vi "PAS RI Retrieval with LABVIEW.vi"() -> ()   [LabVIEW 2013]
uses:
  BaesDataTypeDefinition.ctl
  ReadBaesDataTypeDefinition.ctl
  ParticleDistributionData.ctl
  GeneralDataForRIRetrieval.ctl
  <vilib>/Native 3D Graph/xcontrol/3DPC_SurfacePlot.xctl
  <vilib>/Native 3D Graph/classes/Surface/Surface.lvclass
  RIandRIMCResults.ctl
  <vilib>/gmath/NumericalOptimization/stopping criteria.ctl
  <vilib>/Analysis/1siggen.llb/Ramp Pattern by Samples.vi
  <vilib>/gmath/NumericalOptimization/Conjugate Gradient.vi
  <vilib>/Utility/file.llb/Write To Spreadsheet File (string).vi
  <vilib>/Analysis/Matrix/Numeric/Conversions/Matrix To Array - RM.vi
  <vilib>/gmath/statdist.llb/Normal Inverse CDF.vi
  <vilib>/imath/engines/lvmath2/RunTimeEngine/ErrorHandling/NIMS_Finalize Error.vi
  <vilib>/imath/engines/lvmath2/RunTimeEngine/RangeToken/NIMS_Range_R2 - Float.vi
  <instcachedir>/0/NIMS_Range_R2 - Float_E19924E36A3948A4B33043226480F83C.lvgen/NIMS_Range_R2 - Float_E19924E36A3948A4B33043226480F83C_000.vi
  <vilib>/imath/engines/lvmath2/RunTimeEngine/NodeEndStatement/NIMS_NodeEndStatement_Output.vi
  <instcachedir>/0/NIMS_NodeEndStatement_Output_53EC0D466D134D7ABD903AC30B43404B.lvgen/NIMS_NodeEndStatement_Output_53EC0D466D134D7ABD903AC30B43404B_002.vi
  <vilib>/imath/engines/lvmath2/RunTimeEngine/CommandStatement/MC_CommandStatement_break.vi
  <vilib>/imath/engines/lvmath2/RunTimeSupport/NIMS_Error if Not Equal.vi
  <instcachedir>/0/NIMS_Error if Not Equal_902F5D2649E64F5087A1EF57C55C58AB.lvgen/NIMS_Error if Not Equal_902F5D2649E64F5087A1EF57C55C58AB_000.vi
  <vilib>/imath/engines/lvmath2/RunTimeEngine/IndexRead/NIMS M($,S).vi
  <instcachedir>/0/NIMS M($,S)_3E5749BBB62E49528D4765A77F1F6D98.lvgen/NIMS M($,S)_3E5749BBB62E49528D4765A77F1F6D98_000.vi
  <vilib>/imath/engines/lvmath2/RunTimeEngine/RowToken/NIMS_RowToken_M_CV.vi
  <instcachedir>/0/NIMS_RowToken_M_CV_4FFFB80A1A2C4A06BEF1E2564C6BAFA4.lvgen/NIMS_RowToken_M_CV_4FFFB80A1A2C4A06BEF1E2564C6BAFA4_000.vi
  <vilib>/imath/engines/lvmath2/RunTimeEngine/ErrorHandling/NIMS_Create Error From Enums.vi
  <vilib>/gmath/NI_Gmath.lvlib
  <vilib>/Analysis/Matrix/NI_Matrix.lvlib
  <vilib>/Analysis/NI_AALBase.lvlib
panel:
  in  "autoscale":bool
  in  "Correct SMPS sizes to selected Sizes":bool
  out "Peak Center":dbl[](array[numeric])=[215.23700286959917, 239.46777469280113, 266.53712087613405, 296.56972011152817, 329.9933867048781, 354.3213922159785, 380.24064147372457, 407.9273850466716, 436.86507564817134]
  in  "method":i32(ring)=3 items=["nearest", "linear", "spline", "cubic Hermite", "Lagrange"]
  out "yi out":dbl[][](array[numeric])=[[0.0, 0.0, 0.0, 0.0, 0.0, 0.0, 0.0, 0.0, 0.0], [0.0, 0.0, 0.0, 0.0, 0.0, 0.0, 0.0, 0.0, 0.0], [0.0, 0.0, 0.0, 0.0, 0.0, 0.0, 0.0, 0.0, 0.0], [0.0, 0.0, 0.0, 0.0, 0.0, 0.0, 0.0, 0.0, 0.0], [0.0, 0.0, 0.0, 0.0, 0.0, 0.0, 0.0, 0.0, 0.0], [0.0, 0.0, 0.0, 0.0, 0.0, 0.0, 0.0, 0.0, 0.0], [0.0, 0.0, 0.0, 0.0, 0.0, 0.0, 0.0, 0.0, 0.0], [0.0, 0.0, 0.0, 0.0, 0.0, 0.0, 0.0, 0.0, 0.0], [0.0, 0.0, 0.0, 0.0, 0.0, 0.0, 0.0, 0.0, 0.0], [0.0, 0.0, 0.0, 0.0, 0.0, 0.0, 0.0, 0.0, 0.0], [0.0, 0.0, 0.0, 0.0, 0.0, 0.0, 0.0, 0.0, 0.0], [0.0, 0.0, 0.0, 0.0, 0.0, 0.0, 0.0, 0.0, 0.0], [0.0, 0.0, 0.0, 0.0, 0.0, 0.0, 0.0, 0.0, 0.0], [0.0, 0.0, 0.0, 0.0, 0.0, 0.0, 0.0, 0.0, 0.0], [0.0, 0.0, 0.0, 0.0, 0.0, 0.0, 0.0, 0.0, 0.0], [0.0, 0.0, 0.0, 0.0, 0.0, 0.0, 0.0, 0.0, 0.0], [0.002995533043634161, 0.0, 0.0, 0.0, 0.0, 0.0, 0.0, 0.0, 0.0], [0.025840856539342556, 0.0, 0.0, 0.0, 0.0, 0.0, 0.0, 0.0, 0.0], [0.09627433030958367, 0.0, 0.0, 0.0, 0.0, 0.0, 0.0, 0.0, 0.0], [0.20114413818462407, 0.003679405258454903, 0.0, 0.0, 0.0, 0.0, 0.0, 0.0, 0.0], [0.24542760207823705, 0.030110785948579594, 0.0, 0.0, 0.0, 0.0, 0.0, 0.0, 0.0], [0.19935011876678227, 0.10676097365384078, 0.0, 0.0, 0.0, 0.0, 0.0, 0.0, 0.0], [0.10027077337218139, 0.21292413302969826, 0.0033748243651170722, 0.0, 0.0, 0.0, 0.0, 0.0, 0.0], [0.02900603131815543, 0.252436330373865, 0.02890039600275283, 0.0, 0.0, 0.0, 0.0, 0.0, 0.0], [0.0039798778324419744, 0.1962993842174311, 0.10425475468568692, 0.0, 0.0, 0.0, 0.0, 0.0, 0.0], [0.0, 0.09510810120556674, 0.2127509720448336, 0.003204303022032701, 0.0, 0.0, 0.0, 0.0, 0.0], [0.0, 0.026788275767934952, 0.25443516550640577, 0.028222420464123123, 0.0, 0.0, 0.0, 0.0, 0.0], [0.0, 0.0036138798422305257, 0.20572070395413536, 0.10336691645150534, 0.0, 0.0, 0.0, 0.0, 0.0], [0.0, 0.0, 0.10385751888143922, 0.21356874773842194, 0.003345015757771727, 0.0, 0.0, 0.0, 0.0], [0.0, 0.0, 0.03184137129301377, 0.25514474611865134, 0.02938228217938827, 0.0, 0.0, 0.0, 0.0], [0.0014956304497509467, 0.0, 0.005324689051489316, 0.21179320089555217, 0.10705199934528585, 0.003308736710887511, 0.0, 0.0, 0.0], [0.006181204689297098, 0.0, 0.0, 0.10947088728935564, 0.21880478513266646, 0.029404152563977024, 0.0, 0.0, 0.0], [0.014779079751943505, 0.0, 0.0, 0.0351443521735081, 0.2573967125709004, 0.10811744003531051, 0.004055473967709127, 0.0, 0.0], [0.021873123606276416, 0.0, 0.0, 0.00645421284142625, 0.21311979554910082, 0.21949012820871305, 0.03249660231234976, 0.0, 0.0], [0.020938671287516166, 0.002941447778294588, 0.0, 0.0005784696243201418, 0.11000745576713801, 0.2570127905092043, 0.11420156491259865, 0.004251138588627886, 0.0], [0.014150903231161319, 0.00918486371676828, 0.0, 0.0, 0.036185400505208645, 0.21598258772382448, 0.22683349675845424, 0.03241034304426709, 0.0], [0.005998151011193356, 0.016563944732687075, 0.0, 0.0, 0.007021566470141746, 0.11238428494392888, 0.25641274621663857, 0.11266793086437756, 0.004147715999403451], [0.0015120995486811858, 0.017797923247623602, 0.001492807625783663, 0.0, 0.0007094205616598339, 0.037396339870968194, 0.21111602466052512, 0.22428037538775147, 0.031085439808444255], [0.0, 0.01329593538708705, 0.005201029958243257, 0.0, 0.0, 0.007536234728094553, 0.10787117985635983, 0.25568882442612334, 0.11065902188610582], [0.0, 0.00635541490586478, 0.010415971194231972, 0.0, 0.0, 0.0008190951722994508, 0.03536648135652447, 0.21469636352155314, 0.2221123992215679], [0.0010729774499575713, 0.0019363898629268694, 0.01277891881575932, 0.0006807013617405569, 0.0, 0.0, 0.007025068509258474, 0.10969810395513567, 0.25508407775997943], [0.002057300309839938, 0.0, 0.010740838502774176, 0.002649342768284491, 0.0, 0.0, 0.0007440549395453882, 0.03615143628832095, 0.216785934587122], [0.002474950875894475, 0.0, 0.006120821318984597, 0.006052131853820764, 0.0, 0.0, 0.0, 0.007394514918229318, 0.11122539130067338], [0.002060729815382503, 0.0, 0.002286068305636173, 0.008519468407529212, 0.0, 0.0, 0.0, 0.0008550654797584019, 0.03853326504170029], [0.0011159165281229126, 0.0009250356514019637, 0.0005031484937129974, 0.007827186354841077, 0.0010483084611445424, 0.0, 0.0, 0.0, 0.008221211137071305], [0.0, 0.0013182032160797494, 0.0, 0.0048751624944381525, 0.002846930380238516, 0.0, 0.0, 0.0, 0.0009934611660537788], [0.0, 0.0011832812074649155, 0.0, 0.0019419202748162476, 0.004454066932151218, 0.0, 0.0, 0.0, 0.0], [0.0, 0.0007762909961994142, 0.0, 0.0005058298656327597, 0.004488441198541657, 0.001576949269729668, 0.0, 0.0, 0.0], [0.0, 0.0, 0.0, 0.0, 0.0029347814148206284, 0.002346089545272472, 0.0, 0.0, 0.0], [0.0, 0.0, 0.0, 0.0, 0.0012030377738417415, 0.00231674366991226, 0.0007291026037730795, 0.0, 0.0], [0.0, 0.0, 0.0, 0.0, 0.0, 0.0015886617028698508, 0.0011333656105798114, 0.0, 0.0], [0.0, 0.0, 0.0, 0.0, 0.0, 0.0007197653450079487, 0.0011589853888717718, 0.0, 0.0], [0.0, 0.0, 0.0, 0.0, 0.0, 0.0, 0.0008558529068117928, 0.0005237679257223164, 0.0], [0.0, 0.0, 0.0, 0.0, 0.0, 0.0, 0.0, 0.0007042968505584731, 0.0], [0.0, 0.0, 0.0, 0.0, 0.0, 0.0, 0.0, 0.000677838749574469, 0.0], [0.0, 0.0, 0.0, 0.0, 0.0, 0.0, 0.0, 0.0, 0.000518938219565122], [0.0, 0.0, 0.0, 0.0, 0.0, 0.0, 0.0, 0.0, 0.0006331438723132111]]
  out "SMPS":T1(graph)=[{"Ramp Pattern"=[105.5, 109.4, 113.4, 117.6, 121.9, 126.3, 131.0, 135.8, 140.7, 145.9, 151.2, 156.8, 162.5, 168.5, 174.7, 181.1, 187.7, 194.6, 201.7, 209.1, 216.7, 224.7, 232.9, 241.4, 250.3, 259.5, 269.0, 278.8, 289.0, 299.6, 310.6, 322.0, 333.8, 346.0, 358.7, 371.8, 385.4, 399.5, 414.2, 429.4, 445.1, 461.4, 478.3, 495.8, 514.0, 532.8, 552.3, 572.5, 593.5, 615.3, 637.8, 661.2, 685.4, 710.5, 736.5, 763.5, 791.5], "Extinction"=[0.0, 0.0, 0.0, 0.0, 0.0, 0.0, 0.0, 0.0, 0.0, 0.0, 0.0, 0.0, 0.0, 0.0, 0.0, 0.0, 0.0, 0.0, 0.0, 0.0, 0.0, 0.0, 0.0, 0.0, 0.0, 0.0, 0.0, 0.0, 0.0, 0.0, 0.0, 0.0, 0.0, 0.0, 0.0, 0.0, 0.004147715999403451, 0.031085439808444255, 0.11065902188610582, 0.2221123992215679, 0.25508407775997943, 0.216785934587122, 0.11122539130067338, 0.03853326504170029, 0.008221211137071305, 0.0009934611660537788, 0.0, 0.0, 0.0, 0.0, 0.0, 0.0, 0.0, 0.0, 0.0, 0.000518938219565122, 0.0006331438723132111]}, {"Ramp Pattern"=[105.5, 109.4, 113.4, 117.6, 121.9, 126.3, 131.0, 135.8, 140.7, 145.9, 151.2, 156.8, 162.5, 168.5, 174.7, 181.1, 187.7, 194.6, 201.7, 209.1, 216.7, 224.7, 232.9, 241.4, 250.3, 259.5, 269.0, 278.8, 289.0, 299.6, 310.6, 322.0, 333.8, 346.0, 358.7, 371.8, 385.4, 399.5, 414.2, 429.4, 445.1, 461.4, 478.3, 495.8, 514.0, 532.8, 552.3, 572.5, 593.5, 615.3, 637.8, 661.2, 685.4, 710.5, 736.5, 763.5, 791.5], "Extinction"=[0.0, 0.0, 0.0, 0.0, 0.0, 0.0, 0.0, 0.0, 0.0, 0.0, 0.0, 0.0, 0.0, 0.0, 0.0, 0.0, 0.0, 0.0, 0.0, 0.0, 0.0, 0.0, 0.0, 0.0, 0.0, 0.0, 0.0, 0.0, 0.0, 0.0, 0.0, 0.0, 0.0, 0.0, 0.0, 0.000717254, 0.0123831, 0.0638696, 0.166954, 0.256206, 0.250783, 0.158589, 0.0675111, 0.0180047, 0.00271755, 0.000182617, 0.0, 0.0, 0.0, 0.0, 0.0, 1.197e-05, 6.86901e-05, 0.000249565, 0.000468067, 0.00056712, 0.000716313]}]
  in  "ShiftSMPStoSizes":bool
  out "Size Distribution":T1(graph)=[{"Ramp Pattern"=[105.5, 109.4, 113.4, 117.6, 121.9, 126.3, 131.0, 135.8, 140.7, 145.9, 151.2, 156.8, 162.5, 168.5, 174.7, 181.1, 187.7, 194.6, 201.7, 209.1, 216.7, 224.7, 232.9, 241.4, 250.3, 259.5, 269.0, 278.8, 289.0, 299.6, 310.6, 322.0, 333.8, 346.0, 358.7, 371.8, 385.4, 399.5, 414.2, 429.4, 445.1, 461.4, 478.3, 495.8, 514.0, 532.8, 552.3, 572.5, 593.5, 615.3, 637.8, 661.2, 685.4, 710.5, 736.5, 763.5, 791.5], "Extinction"=[0.0, 0.0, 0.0, 0.0, 0.0, 0.0, 0.0, 0.0, 0.0, 0.0, 0.0, 0.0, 0.0, 0.0, 0.0, 0.0, 0.00469758, 0.0354227, 0.116984, 0.216414, 0.247187, 0.179631, 0.0803359, 0.0204142, 0.00221516, 0.0, 0.0, 0.0, 0.0, 0.000247208, 0.00208403, 0.00771025, 0.0165625, 0.0223051, 0.0201811, 0.012183, 0.00466618, 0.00104529, 0.000166113, 0.000427922, 0.00128502, 0.00219655, 0.00249145, 0.00187776, 0.00091843, 0.000292032, 5.29153e-05, 4.6626e-06, 0.0, 0.0, 0.0, 0.0, 0.0, 0.0, 0.0, 0.0, 0.0]}, {"Ramp Pattern"=[105.5, 109.4, 113.4, 117.6, 121.9, 126.3, 131.0, 135.8, 140.7, 145.9, 151.2, 156.8, 162.5, 168.5, 174.7, 181.1, 187.7, 194.6, 201.7, 209.1, 216.7, 224.7, 232.9, 241.4, 250.3, 259.5, 269.0, 278.8, 289.0, 299.6, 310.6, 322.0, 333.8, 346.0, 358.7, 371.8, 385.4, 399.5, 414.2, 429.4, 445.1, 461.4, 478.3, 495.8, 514.0, 532.8, 552.3, 572.5, 593.5, 615.3, 637.8, 661.2, 685.4, 710.5, 736.5, 763.5, 791.5], "Extinction"=[0.0, 0.0, 0.0, 0.0, 0.0, 0.0, 0.0, 0.0, 0.0, 0.0, 0.0, 0.0, 0.0, 0.0, 0.0, 0.0, 0.0, 0.0, 0.0, 0.00519856, 0.0384325, 0.123532, 0.224073, 0.253164, 0.179467, 0.0797032, 0.0202966, 0.00230883, 2.78494e-05, 0.0, 0.0, 0.0, 1.449e-05, 0.000603145, 0.00368011, 0.0104387, 0.0170704, 0.0177851, 0.0120367, 0.00534763, 0.0015055, 0.000251878, 0.000139253, 0.000474877, 0.00100593, 0.00133239, 0.00112993, 0.000690039, 0.000227701, 5.64159e-05, 7.13036e-06, 4.80125e-07, 0.0, 0.0, 0.0, 0.0, 0.0]}, {"Ramp Pattern"=[105.5, 109.4, 113.4, 117.6, 121.9, 126.3, 131.0, 135.8, 140.7, 145.9, 151.2, 156.8, 162.5, 168.5, 174.7, 181.1, 187.7, 194.6, 201.7, 209.1, 216.7, 224.7, 232.9, 241.4, 250.3, 259.5, 269.0, 278.8, 289.0, 299.6, 310.6, 322.0, 333.8, 346.0, 358.7, 371.8, 385.4, 399.5, 414.2, 429.4, 445.1, 461.4, 478.3, 495.8, 514.0, 532.8, 552.3, 572.5, 593.5, 615.3, 637.8, 661.2, 685.4, 710.5, 736.5, 763.5, 791.5], "Extinction"=[0.0, 0.0, 0.0, 0.0, 0.0, 0.0, 0.0, 0.0, 0.0, 0.0, 0.0, 0.0, 0.0, 0.0, 0.0, 0.0, 0.0, 0.0, 0.0, 0.0, 0.0, 0.0, 0.00571825, 0.0414768, 0.129134, 0.230099, 0.256094, 0.180426, 0.0808733, 0.0216409, 0.00294192, 0.000130313, 0.0, 0.0, 0.0, 0.0, 0.000309949, 0.00212484, 0.00641526, 0.0113124, 0.0128925, 0.00963301, 0.00497583, 0.00165198, 0.00031264, 4.70524e-05, 0.00012066, 0.000336979, 0.000449342, 0.00045116, 0.000267214, 0.000124042, 3.43184e-05, 6.32589e-06, 6.1806e-07, 0.0, 0.0]}, {"Ramp Pattern"=[105.5, 109.4, 113.4, 117.6, 121.9, 126.3, 131.0, 135.8, 140.7, 145.9, 151.2, 156.8, 162.5, 168.5, 174.7, 181.1, 187.7, 194.6, 201.7, 209.1, 216.7, 224.7, 232.9, 241.4, 250.3, 259.5, 269.0, 278.8, 289.0, 299.6, 310.6, 322.0, 333.8, 346.0, 358.7, 371.8, 385.4, 399.5, 414.2, 429.4, 445.1, 461.4, 478.3, 495.8, 514.0, 532.8, 552.3, 572.5, 593.5, 615.3, 637.8, 661.2, 685.4, 710.5, 736.5, 763.5, 791.5], "Extinction"=[0.0, 0.0, 0.0, 0.0, 0.0, 0.0, 0.0, 0.0, 0.0, 0.0, 0.0, 0.0, 0.0, 0.0, 0.0, 0.0, 0.0, 0.0, 0.0, 0.0, 0.0, 0.0, 0.0, 0.0, 0.0, 0.00632071, 0.0446845, 0.135704, 0.236113, 0.25755, 0.180077, 0.0805602, 0.0218917, 0.00313629, 0.000172749, 0.0, 0.0, 0.0, 0.0, 0.000146105, 0.00109424, 0.00357516, 0.00701794, 0.00877109, 0.00708357, 0.00381669, 0.00131952, 0.000297028, 3.13476e-05, 2.27371e-05, 6.57026e-05, 0.000128581, 0.000145168, 0.00012623, 8.554e-05, 3.72251e-05, 2.65028e-05]}, {"Ramp Pattern"=[105.5, 109.4, 113.4, 117.6, 121.9, 126.3, 131.0, 135.8, 140.7, 145.9, 151.2, 156.8, 162.5, 168.5, 174.7, 181.1, 187.7, 194.6, 201.7, 209.1, 216.7, 224.7, 232.9, 241.4, 250.3, 259.5, 269.0, 278.8, 289.0, 299.6, 310.6, 322.0, 333.8, 346.0, 358.7, 371.8, 385.4, 399.5, 414.2, 429.4, 445.1, 461.4, 478.3, 495.8, 514.0, 532.8, 552.3, 572.5, 593.5, 615.3, 637.8, 661.2, 685.4, 710.5, 736.5, 763.5, 791.5], "Extinction"=[0.0, 0.0, 0.0, 0.0, 0.0, 0.0, 0.0, 0.0, 0.0, 0.0, 0.0, 0.0, 0.0, 0.0, 0.0, 0.0, 0.0, 0.0, 0.0, 0.0, 0.0, 0.0, 0.0, 0.0, 0.0, 0.0, 0.0, 0.0, 0.00691542, 0.0475552, 0.141845, 0.242118, 0.259618, 0.178404, 0.0799987, 0.0221613, 0.00339671, 0.000219474, 0.0, 0.0, 0.0, 0.0, 2.69179e-05, 0.000353007, 0.00153723, 0.00346079, 0.0046555, 0.00430387, 0.00217813, 0.000845627, 0.000191511, 2.95911e-05, 4.40706e-06, 1.46487e-05, 4.0603e-05, 5.6006e-05, 7.02252e-05]}, {"Ramp Pattern"=[105.5, 109.4, 113.4, 117.6, 121.9, 126.3, 131.0, 135.8, 140.7, 145.9, 151.2, 156.8, 162.5, 168.5, 174.7, 181.1, 187.7, 194.6, 201.7, 209.1, 216.7, 224.7, 232.9, 241.4, 250.3, 259.5, 269.0, 278.8, 289.0, 299.6, 310.6, 322.0, 333.8, 346.0, 358.7, 371.8, 385.4, 399.5, 414.2, 429.4, 445.1, 461.4, 478.3, 495.8, 514.0, 532.8, 552.3, 572.5, 593.5, 615.3, 637.8, 661.2, 685.4, 710.5, 736.5, 763.5, 791.5], "Extinction"=[0.0, 0.0, 0.0, 0.0, 0.0, 0.0, 0.0, 0.0, 0.0, 0.0, 0.0, 0.0, 0.0, 0.0, 0.0, 0.0, 0.0, 0.0, 0.0, 0.0, 0.0, 0.0, 0.0, 0.0, 0.0, 0.0, 0.0, 0.0, 0.0, 0.0, 0.00736473, 0.0497393, 0.146587, 0.244445, 0.259093, 0.17829, 0.0792691, 0.0221239, 0.00350155, 0.000239507, 0.0, 0.0, 0.0, 0.0, 0.0, 0.000136757, 0.000762018, 0.00196813, 0.00242627, 0.00218637, 0.0012033, 0.000506553, 0.000129976, 2.46205e-05, 2.20754e-06, 0.0, 0.0]}, {"Ramp Pattern"=[105.5, 109.4, 113.4, 117.6, 121.9, 126.3, 131.0, 135.8, 140.7, 145.9, 151.2, 156.8, 162.5, 168.5, 174.7, 181.1, 187.7, 194.6, 201.7, 209.1, 216.7, 224.7, 232.9, 241.4, 250.3, 259.5, 269.0, 278.8, 289.0, 299.6, 310.6, 322.0, 333.8, 346.0, 358.7, 371.8, 385.4, 399.5, 414.2, 429.4, 445.1, 461.4, 478.3, 495.8, 514.0, 532.8, 552.3, 572.5, 593.5, 615.3, 637.8, 661.2, 685.4, 710.5, 736.5, 763.5, 791.5], "Extinction"=[0.0, 0.0, 0.0, 0.0, 0.0, 0.0, 0.0, 0.0, 0.0, 0.0, 0.0, 0.0, 0.0, 0.0, 0.0, 0.0, 0.0, 0.0, 0.0, 0.0, 0.0, 0.0, 0.0, 0.0, 0.0, 0.0, 0.0, 0.0, 0.0, 0.0, 0.0, 0.000111786, 0.00841072, 0.0527736, 0.151025, 0.248521, 0.257332, 0.174677, 0.0773732, 0.021334, 0.00336166, 0.000228943, 0.0, 0.0, 0.0, 0.0, 0.0, 7.68722e-05, 0.000371516, 0.000899449, 0.00118202, 0.00112913, 0.000682538, 0.000358916, 0.00012183, 2.28142e-05, 5.76992e-06]}, {"Ramp Pattern"=[105.5, 109.4, 113.4, 117.6, 121.9, 126.3, 131.0, 135.8, 140.7, 145.9, 151.2, 156.8, 162.5, 168.5, 174.7, 181.1, 187.7, 194.6, 201.7, 209.1, 216.7, 224.7, 232.9, 241.4, 250.3, 259.5, 269.0, 278.8, 289.0, 299.6, 310.6, 322.0, 333.8, 346.0, 358.7, 371.8, 385.4, 399.5, 414.2, 429.4, 445.1, 461.4, 478.3, 495.8, 514.0, 532.8, 552.3, 572.5, 593.5, 615.3, 637.8, 661.2, 685.4, 710.5, 736.5, 763.5, 791.5], "Extinction"=[0.0, 0.0, 0.0, 0.0, 0.0, 0.0, 0.0, 0.0, 0.0, 0.0, 0.0, 0.0, 0.0, 0.0, 0.0, 0.0, 0.0, 0.0, 0.0, 0.0, 0.0, 0.0, 0.0, 0.0, 0.0, 0.0, 0.0, 0.0, 0.0, 0.0, 0.0, 0.0, 0.0, 0.00034567, 0.00996877, 0.0572363, 0.156117, 0.250468, 0.256357, 0.169838, 0.0734243, 0.0196929, 0.00313418, 0.000220524, 0.0, 0.0, 0.0, 0.0, 0.0, 3.08466e-05, 0.000159988, 0.000411927, 0.000591209, 0.000742169, 0.000598205, 0.000349683, 0.000313284]}, {"Ramp Pattern"=[105.5, 109.4, 113.4, 117.6, 121.9, 126.3, 131.0, 135.8, 140.7, 145.9, 151.2, 156.8, 162.5, 168.5, 174.7, 181.1, 187.7, 194.6, 201.7, 209.1, 216.7, 224.7, 232.9, 241.4, 250.3, 259.5, 269.0, 278.8, 289.0, 299.6, 310.6, 322.0, 333.8, 346.0, 358.7, 371.8, 385.4, 399.5, 414.2, 429.4, 445.1, 461.4, 478.3, 495.8, 514.0, 532.8, 552.3, 572.5, 593.5, 615.3, 637.8, 661.2, 685.4, 710.5, 736.5, 763.5, 791.5], "Extinction"=[0.0, 0.0, 0.0, 0.0, 0.0, 0.0, 0.0, 0.0, 0.0, 0.0, 0.0, 0.0, 0.0, 0.0, 0.0, 0.0, 0.0, 0.0, 0.0, 0.0, 0.0, 0.0, 0.0, 0.0, 0.0, 0.0, 0.0, 0.0, 0.0, 0.0, 0.0, 0.0, 0.0, 0.0, 0.0, 0.000717254, 0.0123831, 0.0638696, 0.166954, 0.256206, 0.250783, 0.158589, 0.0675111, 0.0180047, 0.00271755, 0.000182617, 0.0, 0.0, 0.0, 0.0, 0.0, 1.197e-05, 6.86901e-05, 0.000249565, 0.000468067, 0.00056712, 0.000716313]}]
  out "Extinction Data per size":T1(graph)=[{"Ramp Pattern"=[365.01001, 365.56, 366.10001, 366.64999, 367.19, 367.73001, 368.26999, 368.81, 369.35001, 369.89001, 386.09, 386.60001, 387.10999, 387.62, 388.13, 388.63, 389.14001, 389.64999, 390.14999, 390.66, 391.16, 391.67001, 392.17001, 392.67999, 393.17999, 393.67999, 394.17999, 394.67999, 395.19, 395.69, 396.19, 396.69, 397.19, 397.69, 398.19, 398.69, 399.19, 399.67999, 400.17999, 400.67999, 401.17999, 401.67999, 402.17001, 402.67001, 403.17001, 403.66, 404.16, 404.66, 405.14999, 405.64999, 406.14999, 406.64001, 407.14001, 407.64001, 408.13, 408.63, 409.13, 409.62, 410.12, 410.62, 411.10999, 411.60999, 412.10001, 412.60001, 413.10001, 413.60001, 414.09, 414.59, 415.09, 415.59, 416.07999, 416.57999, 417.07999, 417.57999, 418.07999, 418.57999, 419.07999, 419.57999, 420.07999, 420.57999, 421.07999, 421.57999, 422.07999, 422.57999, 423.09, 423.59, 424.09, 424.60001], "Extinction"=[-2.8242922e-13, -9.5446372e-13, -9.5673914e-13, -2.1710713e-12, -3.0653965e-12, -3.5744682e-12, -2.7968654e-12, -2.494626e-12, -1.8658978e-12, -2.7078036e-12, 1.199962e-09, 1.2044283e-09, 1.1869159e-09, 1.1971283e-09, 1.1743045e-09, 1.1673239e-09, 1.1844579e-09, 1.1774074e-09, 1.1781032e-09, 1.1685674e-09, 1.1821694e-09, 1.1679153e-09, 1.1804325e-09, 1.1549264e-09, 1.1582446e-09, 1.1719666e-09, 1.1561709e-09, 1.1576946e-09, 1.1596397e-09, 1.1522512e-09, 1.1499967e-09, 1.1519218e-09, 1.1412127e-09, 1.136586e-09, 1.1347415e-09, 1.1384925e-09, 1.1290678e-09, 1.134521e-09, 1.125919e-09, 1.1187079e-09, 1.1216958e-09, 1.1213084e-09, 1.1191187e-09, 1.1248569e-09, 1.1156328e-09, 1.1128937e-09, 1.1153232e-09, 1.1142656e-09, 1.1032915e-09, 1.1037591e-09, 1.0994153e-09, 1.0982592e-09, 1.0898938e-09, 1.0945469e-09, 1.090964e-09, 1.0935359e-09, 1.0873367e-09, 1.0829221e-09, 1.0798286e-09, 1.0773584e-09, 1.0711578e-09, 1.0749976e-09, 1.0730125e-09, 1.0733134e-09, 1.0667034e-09, 1.0626963e-09, 1.0597497e-09, 1.0538669e-09, 1.056263e-09, 1.0531479e-09, 1.0517495e-09, 1.0454831e-09, 1.0547482e-09, 1.0485262e-09, 1.0436499e-09, 1.042629e-09, 1.0315969e-09, 1.0291459e-09, 1.0254163e-09, 1.0385639e-09, 1.0386701e-09, 1.0280848e-09, 1.0382387e-09, 1.0251714e-09, 1.0107518e-09, 1.0066801e-09, 1.0073331e-09, 1.0244581e-09]}, {"Ramp Pattern"=[365.01001, 365.01001, 365.01001, 365.56, 365.56, 365.56, 366.10001, 366.10001, 366.10001, 366.64999, 366.64999, 366.64999, 367.19, 367.19, 367.19, 367.73001, 367.73001, 367.73001, 368.26999, 368.26999, 368.26999, 368.81, 368.81, 368.81, 369.35001, 369.35001, 369.35001, 369.89001, 369.89001, 369.89001, 386.09, 386.09, 386.09, 386.60001, 386.60001, 386.60001, 387.10999, 387.10999, 387.10999, 387.62, 387.62, 387.62, 388.13, 388.13, 388.13, 388.63, 388.63, 388.63, 389.14001, 389.14001, 389.14001, 389.64999, 389.64999, 389.64999, 390.14999, 390.14999, 390.14999, 390.66, 390.66, 390.66, 391.16, 391.16, 391.16, 391.67001, 391.67001, 391.67001, 392.17001, 392.17001, 392.17001, 392.67999, 392.67999, 392.67999, 393.17999, 393.17999, 393.17999, 393.67999, 393.67999, 393.67999, 394.17999, 394.17999, 394.17999, 394.67999, 394.67999, 394.67999, 395.19, 395.19, 395.19, 395.69, 395.69, 395.69, 396.19, 396.19, 396.19, 396.69, 396.69, 396.69, 397.19, 397.19, 397.19, 397.69, 397.69, 397.69, 398.19, 398.19, 398.19, 398.69, 398.69, 398.69, 399.19, 399.19, 399.19, 399.67999, 399.67999, 399.67999, 400.17999, 400.17999, 400.17999, 400.67999, 400.67999, 400.67999, 401.17999, 401.17999, 401.17999, 401.67999, 401.67999, 401.67999, 402.17001, 402.17001, 402.17001, 402.67001, 402.67001, 402.67001, 403.17001, 403.17001, 403.17001, 403.66, 403.66, 403.66, 404.16, 404.16, 404.16, 404.66, 404.66, 404.66, 405.14999, 405.14999, 405.14999, 405.64999, 405.64999, 405.64999, 406.14999, 406.14999, 406.14999, 406.64001, 406.64001, 406.64001, 407.14001, 407.14001, 407.14001, 407.64001, 407.64001, 407.64001, 408.13, 408.13, 408.13, 408.63, 408.63, 408.63, 409.13, 409.13, 409.13, 409.62, 409.62, 409.62, 410.12, 410.12, 410.12, 410.62, 410.62, 410.62, 411.10999, 411.10999, 411.10999, 411.60999, 411.60999, 411.60999, 412.10001, 412.10001, 412.10001, 412.60001, 412.60001, 412.60001, 413.10001, 413.10001, 413.10001, 413.60001, 413.60001, 413.60001, 414.09, 414.09, 414.09, 414.59, 414.59, 414.59, 415.09, 415.09, 415.09, 415.59, 415.59, 415.59, 416.07999, 416.07999, 416.07999, 416.57999, 416.57999, 416.57999, 417.07999, 417.07999, 417.07999, 417.57999, 417.57999, 417.57999, 418.07999, 418.07999, 418.07999, 418.57999, 418.57999, 418.57999, 419.07999, 419.07999, 419.07999, 419.57999, 419.57999, 419.57999, 420.07999, 420.07999, 420.07999, 420.57999, 420.57999, 420.57999, 421.07999, 421.07999, 421.07999, 421.57999, 421.57999, 421.57999, 422.07999, 422.07999, 422.07999, 422.57999, 422.57999, 422.57999, 423.09, 423.09, 423.09, 423.59, 423.59, 423.59, 424.09, 424.09, 424.09, 424.60001, 424.60001, 424.60001], "Extinction"=[nan, 5.63555038e-12, -6.20040882e-12, nan, 4.42688488e-12, -6.33581232e-12, nan, 4.44172376e-12, -6.35520204e-12, nan, 3.1925879e-12, -7.5347305e-12, nan, 1.9136571e-12, -8.044450099999999e-12, nan, 1.7542992000000003e-12, -8.9032356e-12, nan, 2.3729171999999995e-12, -7.966648e-12, nan, 2.7093124e-12, -7.6985644e-12, nan, 4.4583185e-12, -8.1901141e-12, nan, 2.9758349000000003e-12, -8.3914421e-12, nan, 1.3537115500000002e-09, 1.04621245e-09, nan, 1.33050989e-09, 1.0783467100000001e-09, nan, 1.29980645e-09, 1.07402535e-09, nan, 1.30703543e-09, 1.0872211700000001e-09, nan, 1.263323188e-09, 1.085285812e-09, nan, 1.257682822e-09, 1.0769649780000001e-09, nan, 1.257997803e-09, 1.110917997e-09, nan, 1.258281811e-09, 1.0965329889999999e-09, nan, 1.249724367e-09, 1.106482033e-09, nan, 1.233311541e-09, 1.1038232590000001e-09, nan, 1.242856071e-09, 1.1214827290000002e-09, nan, 1.220968997e-09, 1.114861603e-09, nan, 1.237850674e-09, 1.123014326e-09, nan, 1.20776521e-09, 1.1020875899999999e-09, nan, 1.207318623e-09, 1.1091705769999999e-09, nan, 1.219534456e-09, 1.124398744e-09, nan, 1.206780784e-09, 1.105561016e-09, nan, 1.2016583529999999e-09, 1.113730847e-09, nan, 1.202722643e-09, 1.1165567570000001e-09, nan, 1.193639166e-09, 1.110863234e-09, nan, 1.190472677e-09, 1.1095207229999998e-09, nan, 1.192674486e-09, 1.1111691140000001e-09, nan, 1.1818626490000002e-09, 1.100562751e-09, nan, 1.1711783190000001e-09, 1.101993681e-09, nan, 1.171442972e-09, 1.0980400280000001e-09, nan, 1.1742146020000001e-09, 1.102770398e-09, nan, 1.1647996130000001e-09, 1.093335987e-09, nan, 1.1680687030000001e-09, 1.100973297e-09, nan, 1.158754071e-09, 1.0930839290000001e-09, nan, 1.150347064e-09, 1.0870687359999998e-09, nan, 1.153138513e-09, 1.0902530870000001e-09, nan, 1.1536706730000001e-09, 1.088946127e-09, nan, 1.152280031e-09, 1.085957369e-09, nan, 1.155661193e-09, 1.094052607e-09, nan, 1.147199119e-09, 1.0840664810000001e-09, nan, 1.145071783e-09, 1.080715617e-09, nan, 1.147246497e-09, 1.083399903e-09, nan, 1.143375044e-09, 1.0851561559999999e-09, nan, 1.1348594220000001e-09, 1.071723578e-09, nan, 1.135517436e-09, 1.072000764e-09, nan, 1.125704434e-09, 1.0731261660000001e-09, nan, 1.127667266e-09, 1.0688511340000001e-09, nan, 1.117893049e-09, 1.061894551e-09, nan, 1.126185515e-09, 1.062908285e-09, nan, 1.1200817459999999e-09, 1.061846254e-09, nan, 1.1247833070000001e-09, 1.062288493e-09, nan, 1.117086625e-09, 1.057586775e-09, nan, 1.11416822e-09, 1.0516759800000001e-09, nan, 1.111104457e-09, 1.048552743e-09, nan, 1.107725349e-09, 1.046991451e-09, nan, 1.104137273e-09, 1.038178327e-09, nan, 1.107764944e-09, 1.042230256e-09, nan, 1.106480232e-09, 1.039544768e-09, nan, 1.110412925e-09, 1.0362138749999999e-09, nan, 1.1036413210000002e-09, 1.029765479e-09, nan, 1.099794992e-09, 1.0255976079999999e-09, nan, 1.098809091e-09, 1.0206903090000001e-09, nan, 1.094440483e-09, 1.013293317e-09, nan, 1.09649886e-09, 1.01602714e-09, nan, 1.095379445e-09, 1.010916355e-09, nan, 1.095129175e-09, 1.008369825e-09, nan, 1.0888327469999999e-09, 1.002133453e-09, nan, 1.105700682e-09, 1.0037957179999999e-09, nan, 1.096226079e-09, 1.0008263209999998e-09, nan, 1.090656791e-09, 9.96643009e-10, nan, 1.096478637e-09, 9.88779363e-10, nan, 1.08555377e-09, 9.7764003e-10, nan, 1.0987320770000001e-09, 9.59559723e-10, nan, 1.099013116e-09, 9.51819484e-10, nan, 1.115469798e-09, 9.61658002e-10, nan, 1.121745799e-09, 9.55594401e-10, nan, 1.1148866849999999e-09, 9.41282915e-10, nan, 1.14595311e-09, 9.305242899999999e-10, nan, 1.13382451e-09, 9.165182899999999e-10, nan, 1.15459483e-09, 8.6690877e-10, nan, 1.14573256e-09, 8.676276399999999e-10, nan, 1.19507904e-09, 8.1958716e-10, nan, 1.2450424e-09, 8.038738e-10]}, ...(18 in all)]
  out "Wavelength":string="WL=390.660nm"
  out "Imaginary Part":string="k=0.048±0.000"
  out "Real Part":string="n=1.680±0.000"
  in  "Quick Fit":bool=TRUE
  in  "Diameters to fit":i32[](listbox)=[8]
  out "Residue":dbl=nan
  in  "ExtinctionOrAbsorptionOrScattering":i8(knob) scale=0.0..2.0
  in  "Plot RI":bool
  in  "k":dbl=0.042
  in  "n":dbl=1.668
  out "Residue (CDMRI)":dbl=0.5889105101545833
  out "Wavelength":dbl=390.66 format="%.3g"
  out "Imaginary Uncertainty":dbl caption="±" format="%.3g"
  out "Imaginary Part":dbl=0.047805814919599496 format="%.3g"
  out "Real Uncertainty":dbl caption="±" format="%.3g"
  out "Real part":dbl=1.6804005919533238 format="%.3g"
  out "Diameter Offset":dbl
  out "Diameter Factor":dbl=1.0
  out "Extinction Factor":dbl=1.0
  out "Residue (MDBF)":dbl=0.15189618824405976
  out "Time Left (min)":dbl=22.74556666666667 format="%#.1f"
  out "Progress bar for Extinction search":u8(slide)=12 max=5 scale=-1.0..51.0
  in  "Diameter Factor Radio Button":bool
  in  "Diamter Offset Radio Button":bool=TRUE
  in  "Diameter FO Interval":dbl=1.0 caption="Interval"
  in  "Diameter FO Finish":dbl=5.0 caption="Finish"
  in  "Diameter FO start":dbl=-5.0 caption="Start"
  in  "Diameter Offset":dbl
  in  "Diameter Factor":dbl=1.0
  in  "Extinction Factor":dbl=1.2
  in  "Extinction Factor Interval":dbl=0.1 caption="Interval"
  in  "Extinction Factor Finish":dbl=1.2 caption="Finish"
  in  "Extinction Factor Start":dbl=0.8 caption="Start"
  in  "Find Extinction Factor Graph":bool
  out "3D Graph":refnum<class "Base Datatype.lvclass">[](xcontrol)
  in  "Use Factors":bool
  in  "Min Wavelength":string(combo)="0"
  in  "Max Wavelength":string(combo)="87"
  in  "Restrict to Positive Imaginary Part":bool=TRUE
  in  "Calculate Errors":bool=TRUE
  in  "Approximate Errors":bool
  in  "Save RI":bool
  in  "Retrieve RI":bool
  in  "Mutiple Charge Data File":path=path "Pahokee Interpulated Multiply charge distribution.txt"
  in  "Extinction Cross Section File":path=path "Pahokee BAES 405 only data.txt"
  in  "Diameter Factor or Offset 2":bool=TRUE caption="Offset - True, Factor - OFF"
  out "Simplex":T2(graph)=[{"Size parameters"=[1.6529173641234718, 1.6528239047901785, 1.6528645104684014, 1.6529173641234718], "Normalized Residuals"=[0.039652080755025215, 0.03959684108062281, 0.03975145459202683, 0.039652080755025215]}]
  in  "Diameter Factor or Offset":bool=TRUE caption="Offset - True, Factor - OFF"
  in  "Minimization method":u16(ring)=1 items=["LM method", "Simplex Method"]
  in  "Extinction Factor in Data":dbl=1.0
  out "Residue Graph Matrix":dbl[][](array[numeric])=[[0.8817748876641518, 0.7943260267120898, 0.7221799384952265, 0.6683504995926692, 0.6311277469517097, 0.6088767086158524], [0.7307518731289654, 0.673042958848353, 0.6345421279928648, 0.6122901406297341, 0.6040701363961388, 0.6079500250191767], [0.6456146353159482, 0.6217239264490524, 0.6132715417472164, 0.6175167400813633, 0.6328117960393451, 0.6563665043893292], [0.6273068413741216, 0.6311010869376654, 0.6464620791865137, 0.671082182122829, 0.7034305368703453, 0.741845745993439], [0.6631237737749567, 0.6880232407171314, 0.7208560286150587, 0.7602689432195936, 0.8046376766720158, 0.8530494481747876]]
  out "Extinction Factor Results":cluster{dbl[], dbl[]}[](graph)=[{[0.8, 0.9, 1.0, 1.1, 1.2], [1.539671374334097, 1.5976213646223005, 1.5606320545412844, 1.5516397914476685, 1.5319499648100456]}, {[0.8, 0.9, 1.0, 1.1, 1.2], [-0.11096660801067405, -0.0653657766346238, -0.05966999471633491, -0.017727862931787984, 0.01906205546692944]}, {[0.8, 0.9, 1.0, 1.1, 1.2], [13.260187371616055, 8.444315776530917, 1.2615157523101117, 0.7276563123626676, 0.6329059597830448]}]
  in  "General Data for RI Retrieval VI":T3={"Min WaveLength Index"=0, "Max WaveLength Index"=0, "Extinction Factor"=FALSE, "Size Parameter Factor"=FALSE, "Size Paramter Offset"=FALSE, "Extinction Factor"=1.0, "Diameter Factor"=1.0, "Diameter Offset"=0.0, "ExtinctionOrAbsorptionOrScattering"=0} {"ExtinctionOrAbsorptionOrScattering" scale=0.0..2.0; "Max WaveLength Index" max=200 step=1; "Min WaveLength Index" max=200 step=1}
  in  "Graph Refs 2":T4
  in  "Size Parameter Offset":bool
  in  "Size Parameter Factor":bool
  in  "Extinction Factor":bool
  out "Minimized Size Parameter Factor":dbl
  out "Minimized Extinction Factor":dbl
  in  "Data for RIRetrieval VI":T7={"Approximate Errors"=FALSE, "Extinction ExtinctionUncertainity Size parameter and Number ofS sizes"={"Extinction"=[], "Extinction Uncertainty"=[], "Size parameters"=[], "Number ofSizes"=0.0, "GeometricCrossSection"=[], "WaveLength"=[], "Sizes"=[]}, "Minimization method"=0, "Graph Ref"={"Real Part vs wavelength"=refnum, "Imaginary Part vs wavelength"=refnum, "Normalized Residuals vs Size parameter"=refnum, "Not Corrected for Multiple charge particles"=refnum, "Simplex 2"=refnum}, "Particle Distribution Data"={"SMPS Sizes"=[], "Concentration"=[], "Double Charge Correction Flag"=FALSE}, "Calculate Errors"=FALSE, "Restrict to Positive Imaginary Part"=FALSE, "MinMaxWavelength"={0, 0, "Extinction Factor"=FALSE, "Size Parameter Factor"=FALSE, "Size Parameter Offset"=TRUE, "Extinction Factor"=1.0, "Diameter Factor"=1.0, "Diameter Offset"=0.0, "ExtinctionOrAbsorptionOrScattering"=0}} {"MinMaxWavelength"."ExtinctionOrAbsorptionOrScattering" scale=0.0..2.0}
  in  "Graph Refs":T4
  in  "Factor Ext Uncertainty in Data":dbl=1.0
  in  "Save RI expanded Edition":bool
  out "Saved RI to this filename and path 2":path=path "Z:/Dropbox/Lior Segev/Lior Segev Projects/RI retrieval in Labview/Data/Ammonium Sulfate/20130724ForMatlabRetrival-RIresult.xls"
  out "index of element":i32=19
  out "Corrected for multiple charge particles":cluster{"Size parameters":dbl[], dbl[]}[](graph)=[{"Size parameters"=[1.7450611934392695, 1.9380633530823226, 2.163232539332551, 2.4125269955381605, 2.6859467216991524, 2.886990637993999, 3.09607631094064, 3.3292872538426614, 3.5785817100482715], [8.613177599197425e-10, 1.2408352063925388e-09, 1.7995629510509214e-09, 2.6110235655556243e-09, 3.3534046199730396e-09, 3.98056940281271e-09, 4.73942328753743e-09, 5.206671970490486e-09, 5.5799340886387966e-09]}, {"Size parameters"=[1.7450611934392695, 1.9380633530823226, 2.163232539332551, 2.4125269955381605, 2.6859467216991524, 2.886990637993999, 3.09607631094064, 3.3292872538426614, 3.5785817100482715], [1.1685674e-09, 1.5291233e-09, 2.0086066e-09, 2.7468887e-09, 3.4171841e-09, 4.0104418e-09, 4.7531996e-09, 5.2183244e-09, 5.5894183e-09]}, {"Size parameters"=[1.3960489547514157, 1.4250314457244808, 1.4540139366975458, 1.482996427670611, 1.511978918643676, 1.5409614096167412, 1.5699439005898062, 1.5989263915628713, 1.6279088825359365, 1.6568913735090016, 1.6858738644820666, 1.7148563554551317, 1.7438388464281969, 1.772821337401262, 1.801803828374327, 1.830786319347392, 1.8597688103204573, 1.8887513012935222, 1.9177337922665874, 1.9467162832396525, 1.9756987742127177, 2.004681265185783, 2.0336637561588478, 2.0626462471319127, 2.091628738104978, 2.120611229078043, 2.1495937200511084, 2.1785762110241733, 2.2075587019972382, 2.2365411929703036, 2.2655236839433686, 2.2945061749164335, 2.323488665889499, 2.352471156862564, 2.3814536478356287, 2.410436138808694, 2.439418629781759, 2.4684011207548244, 2.4973836117278894, 2.5263661027009543, 2.5553485936740197, 2.5843310846470846, 2.6133135756201495, 2.642296066593215, 2.67127855756628, 2.7002610485393452, 2.72924353951241, 2.758226030485475, 2.7872085214585405, 2.8161910124316054, 2.8451735034046703, 2.8741559943777357, 2.9031384853508007, 2.9321209763238656, 2.961103467296931, 2.990085958269996, 3.0190684492430613, 3.048050940216126, 3.077033431189191, 3.1060159221622565, 3.1349984131353215, 3.1639809041083864, 3.1929633950814518, 3.2219458860545167, 3.2509283770275816, 3.279910868000647, 3.308893358973712, 3.3378758499467773, 3.3668583409198423, 3.395840831892907, 3.4248233228659726, 3.4538058138390375, 3.4827883048121024, 3.511770795785168, 3.5407532867582328, 3.569735777731298, 3.598718268704363, 3.627700759677428, 3.6566832506504934, 3.6856657416235583, 3.7146482325966232, 3.7436307235696886, 3.7726132145427536, 3.8015957055158185, 3.830578196488884, 3.859560687461949, 3.888543178435014, 3.917525669408079, 3.946508160381144, 3.9754906513542094, 4.004473142327274, 4.033455633300339, 4.062438124273404, 4.09142061524647, 4.120403106219535, 4.1493855971926, 4.178368088165665, 4.20735057913873, 4.236333070111795, 4.2653155610848605, 4.2942980520579255], [3.1999962634979153e-10, 3.5476346304213334e-10, 3.9297409960164114e-10, 4.348464251681627e-10, 4.804804480081233e-10, 5.298089185406747e-10, 5.825511045859248e-10, 6.381928416898762e-10, 6.959972412781217e-10, 7.550646131007389e-10, 8.144289325679342e-10, 8.73174810389267e-10, 9.305557061004217e-10, 9.860789069967023e-10, 1.0395500501967404e-09, 1.0910710868201193e-09, 1.1410067640159253e-09, 1.1899275067958656e-09, 1.2385516680813608e-09, 1.2876950434163523e-09, 1.3382312059776863e-09, 1.391065290024309e-09, 1.4471173475455016e-09, 1.507310847363849e-09, 1.5725600741818555e-09, 1.6437445321049892e-09, 1.7216747121318231e-09, 1.8070194543752458e-09, 1.900210458210982e-09, 2.0013167525924466e-09, 2.109895618329599e-09, 2.2248697109395706e-09, 2.344462150340603e-09, 2.466252492186942e-09, 2.5873851997038063e-09, 2.7049055770256327e-09, 2.8161613120843704e-09, 2.9191553389675797e-09, 3.0127531282085456e-09, 3.09672604490397e-09, 3.1716332294145293e-09, 3.2386261892168273e-09, 3.299240555572946e-09, 3.3552251437191067e-09, 3.40841709937649e-09, 3.4606762609485094e-09, 3.5138590255463857e-09, 3.5698107946301626e-09, 3.6303705800962336e-09, 3.6973624482112832e-09, 3.772569146145701e-09, 3.8576612175724505e-09, 3.954068463852589e-09, 4.06277923016077e-09, 4.184048013576186e-09, 4.317076317392021e-09, 4.459698434378452e-09, 4.608242797008923e-09, 4.7577153158902534e-09, 4.902363070370764e-09, 5.0365835613572695e-09, 5.155860085657124e-09, 5.257437494492346e-09, 5.340508015895134e-09, 5.405934475295575e-09, 5.455720742168624e-09, 5.492447378564924e-09, 5.518853121490812e-09, 5.5375841039278476e-09, 5.551121993046561e-09, 5.56180211169715e-09, 5.571892029601151e-09, 5.583689677574713e-09, 5.599604230808026e-09, 5.6221957666898505e-09, 5.654164537266654e-09, 5.698244779172477e-09, 5.756981317422774e-09, 5.832344164967521e-09, 5.925178997803131e-09, 6.034542221565242e-09, 6.157111230696494e-09, 6.286989272464443e-09, 6.416234563244409e-09, 6.536214327368349e-09, 6.639446139202945e-09, 6.72113437672997e-09, 6.7797496152719426e-09, 6.816543487712864e-09, 6.834422976414469e-09, 6.836812022362357e-09, 6.826891546266595e-09, 6.807286091219029e-09, 6.780098117090016e-09, 6.747143563591586e-09, 6.710211226649034e-09, 6.671306189359832e-09, 6.632820233667034e-09, 6.597636772444028e-09, 6.569129317569685e-09, 6.5511020585556446e-09]}, {"Size parameters"=[1.7450611934392695, 1.7450611934392695, 1.7450611934392695, 1.9380633530823226, 1.9380633530823226, 1.9380633530823226, 2.163232539332551, 2.163232539332551, 2.163232539332551, 2.4125269955381605, 2.4125269955381605, 2.4125269955381605, 2.6859467216991524, 2.6859467216991524, 2.6859467216991524, 2.886990637993999, 2.886990637993999, 2.886990637993999, 3.09607631094064, 3.09607631094064, 3.09607631094064, 3.3292872538426614, 3.3292872538426614, 3.3292872538426614, 3.5785817100482715, 3.5785817100482715, 3.5785817100482715], [nan, 9.260619009197425e-10, 7.965736189197425e-10, nan, 1.3049792433925387e-09, 1.1766911693925389e-09, nan, 1.8977598250509215e-09, 1.7013660770509214e-09, nan, 2.6999713035556244e-09, 2.522075827555624e-09, nan, 3.4569189599730397e-09, 3.2498902799730395e-09, nan, 4.1247233528127094e-09, 3.83641545281271e-09, nan, 4.94923861753743e-09, 4.52960795753743e-09, nan, 5.501231460490486e-09, 4.912112480490486e-09, nan, 6.0033378186387964e-09, 5.156530358638797e-09]}, {"Size parameters"=[1.7450611934392695, 1.9380633530823226, 2.163232539332551, 2.4125269955381605, 2.6859467216991524, 2.886990637993999, 3.09607631094064, 3.3292872538426614, 3.5785817100482715], [9.049410847944561e-10, 1.2643894773953952e-09, 1.7645799224496126e-09, 2.5917621135200773e-09, 3.380509474745812e-09, 3.910295403632372e-09, 4.65069705119374e-09, 5.312223094221181e-09, 5.726260863341419e-09]}]
  out "Multiple charge correction term":cluster{"Size parameters":dbl[], dbl[]}(graph)={"Size parameters"=[1.7450611934392695, 1.9380633530823226, 2.163232539332551, 2.4125269955381605, 2.6859467216991524, 2.886990637993999, 3.09607631094064, 3.3292872538426614, 3.5785817100482715], [3.905377336696676e-10, 3.798573320727451e-10, 3.0165907358137205e-10, 2.2409122852190442e-10, 1.2336343624910699e-10, 6.707843359850891e-11, 3.676768451675402e-11, 2.8300014180629405e-11, 2.1102074861523367e-11]}
  in  "Baes data type definition":T8={"Extinction"=[], "Extinction Uncertainty"=[], "Size parameters"=[], "Number ofSizes"=0.0, "GeometricCrossSection"=[], "Wave Length"=0.0, "SMPS Sizes"=[], "Concentration"=[], "Double Charge Correction"=FALSE, "Extincation Factor"=1.0, "Diameter Factor"=1.0, "Diameter Offset"=0.0, "Extinction Factor Flag"=FALSE, "Diameter Factor Flag"=FALSE, "Diameter Offset Flag"=FALSE, "Sizes"=[], "ExtinctionOrAbsorptionOrScattering"=0} {"ExtinctionOrAbsorptionOrScattering" scale=0.0..2.0}
  in  "Retrieve RI without taking the mean (MC)":bool
  out "Loop index (MC) 2":i32=4
  in  "Retrieve RI Calculate lines seperately":bool
  out "MC progress":u8(slide)=5 max=5 scale=-1.0..5.0
  in  "Save RI MC":bool
  out "Saved RI (MC) to this filename and path":path=path "Z:/Dropbox/Lior Segev/Lior Segev Projects/RI retrieval in Labview/Data/SyntheticData/SRFA_Spectrafit1-RI-MC-result.xls"
  out "Saved RI to this filename and path":path=path "Z:/Dropbox/Lior Segev/Lior Segev Projects/RI retrieval in Labview/Data/SyntheticData/PahokeeSynthetic/data/PahokeeFake4nd-ApproxError-Error-Restricted_RIresult.txt"
  out "Time Left (min) (MC)":dbl=0.0242 format="%#.1f"
  out "Loop index (MC)":i32=4
  out "Imaginary Part MC":cluster{dbl[], dbl[]}[](graph)=[{[414.59], [0.0008685207556328173]}, {[414.59, 414.59, 414.59], [nan, 0.004360832212642005, -0.0026237907013763706]}]
  out "Real Part MC":cluster{dbl[], dbl[]}[](graph)=[{[414.59], [1.5002369861550031]}, {[414.59, 414.59, 414.59], [nan, 1.5023737313826764, 1.4981002409273299]}]
  in  "Size of statistics":i32=5 min=0 max=150 step=1
  in  "Retrieve RI (MC)":bool
  out "Not Corrected for Multiple charge Best fit result":T1(graph)=[{"Ramp Pattern"=[1.7450611934392695, 1.9380633530823226, 2.163232539332551, 2.4125269955381605, 2.6859467216991524, 2.886990637993999, 3.09607631094064, 3.3292872538426614, 3.5785817100482715], "Extinction"=[1.1685674e-09, 1.5291233e-09, 2.0086066e-09, 2.7468887e-09, 3.4171841e-09, 4.0104418e-09, 4.7531996e-09, 5.2183244e-09, 5.5894183e-09]}, {"Ramp Pattern"=[1.7450611934392695, 1.7450611934392695, 1.7450611934392695, 1.9380633530823226, 1.9380633530823226, 1.9380633530823226, 2.163232539332551, 2.163232539332551, 2.163232539332551, 2.4125269955381605, 2.4125269955381605, 2.4125269955381605, 2.6859467216991524, 2.6859467216991524, 2.6859467216991524, 2.886990637993999, 2.886990637993999, 2.886990637993999, 3.09607631094064, 3.09607631094064, 3.09607631094064, 3.3292872538426614, 3.3292872538426614, 3.3292872538426614, 3.5785817100482715, 3.5785817100482715, 3.5785817100482715], "Extinction"=[nan, 1.233311541e-09, 1.1038232590000001e-09, nan, 1.593267337e-09, 1.464979263e-09, nan, 2.106803474e-09, 1.910409726e-09, nan, 2.835836438e-09, 2.6579409619999996e-09, nan, 3.52069844e-09, 3.31366976e-09, nan, 4.15459575e-09, 3.8662878500000004e-09, nan, 4.9630149300000005e-09, 4.54338427e-09, nan, 5.51288389e-09, 4.92376491e-09, nan, 6.01282203e-09, 5.16601457e-09]}, {"Ramp Pattern"=[1.7450611934392695, 1.9380633530823226, 2.163232539332551, 2.4125269955381605, 2.6859467216991524, 2.886990637993999, 3.09607631094064, 3.3292872538426614, 3.5785817100482715], "Extinction"=[1.2079723339471212e-09, 1.5509393252423484e-09, 1.975424020867661e-09, 2.728277970178248e-09, 3.4438075528296033e-09, 3.940824604885126e-09, 4.6649034931145616e-09, 5.323537873024072e-09, 5.7354406452365435e-09]}]
  out "Normalized Residuals vs Size parameter":T2(graph)=[{"Size parameters"=[1.7450611934392695, 1.9380633530823226, 2.163232539332551, 2.4125269955381605, 2.6859467216991524, 2.886990637993999, 3.09607631094064, 3.3292872538426614, 3.5785817100482715], "Normalized Residuals"=[0.608626327804295, 0.3401107561472616, -0.33791863310195897, -0.20923131372475734, 0.2571949106077552, -0.48293677994572304, -0.4208273316535878, 0.35718983226254, 0.34487713871341974]}]
  out "Imaginary Part vs wavelength":cluster{dbl[], dbl[]}[](graph)=[{[365.01001, 365.56, 366.10001, 366.64999, 367.19, 367.73001, 368.26999, 368.81, 369.35001, 369.89001, 386.09, 386.60001, 387.10999, 387.62, 388.13, 388.63, 389.14001, 389.64999, 390.14999, 390.66, 391.16, 391.67001, 392.17001, 392.67999, 393.17999, 393.67999, 394.17999, 394.67999, 395.19, 395.69, 396.19, 396.69, 397.19, 397.69, 398.19, 398.69, 399.19, 399.67999, 400.17999, 400.67999, 401.17999, 401.67999, 402.17001, 402.67001, 403.17001, 403.66, 404.16, 404.66, 405.14999, 405.64999, 406.14999, 406.64001, 407.14001, 407.64001, 408.13, 408.63, 409.13, 409.62, 410.12, 410.62, 411.10999, 411.60999, 412.10001, 412.60001, 413.10001, 413.60001, 414.09, 414.59, 415.09, 415.59, 416.07999, 416.57999, 417.07999, 417.57999, 418.07999, 418.57999, 419.07999, 419.57999, 420.07999, 420.57999, 421.07999, 421.57999, 422.07999, 422.57999, 423.09, 423.59, 424.09, 424.60001], [-0.00033967128569114874, -0.0005885819679670406, -0.004045485466519078, -0.007787172666459452, -0.010273410540921728, -0.012636447251879838, -0.014203342427545035, -0.014788763235872183, -0.015279677621325958, -0.019451191940988356, 1.9377636054690752, 1.8922317127548731, 1.7802834234994924, 1.8652250007083042, 1.781330597285123, 0.05102275361485863, 0.04521832768984223, 0.04362454178805547, 0.0464722123003294, 0.047805814919599496, 0.04677759938601142, 0.04224800457230871, 0.04738779810241525, 0.04765144934425466, 0.04319441664293394, 0.04957728225067244, 0.04772527598840229, 0.04522721714404457, 0.04732011417471499, 0.0418440339209947, 0.042329017316139514, 0.045291455752364575, 0.04577794951494711, 0.04251595291300604, 0.04289027951591111, 0.042649187845733696, 0.043880046819892465, 0.042528877982537835, 0.043035239168809386, 0.04002553847224323, 0.04215284466713188, 0.039676294770894904, 0.039982187325938, 0.041359394074522285, 0.04231557240155512, 0.04180514788239366, 0.041754018142080046, 0.03935683462694857, 0.03875834810622061, 0.03936000982752326, 0.03774662184996437, 0.039042223606538265, 0.035256500847335205, 0.03658445753871953, 0.035324768340087284, 0.03499068348955868, 0.03227828625876962, 0.032063578817141634, 0.03261090180192648, 0.02956018749446182, 0.0330706167389503, 0.0344585324293798, 0.03029226040754971, 0.028251680901120797, 0.02786034915046863, 0.02916685960637502, 0.028076637537327018, 0.02838302559767105, 0.026469497844466942, 0.030441641971359033, 0.027401275842406148, 0.02536729760742962, 0.028574402707584497, 0.02652712707915559, 0.025082738991316696, 0.0257647711438614, 0.023331552895672906, 0.023766312078062735, 0.021962693467342576, 0.023386105432712755, 0.028157361713077228, 0.019776304678801503, 0.019886804407272543, 0.014029367768947091, 0.02319401495884737, 0.014207610498691034, 0.020784388549203114, 0.039652080755025215]}, {[365.01001, 365.01001, 365.01001, 365.56, 365.56, 365.56, 366.10001, 366.10001, 366.10001, 366.64999, 366.64999, 366.64999, 367.19, 367.19, 367.19, 367.73001, 367.73001, 367.73001, 368.26999, 368.26999, 368.26999, 368.81, 368.81, 368.81, 369.35001, 369.35001, 369.35001, 369.89001, 369.89001, 369.89001, 386.09, 386.09, 386.09, 386.60001, 386.60001, 386.60001, 387.10999, 387.10999, 387.10999, 387.62, 387.62, 387.62, 388.13, 388.13, 388.13, 388.63, 388.63, 388.63, 389.14001, 389.14001, 389.14001, 389.64999, 389.64999, 389.64999, 390.14999, 390.14999, 390.14999, 390.66, 390.66, 390.66, 391.16, 391.16, 391.16, 391.67001, 391.67001, 391.67001, 392.17001, 392.17001, 392.17001, 392.67999, 392.67999, 392.67999, 393.17999, 393.17999, 393.17999, 393.67999, 393.67999, 393.67999, 394.17999, 394.17999, 394.17999, 394.67999, 394.67999, 394.67999, 395.19, 395.19, 395.19, 395.69, 395.69, 395.69, 396.19, 396.19, 396.19, 396.69, 396.69, 396.69, 397.19, 397.19, 397.19, 397.69, 397.69, 397.69, 398.19, 398.19, 398.19, 398.69, 398.69, 398.69, 399.19, 399.19, 399.19, 399.67999, 399.67999, 399.67999, 400.17999, 400.17999, 400.17999, 400.67999, 400.67999, 400.67999, 401.17999, 401.17999, 401.17999, 401.67999, 401.67999, 401.67999, 402.17001, 402.17001, 402.17001, 402.67001, 402.67001, 402.67001, 403.17001, 403.17001, 403.17001, 403.66, 403.66, 403.66, 404.16, 404.16, 404.16, 404.66, 404.66, 404.66, 405.14999, 405.14999, 405.14999, 405.64999, 405.64999, 405.64999, 406.14999, 406.14999, 406.14999, 406.64001, 406.64001, 406.64001, 407.14001, 407.14001, 407.14001, 407.64001, 407.64001, 407.64001, 408.13, 408.13, 408.13, 408.63, 408.63, 408.63, 409.13, 409.13, 409.13, 409.62, 409.62, 409.62, 410.12, 410.12, 410.12, 410.62, 410.62, 410.62, 411.10999, 411.10999, 411.10999, 411.60999, 411.60999, 411.60999, 412.10001, 412.10001, 412.10001, 412.60001, 412.60001, 412.60001, 413.10001, 413.10001, 413.10001, 413.60001, 413.60001, 413.60001, 414.09, 414.09, 414.09, 414.59, 414.59, 414.59, 415.09, 415.09, 415.09, 415.59, 415.59, 415.59, 416.07999, 416.07999, 416.07999, 416.57999, 416.57999, 416.57999, 417.07999, 417.07999, 417.07999, 417.57999, 417.57999, 417.57999, 418.07999, 418.07999, 418.07999, 418.57999, 418.57999, 418.57999, 419.07999, 419.07999, 419.07999, 419.57999, 419.57999, 419.57999, 420.07999, 420.07999, 420.07999, 420.57999, 420.57999, 420.57999, 421.07999, 421.07999, 421.07999, 421.57999, 421.57999, 421.57999, 422.07999, 422.07999, 422.07999, 422.57999, 422.57999, 422.57999, 423.09, 423.09, 423.09, 423.59, 423.59, 423.59, 424.09, 424.09, 424.09, 424.60001, 424.60001, 424.60001], [nan, -0.00033967128569114874, -0.00033967128569114874, nan, -0.0005885819679670406, -0.0005885819679670406, nan, -0.004045485466519078, -0.004045485466519078, nan, -0.007787172666459452, -0.007787172666459452, nan, -0.010273410540921728, -0.010273410540921728, nan, -0.012636447251879838, -0.012636447251879838, nan, -0.014203342427545035, -0.014203342427545035, nan, -0.014788763235872183, -0.014788763235872183, nan, -0.015279677621325958, -0.015279677621325958, nan, -0.019451191940988356, -0.019451191940988356, nan, 1.9377636054690752, 1.9377636054690752, nan, 1.8922317127548731, 1.8922317127548731, nan, 1.7802834234994924, 1.7802834234994924, nan, 1.8652250007083042, 1.8652250007083042, nan, 1.781330597285123, 1.781330597285123, nan, 0.05102275361485863, 0.05102275361485863, nan, 0.04521832768984223, 0.04521832768984223, nan, 0.04362454178805547, 0.04362454178805547, nan, 0.0464722123003294, 0.0464722123003294, nan, 0.047805814919599496, 0.047805814919599496, nan, 0.04677759938601142, 0.04677759938601142, nan, 0.04224800457230871, 0.04224800457230871, nan, 0.04738779810241525, 0.04738779810241525, nan, 0.04765144934425466, 0.04765144934425466, nan, 0.04319441664293394, 0.04319441664293394, nan, 0.04957728225067244, 0.04957728225067244, nan, 0.04772527598840229, 0.04772527598840229, nan, 0.04522721714404457, 0.04522721714404457, nan, 0.04732011417471499, 0.04732011417471499, nan, 0.0418440339209947, 0.0418440339209947, nan, 0.042329017316139514, 0.042329017316139514, nan, 0.045291455752364575, 0.045291455752364575, nan, 0.04577794951494711, 0.04577794951494711, nan, 0.04251595291300604, 0.04251595291300604, nan, 0.04289027951591111, 0.04289027951591111, nan, 0.042649187845733696, 0.042649187845733696, nan, 0.043880046819892465, 0.043880046819892465, nan, 0.042528877982537835, 0.042528877982537835, nan, 0.043035239168809386, 0.043035239168809386, nan, 0.04002553847224323, 0.04002553847224323, nan, 0.04215284466713188, 0.04215284466713188, nan, 0.039676294770894904, 0.039676294770894904, nan, 0.039982187325938, 0.039982187325938, nan, 0.041359394074522285, 0.041359394074522285, nan, 0.04231557240155512, 0.04231557240155512, nan, 0.04180514788239366, 0.04180514788239366, nan, 0.041754018142080046, 0.041754018142080046, nan, 0.03935683462694857, 0.03935683462694857, nan, 0.03875834810622061, 0.03875834810622061, nan, 0.03936000982752326, 0.03936000982752326, nan, 0.03774662184996437, 0.03774662184996437, nan, 0.039042223606538265, 0.039042223606538265, nan, 0.035256500847335205, 0.035256500847335205, nan, 0.03658445753871953, 0.03658445753871953, nan, 0.035324768340087284, 0.035324768340087284, nan, 0.03499068348955868, 0.03499068348955868, nan, 0.03227828625876962, 0.03227828625876962, nan, 0.032063578817141634, 0.032063578817141634, nan, 0.03261090180192648, 0.03261090180192648, nan, 0.02956018749446182, 0.02956018749446182, nan, 0.0330706167389503, 0.0330706167389503, nan, 0.0344585324293798, 0.0344585324293798, nan, 0.03029226040754971, 0.03029226040754971, nan, 0.028251680901120797, 0.028251680901120797, nan, 0.02786034915046863, 0.02786034915046863, nan, 0.02916685960637502, 0.02916685960637502, nan, 0.028076637537327018, 0.028076637537327018, nan, 0.02838302559767105, 0.02838302559767105, nan, 0.026469497844466942, 0.026469497844466942, nan, 0.030441641971359033, 0.030441641971359033, nan, 0.027401275842406148, 0.027401275842406148, nan, 0.02536729760742962, 0.02536729760742962, nan, 0.028574402707584497, 0.028574402707584497, nan, 0.02652712707915559, 0.02652712707915559, nan, 0.025082738991316696, 0.025082738991316696, nan, 0.0257647711438614, 0.0257647711438614, nan, 0.023331552895672906, 0.023331552895672906, nan, 0.023766312078062735, 0.023766312078062735, nan, 0.021962693467342576, 0.021962693467342576, nan, 0.023386105432712755, 0.023386105432712755, nan, 0.028157361713077228, 0.028157361713077228, nan, 0.019776304678801503, 0.019776304678801503, nan, 0.019886804407272543, 0.019886804407272543, nan, 0.014029367768947091, 0.014029367768947091, nan, 0.02319401495884737, 0.02319401495884737, nan, 0.014207610498691034, 0.014207610498691034, nan, 0.020784388549203114, 0.020784388549203114, nan, 0.039652080755025215, 0.039652080755025215]}, {[365.01001, 365.56, 366.10001, 366.64999, 367.19, 367.73001, 368.26999, 386.09, 388.63, 389.14001, 389.64999, 390.14999, 390.66, 391.16, 391.67001, 392.17001, 392.67999, 393.17999, 393.67999, 394.17999, 394.67999, 395.19, 395.69, 396.19, 396.69, 397.19, 397.69, 398.19, 398.69, 399.19, 399.67999, 400.17999, 400.67999, 401.17999, 401.67999, 402.17001, 402.67001, 403.17001, 403.66, 404.16, 404.66, 405.14999, 405.64999, 406.14999, 406.64001, 407.14001, 407.64001, 408.13, 408.63, 409.13, 409.62, 410.12, 410.62, 411.10999, 411.60999, 412.10001, 412.60001, 413.10001, 413.60001, 414.09, 414.59, 415.09, 415.59, 416.07999, 416.57999, 417.07999, 417.57999, 418.07999, 418.57999, 419.07999, 419.57999, 420.07999, 420.57999, 421.07999, 421.57999, 422.07999, 422.57999, 423.09, 423.59, 424.09, 424.60001], [-0.00033967128569114874, -0.0005885819679670406, -0.004045485466519078, -0.007787172666459452, -0.010273410540921728, -0.012636447251879838, -0.014203342427545035, 1.9377636054690752, 0.05102275361485863, 0.04521832768984223, 0.04362454178805547, 0.0464722123003294, 0.047805814919599496, 0.04677759938601142, 0.04224800457230871, 0.04738779810241525, 0.04765144934425466, 0.04319441664293394, 0.04957728225067244, 0.04772527598840229, 0.04522721714404457, 0.04732011417471499, 0.0418440339209947, 0.042329017316139514, 0.045291455752364575, 0.04577794951494711, 0.04251595291300604, 0.04289027951591111, 0.042649187845733696, 0.043880046819892465, 0.042528877982537835, 0.043035239168809386, 0.04002553847224323, 0.04215284466713188, 0.039676294770894904, 0.039982187325938, 0.041359394074522285, 0.04231557240155512, 0.04180514788239366, 0.041754018142080046, 0.03935683462694857, 0.03875834810622061, 0.03936000982752326, 0.03774662184996437, 0.039042223606538265, 0.035256500847335205, 0.03658445753871953, 0.035324768340087284, 0.03499068348955868, 0.03227828625876962, 0.032063578817141634, 0.03261090180192648, 0.02956018749446182, 0.0330706167389503, 0.0344585324293798, 0.03029226040754971, 0.028251680901120797, 0.02786034915046863, 0.02916685960637502, 0.028076637537327018, 0.02838302559767105, 0.026469497844466942, 0.030441641971359033, 0.027401275842406148, 0.02536729760742962, 0.028574402707584497, 0.02652712707915559, 0.025082738991316696, 0.0257647711438614, 0.023331552895672906, 0.023766312078062735, 0.021962693467342576, 0.023386105432712755, 0.028157361713077228, 0.019776304678801503, 0.019886804407272543, 0.014029367768947091, 0.02319401495884737, 0.014207610498691034, 0.020784388549203114, 0.039652080755025215]}]
  out "Real Part vs wavelength":cluster{dbl[], dbl[]}[](graph)=[{[365.01001, 365.56, 366.10001, 366.64999, 367.19, 367.73001, 368.26999, 368.81, 369.35001, 369.89001, 386.09, 386.60001, 387.10999, 387.62, 388.13, 388.63, 389.14001, 389.64999, 390.14999, 390.66, 391.16, 391.67001, 392.17001, 392.67999, 393.17999, 393.67999, 394.17999, 394.67999, 395.19, 395.69, 396.19, 396.69, 397.19, 397.69, 398.19, 398.69, 399.19, 399.67999, 400.17999, 400.67999, 401.17999, 401.67999, 402.17001, 402.67001, 403.17001, 403.66, 404.16, 404.66, 405.14999, 405.64999, 406.14999, 406.64001, 407.14001, 407.64001, 408.13, 408.63, 409.13, 409.62, 410.12, 410.62, 411.10999, 411.60999, 412.10001, 412.60001, 413.10001, 413.60001, 414.09, 414.59, 415.09, 415.59, 416.07999, 416.57999, 417.07999, 417.57999, 418.07999, 418.57999, 419.07999, 419.57999, 420.07999, 420.57999, 421.07999, 421.57999, 422.07999, 422.57999, 423.09, 423.59, 424.09, 424.60001], [0.999925365118786, 1.0190598908220525, 1.0517474408399405, 1.070226831916862, 1.0807585065879068, 1.0904326142267635, 1.095167348462244, 1.0979234786261842, 1.1010601073384612, 0.8890575035735264, 0.6747447069818042, 0.6887526383034903, 0.7286695747717085, 0.6939504883286365, 0.730608750980982, 1.6782732188226817, 1.6769673521341915, 1.6770787382722059, 1.6783646720126428, 1.6804005919533238, 1.685791602444036, 1.675628031256086, 1.6826531577729051, 1.674911014996645, 1.6733864728788044, 1.6842972401956229, 1.6775167121719587, 1.675427161602305, 1.6789051975809293, 1.6743027817212304, 1.6746538482838103, 1.677146503389699, 1.674751663938982, 1.67093405405048, 1.6718055158829102, 1.672660334062415, 1.6715018690644086, 1.6711893815205567, 1.6700324291440796, 1.6663407370828232, 1.6691308645638077, 1.6692037435343396, 1.6713015508746634, 1.671930356514817, 1.6684320504092047, 1.668142609581877, 1.6714414415900265, 1.6704097708706414, 1.6673772432670162, 1.6677956280930597, 1.664962214943713, 1.6675629567288492, 1.6635820804586334, 1.6667011500945015, 1.6656713141888553, 1.6656123484777143, 1.6627670101554923, 1.6637836822600893, 1.663822873580628, 1.6619636450255146, 1.6627326406830778, 1.664309531796151, 1.663455726105147, 1.6618534261792761, 1.6607123307148672, 1.6614120890955189, 1.6598688087633238, 1.660216551263631, 1.66033167860359, 1.6605317404016855, 1.661789139705553, 1.6588856641676568, 1.661599843921914, 1.6598728546880481, 1.6584018727772238, 1.6599920269016475, 1.6582284019057008, 1.6568187774353036, 1.6564199187917015, 1.6616388085049885, 1.6591526882428052, 1.657456927173964, 1.6615038704361833, 1.6558845801886244, 1.652472276673846, 1.6526949653590173, 1.6462338357979507, 1.6529173641234718]}, {[365.01001, 365.01001, 365.01001, 365.56, 365.56, 365.56, 366.10001, 366.10001, 366.10001, 366.64999, 366.64999, 366.64999, 367.19, 367.19, 367.19, 367.73001, 367.73001, 367.73001, 368.26999, 368.26999, 368.26999, 368.81, 368.81, 368.81, 369.35001, 369.35001, 369.35001, 369.89001, 369.89001, 369.89001, 386.09, 386.09, 386.09, 386.60001, 386.60001, 386.60001, 387.10999, 387.10999, 387.10999, 387.62, 387.62, 387.62, 388.13, 388.13, 388.13, 388.63, 388.63, 388.63, 389.14001, 389.14001, 389.14001, 389.64999, 389.64999, 389.64999, 390.14999, 390.14999, 390.14999, 390.66, 390.66, 390.66, 391.16, 391.16, 391.16, 391.67001, 391.67001, 391.67001, 392.17001, 392.17001, 392.17001, 392.67999, 392.67999, 392.67999, 393.17999, 393.17999, 393.17999, 393.67999, 393.67999, 393.67999, 394.17999, 394.17999, 394.17999, 394.67999, 394.67999, 394.67999, 395.19, 395.19, 395.19, 395.69, 395.69, 395.69, 396.19, 396.19, 396.19, 396.69, 396.69, 396.69, 397.19, 397.19, 397.19, 397.69, 397.69, 397.69, 398.19, 398.19, 398.19, 398.69, 398.69, 398.69, 399.19, 399.19, 399.19, 399.67999, 399.67999, 399.67999, 400.17999, 400.17999, 400.17999, 400.67999, 400.67999, 400.67999, 401.17999, 401.17999, 401.17999, 401.67999, 401.67999, 401.67999, 402.17001, 402.17001, 402.17001, 402.67001, 402.67001, 402.67001, 403.17001, 403.17001, 403.17001, 403.66, 403.66, 403.66, 404.16, 404.16, 404.16, 404.66, 404.66, 404.66, 405.14999, 405.14999, 405.14999, 405.64999, 405.64999, 405.64999, 406.14999, 406.14999, 406.14999, 406.64001, 406.64001, 406.64001, 407.14001, 407.14001, 407.14001, 407.64001, 407.64001, 407.64001, 408.13, 408.13, 408.13, 408.63, 408.63, 408.63, 409.13, 409.13, 409.13, 409.62, 409.62, 409.62, 410.12, 410.12, 410.12, 410.62, 410.62, 410.62, 411.10999, 411.10999, 411.10999, 411.60999, 411.60999, 411.60999, 412.10001, 412.10001, 412.10001, 412.60001, 412.60001, 412.60001, 413.10001, 413.10001, 413.10001, 413.60001, 413.60001, 413.60001, 414.09, 414.09, 414.09, 414.59, 414.59, 414.59, 415.09, 415.09, 415.09, 415.59, 415.59, 415.59, 416.07999, 416.07999, 416.07999, 416.57999, 416.57999, 416.57999, 417.07999, 417.07999, 417.07999, 417.57999, 417.57999, 417.57999, 418.07999, 418.07999, 418.07999, 418.57999, 418.57999, 418.57999, 419.07999, 419.07999, 419.07999, 419.57999, 419.57999, 419.57999, 420.07999, 420.07999, 420.07999, 420.57999, 420.57999, 420.57999, 421.07999, 421.07999, 421.07999, 421.57999, 421.57999, 421.57999, 422.07999, 422.07999, 422.07999, 422.57999, 422.57999, 422.57999, 423.09, 423.09, 423.09, 423.59, 423.59, 423.59, 424.09, 424.09, 424.09, 424.60001, 424.60001, 424.60001], [nan, 0.999925365118786, 0.999925365118786, nan, 1.0190598908220525, 1.0190598908220525, nan, 1.0517474408399405, 1.0517474408399405, nan, 1.070226831916862, 1.070226831916862, nan, 1.0807585065879068, 1.0807585065879068, nan, 1.0904326142267635, 1.0904326142267635, nan, 1.095167348462244, 1.095167348462244, nan, 1.0979234786261842, 1.0979234786261842, nan, 1.1010601073384612, 1.1010601073384612, nan, 0.8890575035735264, 0.8890575035735264, nan, 0.6747447069818042, 0.6747447069818042, nan, 0.6887526383034903, 0.6887526383034903, nan, 0.7286695747717085, 0.7286695747717085, nan, 0.6939504883286365, 0.6939504883286365, nan, 0.730608750980982, 0.730608750980982, nan, 1.6782732188226817, 1.6782732188226817, nan, 1.6769673521341915, 1.6769673521341915, nan, 1.6770787382722059, 1.6770787382722059, nan, 1.6783646720126428, 1.6783646720126428, nan, 1.6804005919533238, 1.6804005919533238, nan, 1.685791602444036, 1.685791602444036, nan, 1.675628031256086, 1.675628031256086, nan, 1.6826531577729051, 1.6826531577729051, nan, 1.674911014996645, 1.674911014996645, nan, 1.6733864728788044, 1.6733864728788044, nan, 1.6842972401956229, 1.6842972401956229, nan, 1.6775167121719587, 1.6775167121719587, nan, 1.675427161602305, 1.675427161602305, nan, 1.6789051975809293, 1.6789051975809293, nan, 1.6743027817212304, 1.6743027817212304, nan, 1.6746538482838103, 1.6746538482838103, nan, 1.677146503389699, 1.677146503389699, nan, 1.674751663938982, 1.674751663938982, nan, 1.67093405405048, 1.67093405405048, nan, 1.6718055158829102, 1.6718055158829102, nan, 1.672660334062415, 1.672660334062415, nan, 1.6715018690644086, 1.6715018690644086, nan, 1.6711893815205567, 1.6711893815205567, nan, 1.6700324291440796, 1.6700324291440796, nan, 1.6663407370828232, 1.6663407370828232, nan, 1.6691308645638077, 1.6691308645638077, nan, 1.6692037435343396, 1.6692037435343396, nan, 1.6713015508746634, 1.6713015508746634, nan, 1.671930356514817, 1.671930356514817, nan, 1.6684320504092047, 1.6684320504092047, nan, 1.668142609581877, 1.668142609581877, nan, 1.6714414415900265, 1.6714414415900265, nan, 1.6704097708706414, 1.6704097708706414, nan, 1.6673772432670162, 1.6673772432670162, nan, 1.6677956280930597, 1.6677956280930597, nan, 1.664962214943713, 1.664962214943713, nan, 1.6675629567288492, 1.6675629567288492, nan, 1.6635820804586334, 1.6635820804586334, nan, 1.6667011500945015, 1.6667011500945015, nan, 1.6656713141888553, 1.6656713141888553, nan, 1.6656123484777143, 1.6656123484777143, nan, 1.6627670101554923, 1.6627670101554923, nan, 1.6637836822600893, 1.6637836822600893, nan, 1.663822873580628, 1.663822873580628, nan, 1.6619636450255146, 1.6619636450255146, nan, 1.6627326406830778, 1.6627326406830778, nan, 1.664309531796151, 1.664309531796151, nan, 1.663455726105147, 1.663455726105147, nan, 1.6618534261792761, 1.6618534261792761, nan, 1.6607123307148672, 1.6607123307148672, nan, 1.6614120890955189, 1.6614120890955189, nan, 1.6598688087633238, 1.6598688087633238, nan, 1.660216551263631, 1.660216551263631, nan, 1.66033167860359, 1.66033167860359, nan, 1.6605317404016855, 1.6605317404016855, nan, 1.661789139705553, 1.661789139705553, nan, 1.6588856641676568, 1.6588856641676568, nan, 1.661599843921914, 1.661599843921914, nan, 1.6598728546880481, 1.6598728546880481, nan, 1.6584018727772238, 1.6584018727772238, nan, 1.6599920269016475, 1.6599920269016475, nan, 1.6582284019057008, 1.6582284019057008, nan, 1.6568187774353036, 1.6568187774353036, nan, 1.6564199187917015, 1.6564199187917015, nan, 1.6616388085049885, 1.6616388085049885, nan, 1.6591526882428052, 1.6591526882428052, nan, 1.657456927173964, 1.657456927173964, nan, 1.6615038704361833, 1.6615038704361833, nan, 1.6558845801886244, 1.6558845801886244, nan, 1.652472276673846, 1.652472276673846, nan, 1.6526949653590173, 1.6526949653590173, nan, 1.6462338357979507, 1.6462338357979507, nan, 1.6529173641234718, 1.6529173641234718]}, {[365.01001, 365.56, 366.10001, 366.64999, 367.19, 367.73001, 368.26999, 386.09, 388.63, 389.14001, 389.64999, 390.14999, 390.66, 391.16, 391.67001, 392.17001, 392.67999, 393.17999, 393.67999, 394.17999, 394.67999, 395.19, 395.69, 396.19, 396.69, 397.19, 397.69, 398.19, 398.69, 399.19, 399.67999, 400.17999, 400.67999, 401.17999, 401.67999, 402.17001, 402.67001, 403.17001, 403.66, 404.16, 404.66, 405.14999, 405.64999, 406.14999, 406.64001, 407.14001, 407.64001, 408.13, 408.63, 409.13, 409.62, 410.12, 410.62, 411.10999, 411.60999, 412.10001, 412.60001, 413.10001, 413.60001, 414.09, 414.59, 415.09, 415.59, 416.07999, 416.57999, 417.07999, 417.57999, 418.07999, 418.57999, 419.07999, 419.57999, 420.07999, 420.57999, 421.07999, 421.57999, 422.07999, 422.57999, 423.09, 423.59, 424.09, 424.60001], [0.999925365118786, 1.0190598908220525, 1.0517474408399405, 1.070226831916862, 1.0807585065879068, 1.0904326142267635, 1.095167348462244, 0.6747447069818042, 1.6782732188226817, 1.6769673521341915, 1.6770787382722059, 1.6783646720126428, 1.6804005919533238, 1.685791602444036, 1.675628031256086, 1.6826531577729051, 1.674911014996645, 1.6733864728788044, 1.6842972401956229, 1.6775167121719587, 1.675427161602305, 1.6789051975809293, 1.6743027817212304, 1.6746538482838103, 1.677146503389699, 1.674751663938982, 1.67093405405048, 1.6718055158829102, 1.672660334062415, 1.6715018690644086, 1.6711893815205567, 1.6700324291440796, 1.6663407370828232, 1.6691308645638077, 1.6692037435343396, 1.6713015508746634, 1.671930356514817, 1.6684320504092047, 1.668142609581877, 1.6714414415900265, 1.6704097708706414, 1.6673772432670162, 1.6677956280930597, 1.664962214943713, 1.6675629567288492, 1.6635820804586334, 1.6667011500945015, 1.6656713141888553, 1.6656123484777143, 1.6627670101554923, 1.6637836822600893, 1.663822873580628, 1.6619636450255146, 1.6627326406830778, 1.664309531796151, 1.663455726105147, 1.6618534261792761, 1.6607123307148672, 1.6614120890955189, 1.6598688087633238, 1.660216551263631, 1.66033167860359, 1.6605317404016855, 1.661789139705553, 1.6588856641676568, 1.661599843921914, 1.6598728546880481, 1.6584018727772238, 1.6599920269016475, 1.6582284019057008, 1.6568187774353036, 1.6564199187917015, 1.6616388085049885, 1.6591526882428052, 1.657456927173964, 1.6615038704361833, 1.6558845801886244, 1.652472276673846, 1.6526949653590173, 1.6462338357979507, 1.6529173641234718]}]
  in  "OK":bool
  # "Finding Factors is performed on only a single wavelength"
  # "Developed by Lior Segev\nsegev.lior@gmail.com\nYinon Rudich's Group\nDepartment of Earth and Planetary Sciences\n09 Dec 2013\nVer 1.0"
  # "Factors that minimize \nthe residue"
  # "Extinction Factor"
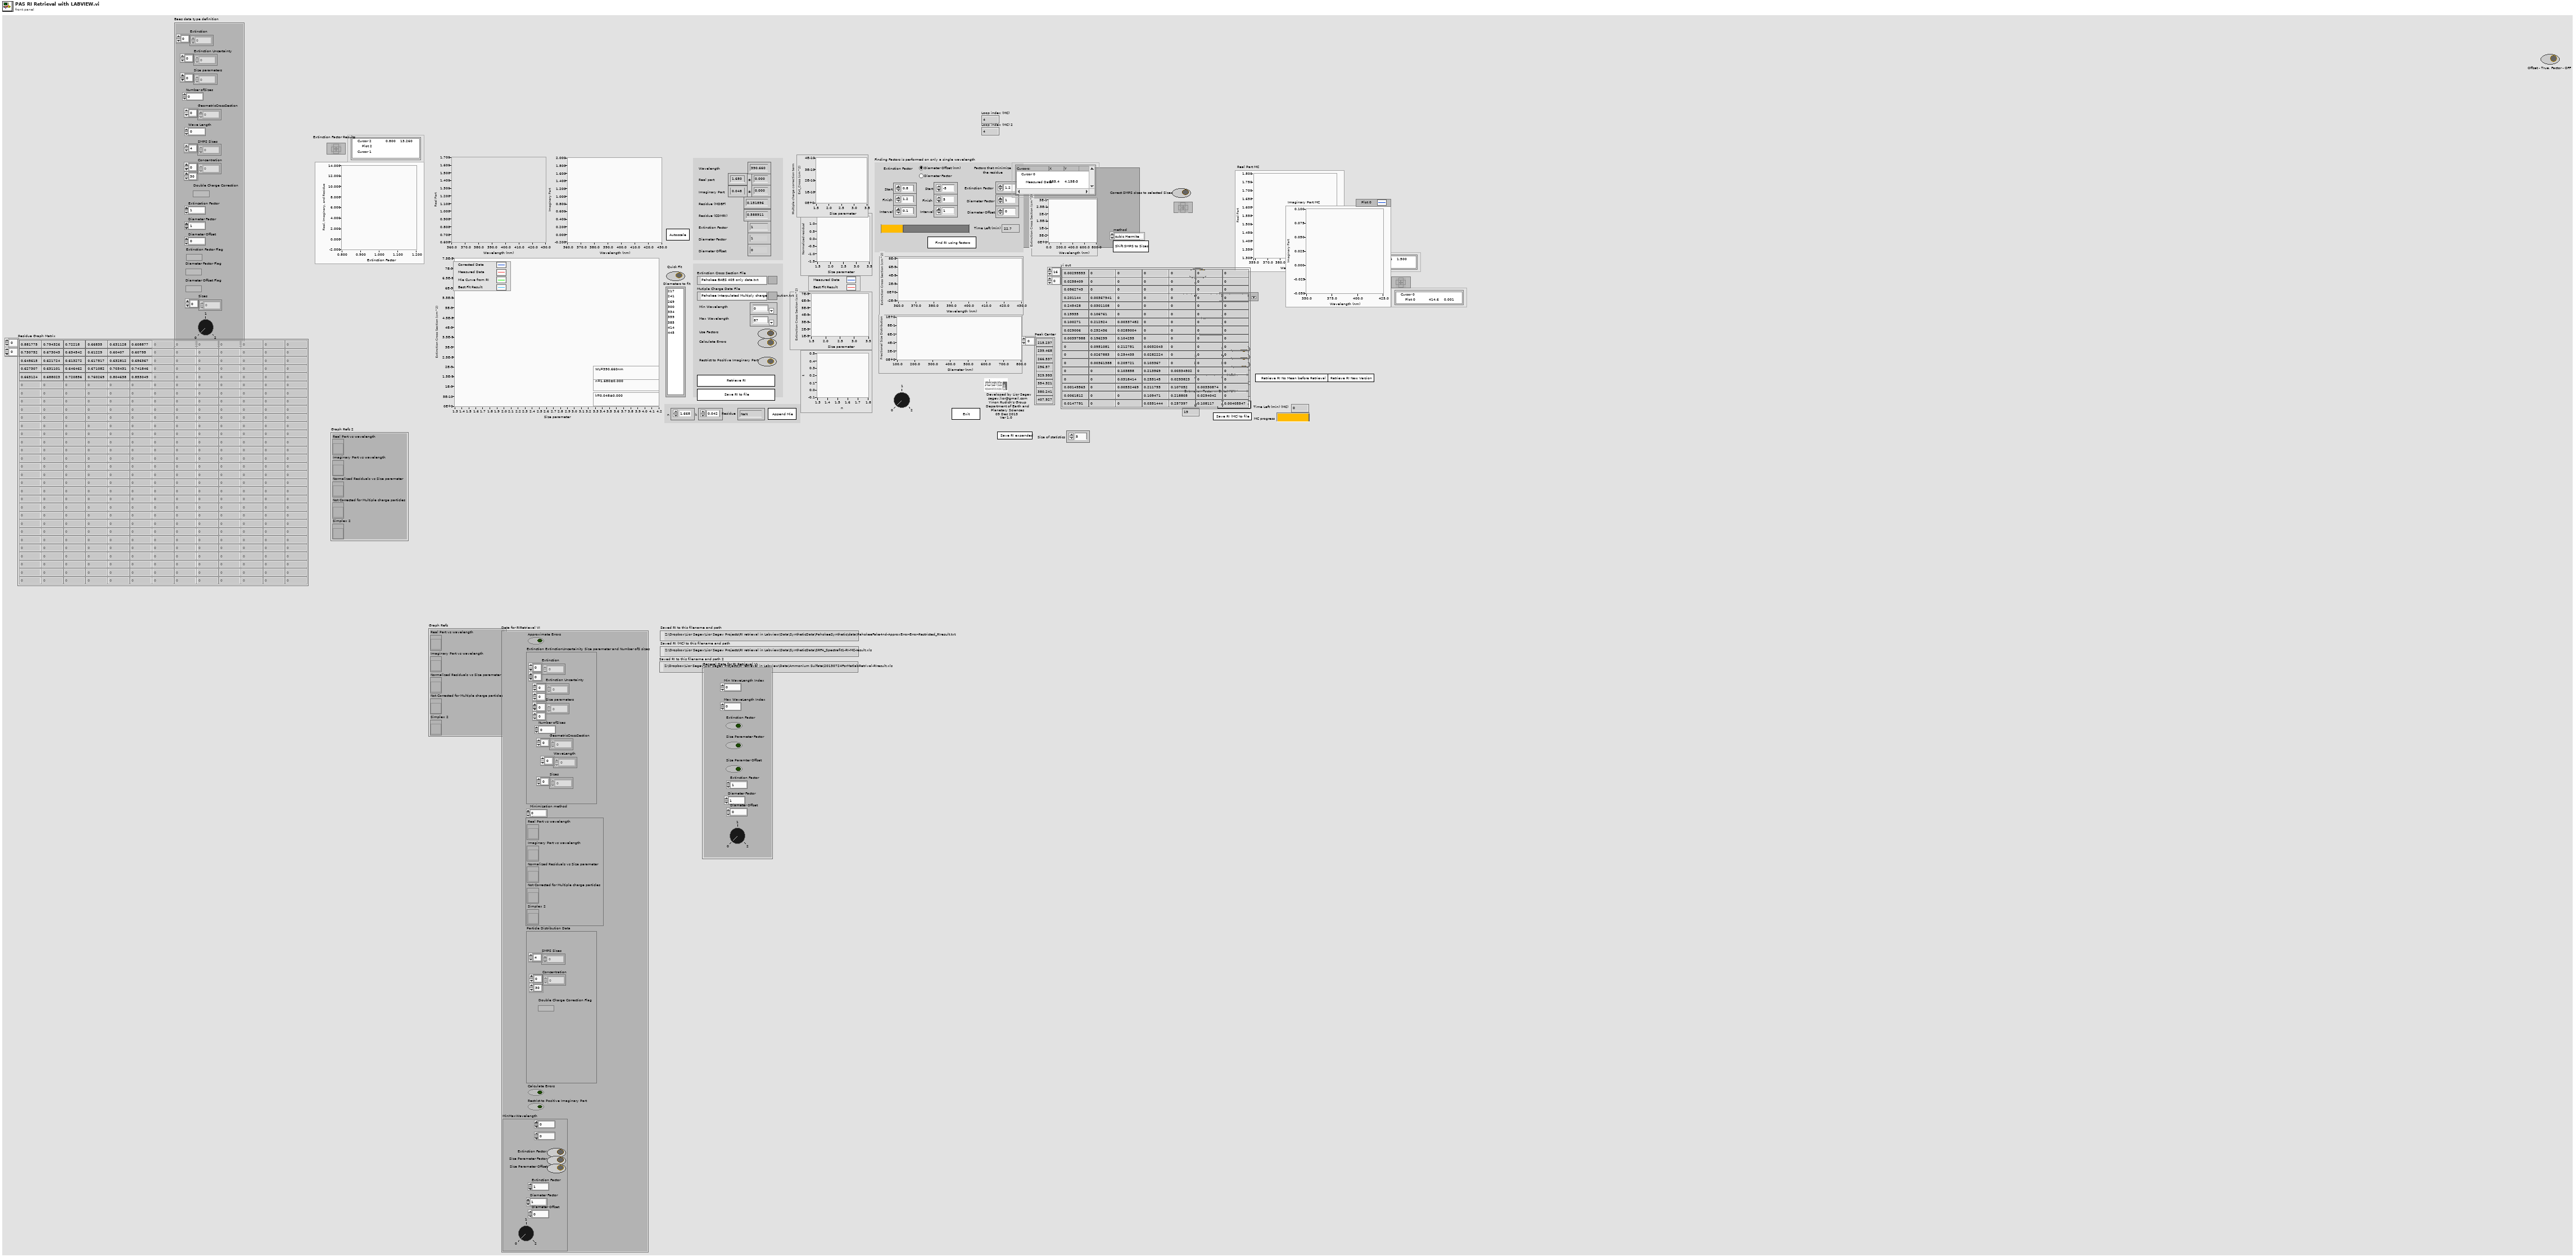
[diagram p1: front panel]
types:
  T1 = cluster{"Ramp Pattern":dbl[], "Extinction":dbl[]}[]
  T2 = cluster{"Size parameters":dbl[], "Normalized Residuals":dbl[]}[]
  T3 = typedef "GeneralDataForRIRetrieval.ctl" = cluster{"Min WaveLength Index":u16, "Max WaveLength Index":u16, "Extinction Factor":bool, "Size Parameter Factor":bool, "Size Paramter Offset":bool, "Extinction Factor":dbl, "Diameter Factor":dbl, "Diameter Offset":dbl, "ExtinctionOrAbsorptionOrScattering":i8}
  T4 = cluster{"Real Part vs wavelength":refnum<vi>, "Imaginary Part vs wavelength":refnum<vi>, "Normalized Residuals vs Size parameter":refnum<vi>, "Not Corrected for Multiple charge particles":refnum<vi>, "Simplex 2":refnum<vi>}
  T5 = typedef "ReadBaesDataTypeDefinition.ctl" = cluster{"Extinction":dbl[][], "Extinction Uncertainty":dbl[][], "Size parameters":dbl[][], "Number ofSizes":dbl, "GeometricCrossSection":dbl[], "WaveLength":dbl[], "Sizes":dbl[]}
  T6 = typedef "ParticleDistributionData.ctl" = cluster{"SMPS Sizes":dbl[], "Concentration":dbl[][], "Double Charge Correction Flag":bool}
  T7 = cluster{"Approximate Errors":bool, "Extinction ExtinctionUncertainity Size parameter and Number ofS sizes":T5, "Minimization method":u16, "Graph Ref":cluster{"Real Part vs wavelength":refnum<vi>, "Imaginary Part vs wavelength":refnum<vi>, "Normalized Residuals vs Size parameter":refnum<vi>, "Not Corrected for Multiple charge particles":refnum<vi>, "Simplex 2":refnum<vi>}, "Particle Distribution Data":T6, "Calculate Errors":bool, "Restrict to Positive Imaginary Part":bool, "MinMaxWavelength":cluster{i32, i32, "Extinction Factor":bool, "Size Parameter Factor":bool, "Size Parameter Offset":bool, "Extinction Factor":dbl, "Diameter Factor":dbl, "Diameter Offset":dbl, "ExtinctionOrAbsorptionOrScattering":i8}}
  T8 = typedef "BaesDataTypeDefinition.ctl" = cluster{"Extinction":dbl[], "Extinction Uncertainty":dbl[], "Size parameters":dbl[], "Number ofSizes":dbl, "GeometricCrossSection":dbl[], "Wave Length":dbl, "SMPS Sizes":dbl[], "Concentration":dbl[][], "Double Charge Correction":bool, "Extincation Factor":dbl, "Diameter Factor":dbl, "Diameter Offset":dbl, "Extinction Factor Flag":bool, "Diameter Factor Flag":bool, "Diameter Offset Flag":bool, "Sizes":dbl[], "ExtinctionOrAbsorptionOrScattering":i8}
  T9 = enum32{"invalid app kind", "Development System", "Run Time System", "Student Edition", "Embedded LabVIEW", "Evaluation", "Custom"}
  T10 = enum32{"Invalid", "Standard", "Closed", "Hidden", "Minimized", "Maximized"}
  T11 = cluster{"SMPS Sizes":dbl[], "Concentration":dbl[]}[]
  T12 = typedef "NI_Gmath.lvlib/stopping criteria.ctl" = cluster{"function tolerance":dbl, "parameter tolerance":dbl, "max iterations":i32, "max function calls":i32, "gradient tolerance":dbl, "max time (sec)":dbl}
  T13 = typedef "LVPoint32TypeDef.ctl" = cluster{"Horizontal":i32, "Vertical":i32}
  T14 = typedef "RIandRIMCResults.ctl" = cluster{"Real RI":dbl[], "Imaginary RI":dbl[], "Std Imaginary RI":dbl[], "Std Real RI":dbl[], "Wavelength":dbl[], "Residue":dbl[], "Extinction Factor":dbl[], "Diameter Factor":dbl[], "Diameter Offset":dbl[], "Best fit result":dbl[][], "Normalized Residuals":dbl[][]}
  T15 = cluster{"Core":cluster{"Current VI Reference":refnum<vi>, "Close Panel on Exit?":bool}, "Extinction ExtinctionUncertainity Size parameter and Number ofS sizes":T5, "Particle Distribution Data":T6, "RI results":T14, "RI MC results":T14, "Extinction Cross section Path":path, "Multiple charge correction file Path":path, "FullExtinctionData":dbl[][], "NumberOfMeasurementsperSize":i32, "Baes data type definition":T8}
  T16 = cluster{"Current VI Reference":refnum<vi>, "Close Panel on Exit?":bool}
  T17 = cluster{"WaveLengths":dbl[], "Extinction":dbl[]}[]
  T18 = cluster{"SMPS Sizes":dbl[], "Concentration":dbl[]}
  T19 = cluster{"\nSMPS sizes":dbl[], "Shifted Concentration":dbl[]}
  T20 = cluster{"Size parameters":dbl[], "Extinction Crosssections":dbl[]}
  T21 = cluster{"Size parameters":dbl[], "Extinction Crosssections":dbl[]}[]
  T22 = cluster{"Real Part vs wavelength":refnum<vi>, "Imaginary Part vs wavelength":refnum<vi>, "Normalized Residuals vs Size parameter":refnum<vi>, "Not Corrected for Multiple charge Best fit result":refnum<vi>, "Simplex":refnum<vi>}
  T23 = typedef "NI_Matrix.lvlib/RealMatrix.ctl" = dbl[][]
  T24 = cluster{"Size parameters":dbl[], "Extinction":dbl[]}
  T25 = cluster{"Size parameters":dbl[], "Normalized Residuals":dbl[]}
  T26 = cluster{"Size parameters":dbl[], "Best fit result":dbl[]}
  T27 = cluster{"Size parameters":dbl[], "Best fit result":dbl[]}[]
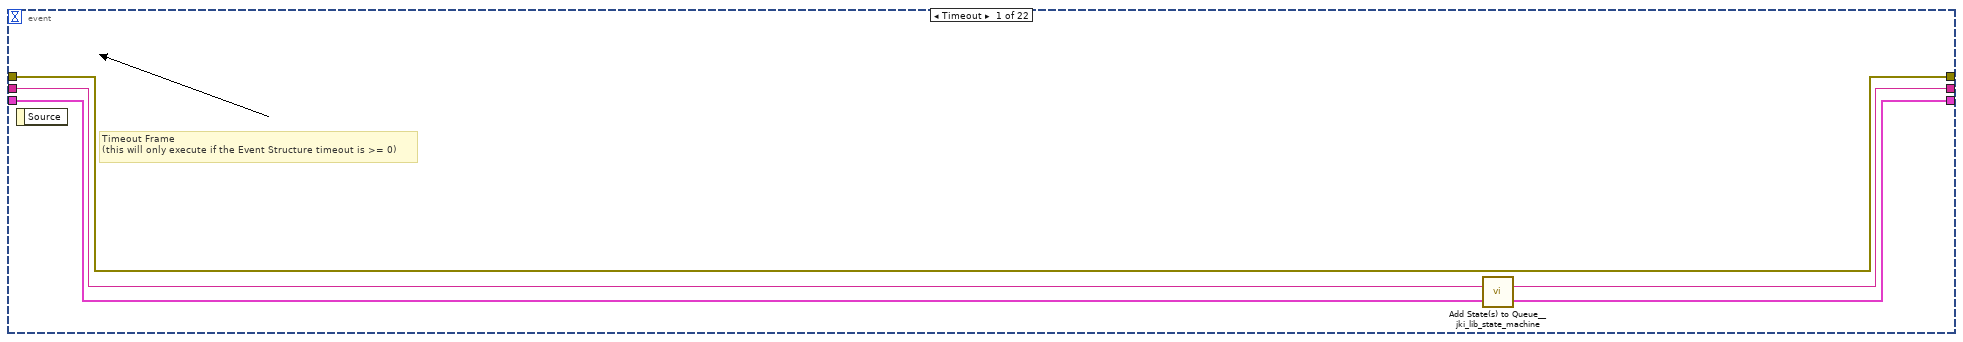
[diagram p3: hidden frame]
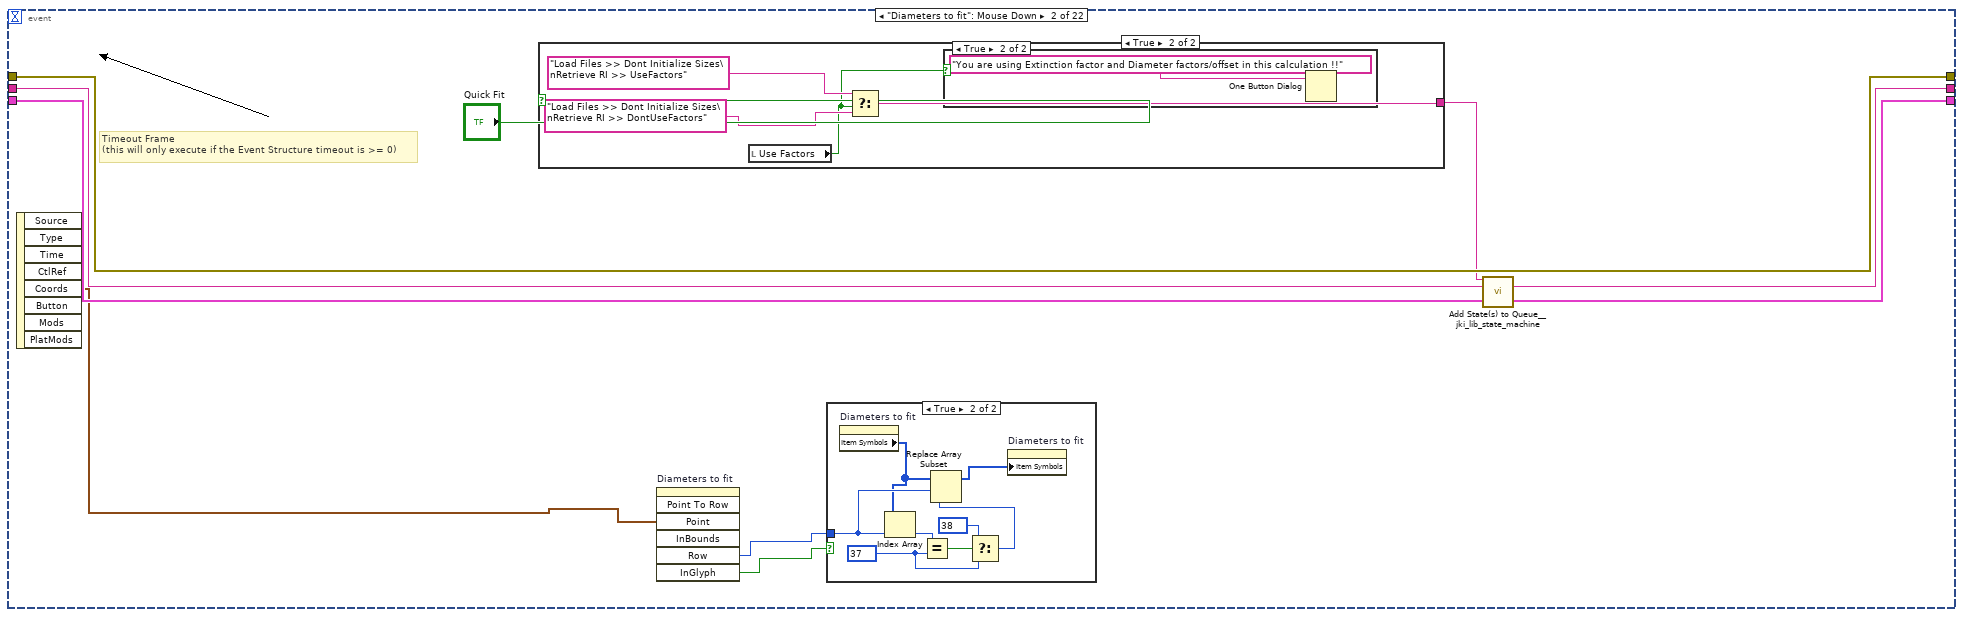
[diagram p4: hidden frame]
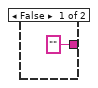
[diagram p5: hidden frame]
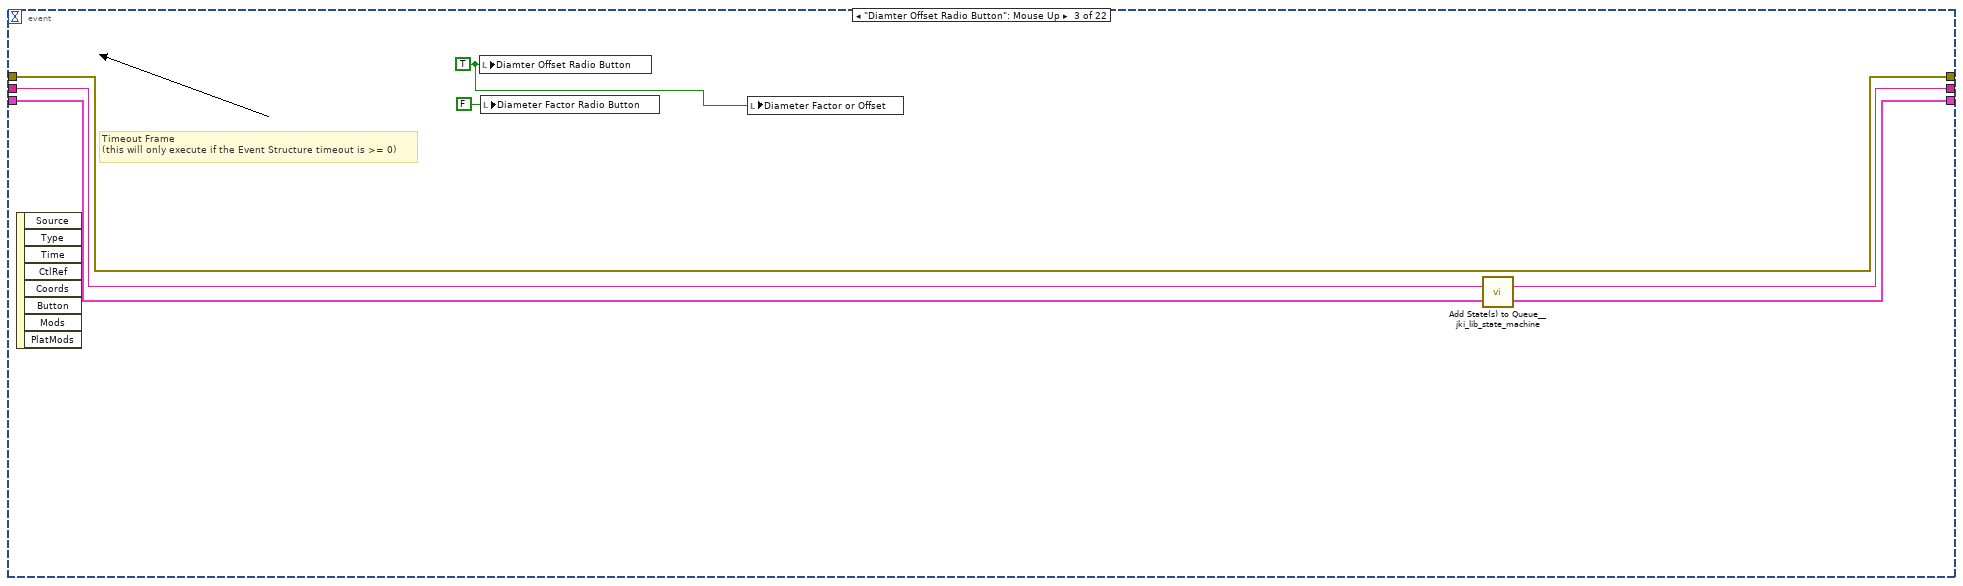
[diagram p8: hidden frame]
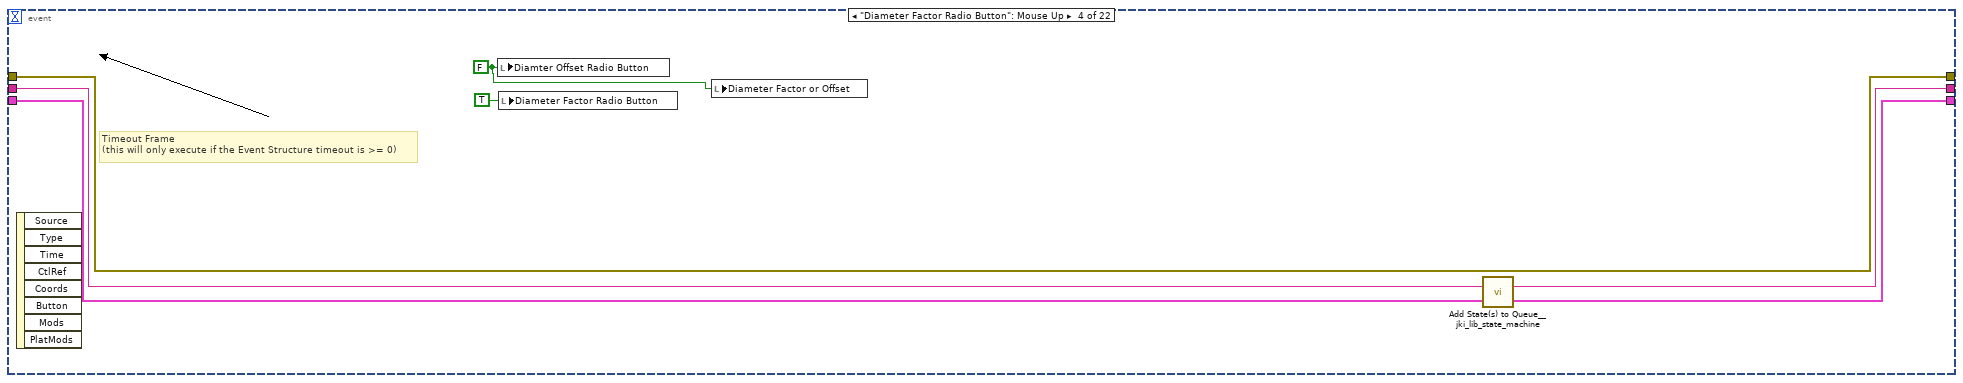
[diagram p9: hidden frame]
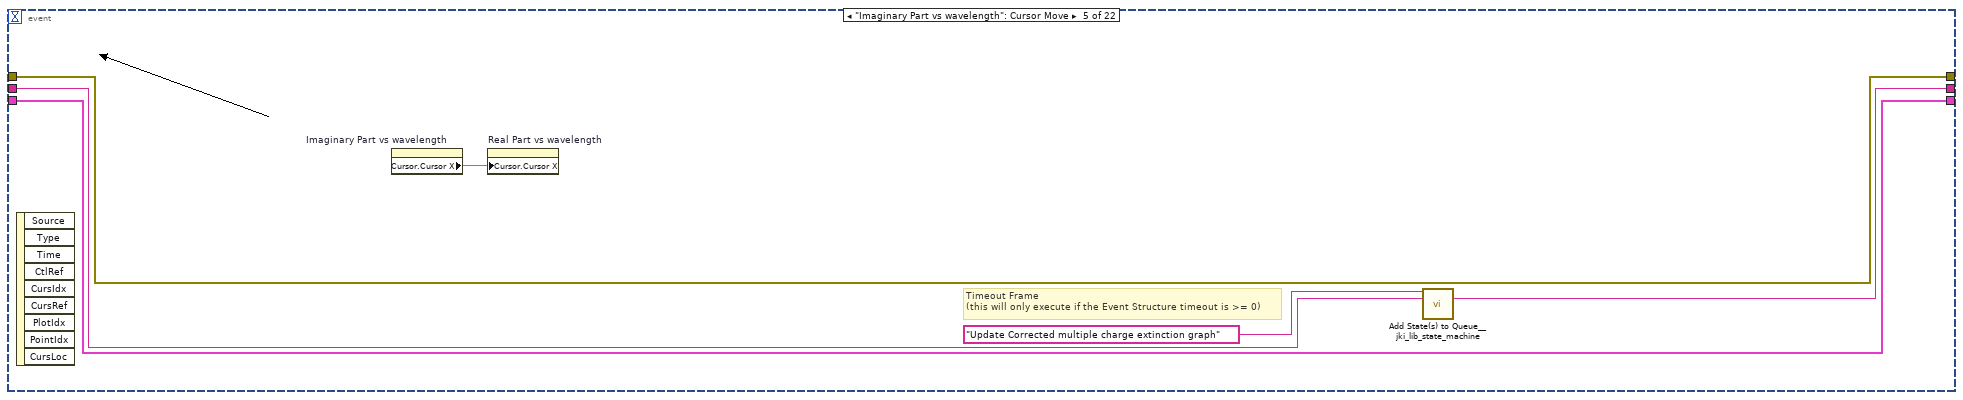
[diagram p10: hidden frame]
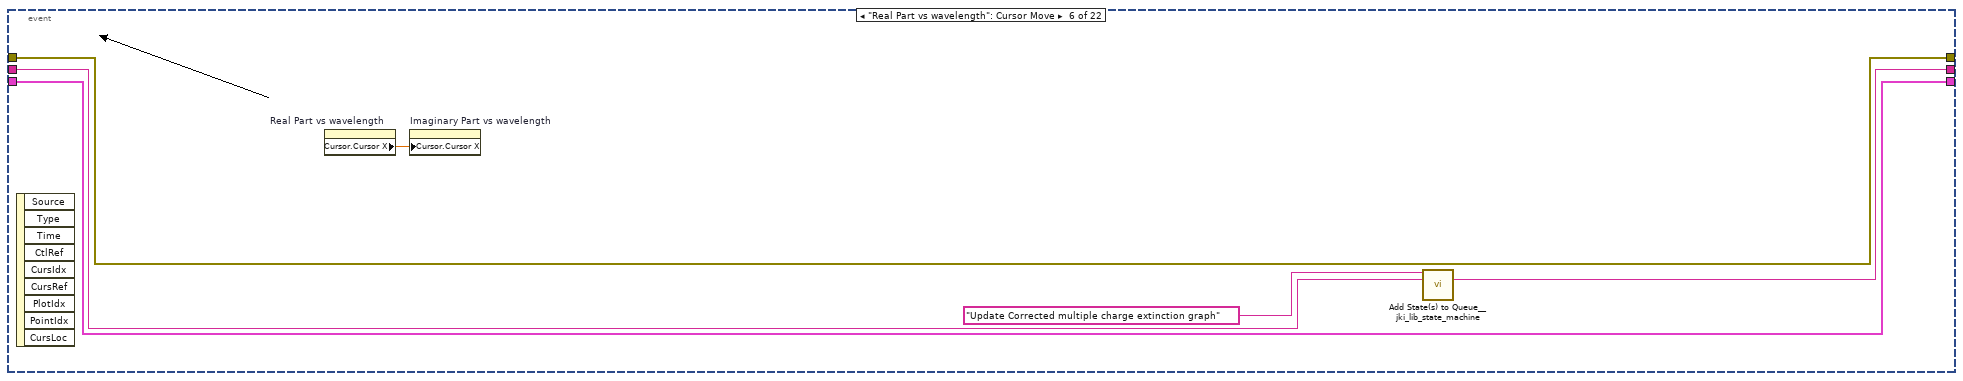
[diagram p11: hidden frame]
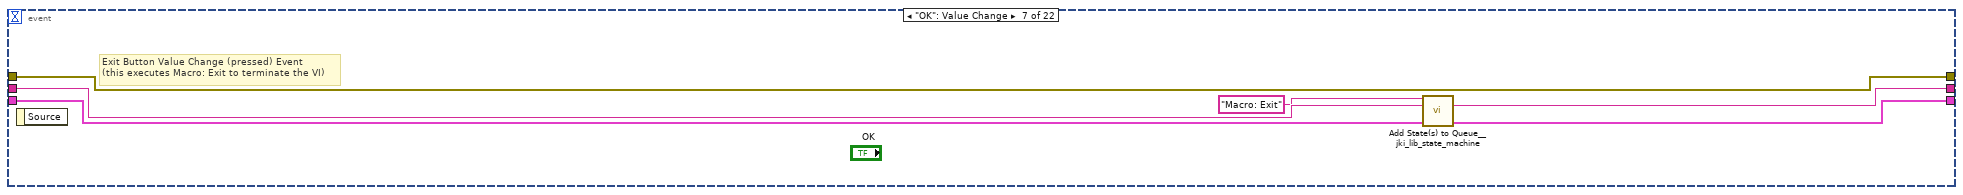
[diagram p12: hidden frame]
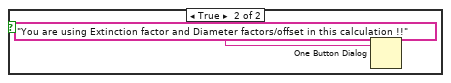
[diagram p13: hidden frame]
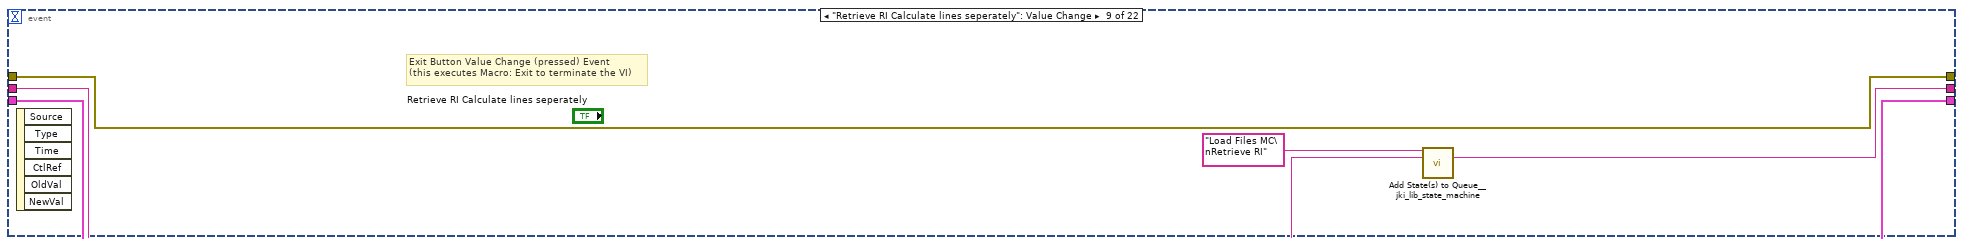
[diagram p14: hidden frame]
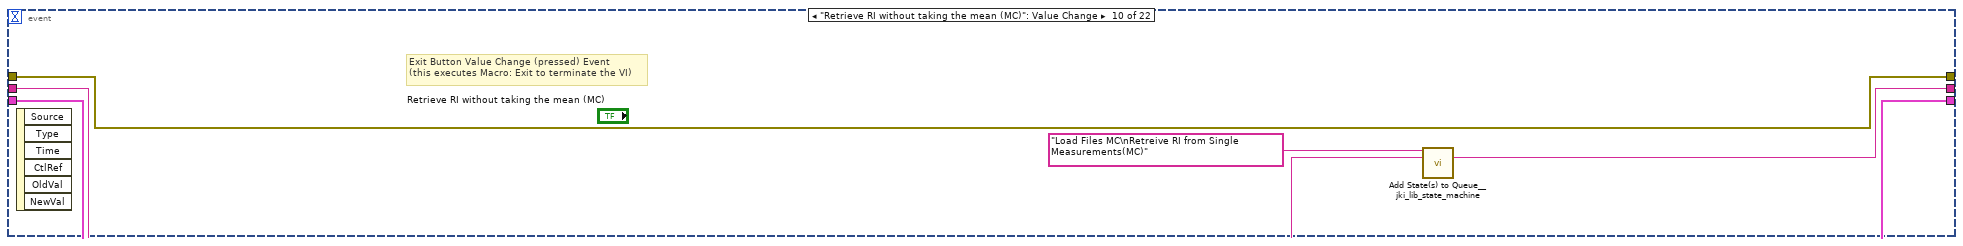
[diagram p15: hidden frame]
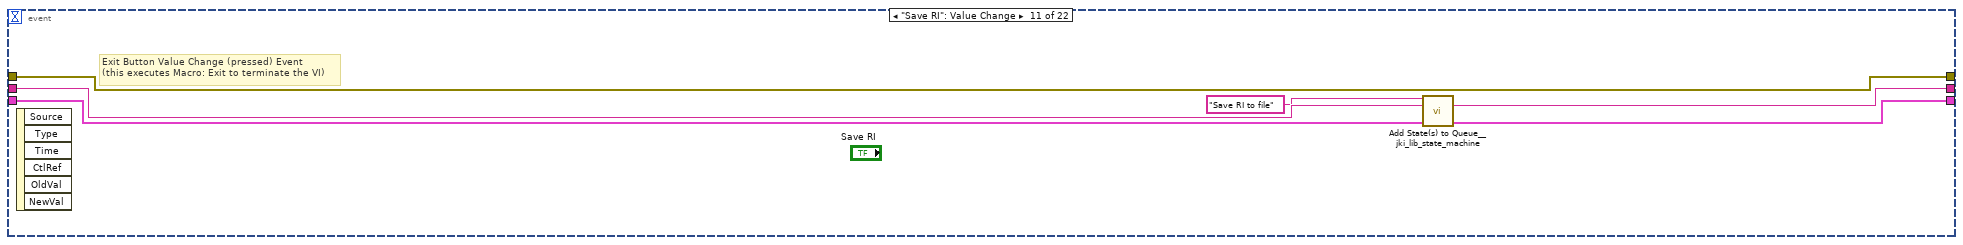
[diagram p16: hidden frame]
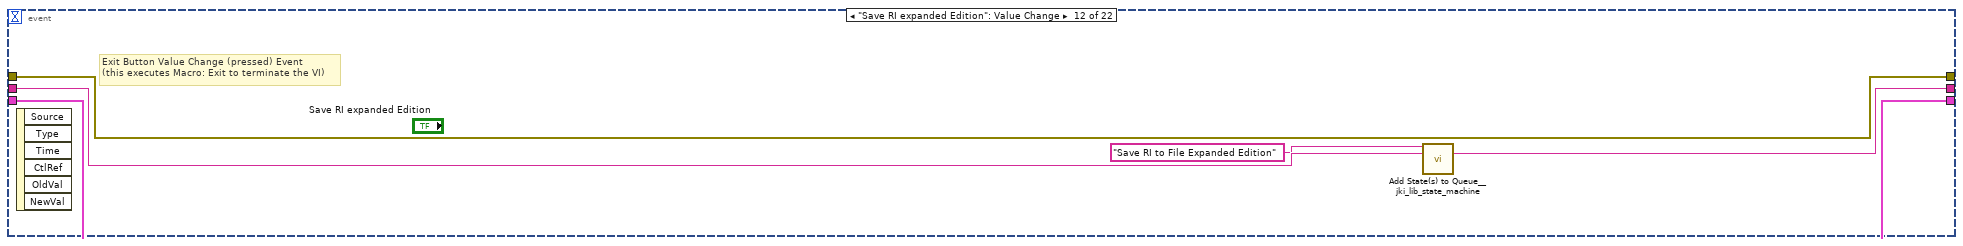
[diagram p17: hidden frame]
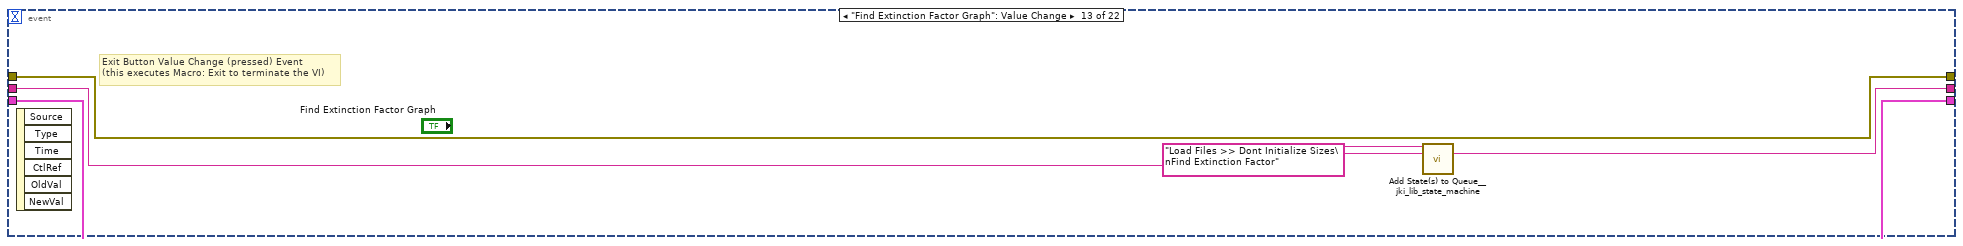
[diagram p18: hidden frame]
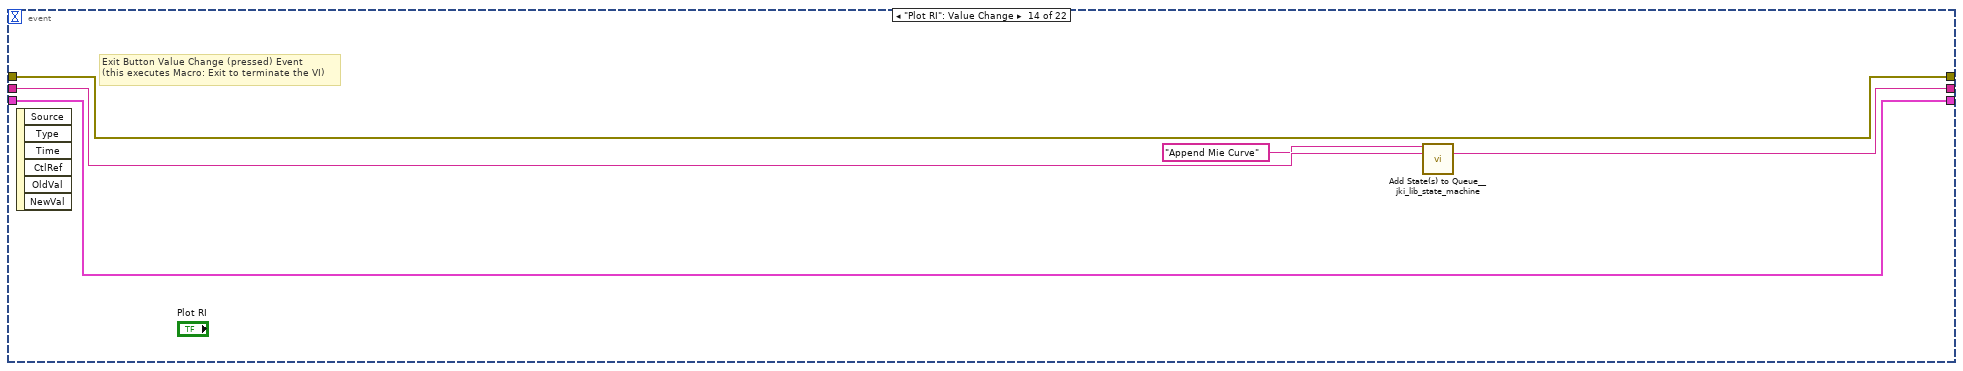
[diagram p19: hidden frame]
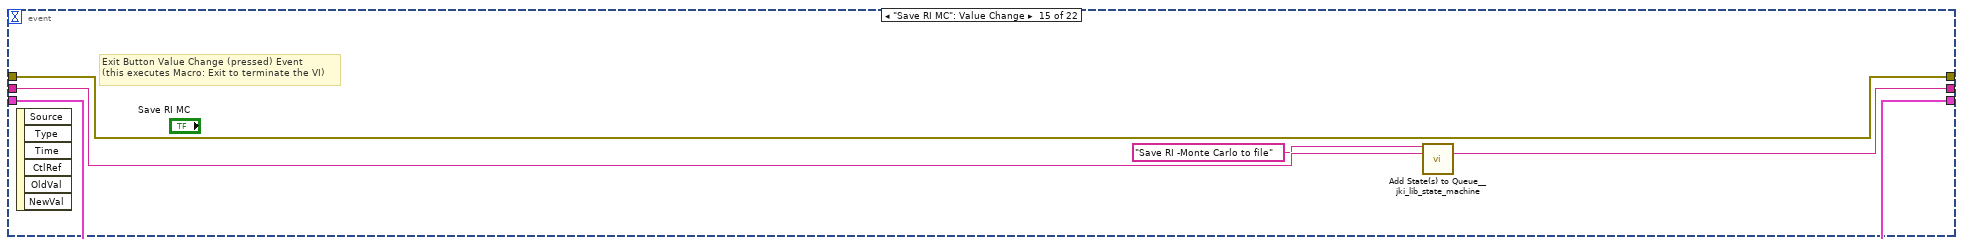
[diagram p20: hidden frame]
diagram:
  (unwired) cluster{dbl[], dbl[]}[] [{[353.79999, 354.37, 354.94, 355.51001, 356.07999, 356.64999, 357.22, 357.78, 358.35001, 358.91, 359.47, 360.03, 360.59, 361.14999, 361.70001, 362.26001, 362.81, 363.35999, 363.91, 364.45999, 365.01001, 365.56, 366.10001, 366.64999, 367.19, 367.73001, 368.26999, 368.81, 369.35001, 369.89001, 370.42001, 370.95999, 371.48999, 372.03, 372.56, 373.09, 373.62, 374.14999, 374.67999, 375.20999, 375.73001, 376.26001, 376.78, 377.31, 377.82999, 378.35001, 378.87, 379.39001, 379.91, 380.42999, 380.95001, 381.47, 381.98001, 382.5, 383.01001, 383.53, 384.04001, 384.54999, 385.07001, 385.57999, 386.09, 386.60001, 387.10999, 387.62, 388.13, 388.63, 389.14001, 389.64999, 390.14999, 388.63, 389.14001, 389.64999, 390.14999, 390.66, 391.16, 391.67001, 392.17001, 392.67999, 393.17999, 393.67999, 394.17999, 394.67999, 395.19, 395.69, 396.19, 396.69, 397.19, 397.69, 398.19, 398.69, 399.19, 399.67999, 400.17999, 400.67999, 401.17999, 401.67999, 402.17001, 402.67001, 403.17001, 403.66, 404.16, 404.66, 405.14999, 405.64999, 406.14999, 406.64001, 407.14001, 407.64001, 408.13, 408.63, 409.13, 409.62, 410.12, 410.62, 411.10999, 411.60999, 412.10001, 412.60001, 413.10001, 413.60001, 414.09, 414.59, 415.09, 415.59, 416.07999, 416.57999, 417.07999, 417.57999, 418.07999, 418.57999], [-0.006880589406937364, -0.005591015240643177, -0.0008128900086740067, 0.0059132125129690355, 0.004727233671001155, 0.005285323022981176, 0.012079702376504426, 0.013295932917972094, 0.009723681324539938, 0.01340675951578305, 0.014300736755976685, 0.017412400216708195, 0.016082847953221062, 0.019541949361009746, 0.016681812204333245, 0.021839119627984467, 0.01917857630542129, 0.01659316249089897, 0.017920546232635386, 0.02331211752971285, 0.018736628440528875, 0.02278859303667559, 0.020160162589600072, 0.01944517701034782, 0.01722059774576336, 0.014545686876081154, 0.017064244530774875, 0.014871257634513302, 0.015814167710632307, 0.012323804928601011, 0.017001137568295226, 0.01761462364709586, 0.011094176200131175, 0.013484050217230092, 0.015463713328499572, 0.017445979654003158, 0.017890194826904918, 0.012171772373985729, 0.0090971027467458, 0.010861800449201833, 0.009486644105636509, 0.009660218265489668, 0.011543706295196892, 0.009241826302022669, 0.0043825353242573275, 0.006012733183160885, 0.016684276899031823, 0.004574877464619924, 0.004680287507653695, 0.005436664247245053, 0.005769621008366801, 0.007016844481986471, 0.005292591657780566, 0.0023362286578048827, 0.001404106784902966, 0.006018627453886426, 0.005868676603131451, 0.004574542292684771, 0.00013407550315604303, 0.005111191491887428, 0.006244050999230227, 0.008470422941900313, 0.0019502929036388976, 0.00693045579799217, 0.00729891092487377, 0.006591697414114595, -0.00464719874347794, -0.0028833235584898023, 0.0030601034901337606, -0.019172722466464624, 0.00349415319418767, -0.019612863241454764, 0.006230360324734642, -0.007644525136092856, -0.0024464061374237676, -0.015743142364772214, -0.01362771525815333, 0.0023827303007783484, 0.004434076127836306, 0.0015447059453072153, -0.0012530544220862782, 0.013970670419985256, 0.005734164261953947, 0.008763635301725982, 0.006956973905904259, 0.0058963200240359104, 0.004165371933482626, 0.009600835719607804, 0.0037134970421865933, 0.01607998543651406, 0.007081749858913052, 0.014576117182728877, 0.010330077196118458, 0.013431346724388227, 0.009247446675431951, 0.013068538923394903, 0.009279456157815679, 0.013932752616816237, 0.013225407198184207, 0.014934507206195071, 0.017106424708032086, 0.01564773346122451, 0.017710188001506998, 0.011882676676028447, 0.014042275741809086, 0.014230648119115306, 0.011795090172377915, 0.01414643231400618, 0.01678394258342081, 0.006007592633110041, 0.012137073369673021, 0.015868997327494014, 0.008004974625515329, 0.012176508619891986, 0.011391254549822344, 0.01562344561258754, 0.005349593450524416, 0.012534566898108031, 0.015731735948216675, 0.012454435731493445, 0.016355219901748506, 0.007853560039517043, 0.0044201289692190875, 0.009950585420452563, 0.0011992242078176175, -0.0040610702724316675, 0.005166605821146673, 0.00788498225462348, -0.004714349788695529, 0.007145714404910847]}, ...(3 in all)] ("Imaginary Part vs wavelength")
  (unwired) cluster{dbl[], dbl[]}[] [{[353.79999, 354.37, 354.94, 355.51001, 356.07999, 356.64999, 357.22, 357.78, 358.35001, 358.91, 359.47, 360.03, 360.59, 361.14999, 361.70001, 362.26001, 362.81, 363.35999, 363.91, 364.45999, 365.01001, 365.56, 366.10001, 366.64999, 367.19, 367.73001, 368.26999, 368.81, 369.35001, 369.89001, 370.42001, 370.95999, 371.48999, 372.03, 372.56, 373.09, 373.62, 374.14999, 374.67999, 375.20999, 375.73001, 376.26001, 376.78, 377.31, 377.82999, 378.35001, 378.87, 379.39001, 379.91, 380.42999, 380.95001, 381.47, 381.98001, 382.5, 383.01001, 383.53, 384.04001, 384.54999, 385.07001, 385.57999, 386.09, 386.60001, 387.10999, 387.62, 388.13, 388.63, 389.14001, 389.64999, 390.14999, 388.63, 389.14001, 389.64999, 390.14999, 390.66, 391.16, 391.67001, 392.17001, 392.67999, 393.17999, 393.67999, 394.17999, 394.67999, 395.19, 395.69, 396.19, 396.69, 397.19, 397.69, 398.19, 398.69, 399.19, 399.67999, 400.17999, 400.67999, 401.17999, 401.67999, 402.17001, 402.67001, 403.17001, 403.66, 404.16, 404.66, 405.14999, 405.64999, 406.14999, 406.64001, 407.14001, 407.64001, 408.13, 408.63, 409.13, 409.62, 410.12, 410.62, 411.10999, 411.60999, 412.10001, 412.60001, 413.10001, 413.60001, 414.09, 414.59, 415.09, 415.59, 416.07999, 416.57999, 417.07999, 417.57999, 418.07999, 418.57999], [1.6483722836524246, 1.6546363395359365, 1.647298907653894, 1.6533287796168583, 1.6513909602141936, 1.6441728100483295, 1.6485630092327472, 1.6465913680498476, 1.644326968253007, 1.6458723273169005, 1.6423749873362237, 1.6435071871004756, 1.6412154858600103, 1.6396834087598822, 1.6391132715105765, 1.6382846511661762, 1.6358307684719318, 1.6354408519662669, 1.6334428509272396, 1.6328074965992703, 1.630211530333035, 1.629597879928187, 1.6276773015694914, 1.6248549924331006, 1.6221911228582016, 1.619860370624227, 1.6186660879658288, 1.6177483954461045, 1.618059125989092, 1.616294733806861, 1.6164932554209357, 1.6163255198620012, 1.615138021497404, 1.6164105257665495, 1.617235077199874, 1.6147912416880703, 1.6164196882297972, 1.6150368907017385, 1.6144850551191468, 1.6133228562399728, 1.6128153905854543, 1.6139403869979996, 1.6131967111234533, 1.6143159173824806, 1.6121220874076225, 1.6114366661699004, 1.6094507790415067, 1.6108839833096118, 1.6122492163476982, 1.6122322997299472, 1.6077321043459216, 1.6138723793940135, 1.6118005408009028, 1.6157486465235684, 1.6147077896853421, 1.6142964675684908, 1.614804272990439, 1.6117647309822476, 1.6161328124848642, 1.6101356911507883, 1.612094662439775, 1.6118531546799915, 1.614236269971587, 1.6062328837497617, 1.6105586500151539, 1.6108228692284308, 1.6178782024106462, 1.6087987962691102, 1.6074587087659151, 1.6187364188290658, 1.6209092605148896, 1.6151493452793495, 1.6182798966697, 1.6109338276299237, 1.6085077651242317, 1.613655399235577, 1.612511934789509, 1.607851046633587, 1.6057532268507935, 1.6024870719133475, 1.6038884748636346, 1.605523559015856, 1.5960101592112506, 1.5997312604952778, 1.598377877440321, 1.597392154092918, 1.600589807386528, 1.5995684913350448, 1.5979434008328421, 1.5961998900762004, 1.5970150338732805, 1.5939307380342091, 1.596156816544494, 1.5962182334684933, 1.597512896681686, 1.595101996088882, 1.5933960300930927, 1.592688229676817, 1.5913322143224218, 1.5917530088094214, 1.591614538502429, 1.5914637114820218, 1.5878221602705458, 1.5928834293750267, 1.5915729711917386, 1.587309104722474, 1.5918112038963161, 1.5881066262119135, 1.584965267353939, 1.5914289179893895, 1.586911737372422, 1.581731065142223, 1.5886590769172397, 1.5849680475176062, 1.586099454232746, 1.581195601241917, 1.5854707251659343, 1.5865012245981702, 1.5838978086861526, 1.584800751487047, 1.5848505559733816, 1.5857486239152707, 1.585591816537336, 1.5810404634087085, 1.5851743649291072, 1.5859104770394237, 1.5823664432736304, 1.5792071958230995, 1.590530467368216, 1.5870072549949592]}, {[353.79999, 353.79999, 353.79999, 354.37, 354.37, 354.37, 354.94, 354.94, 354.94, 355.51001, 355.51001, 355.51001, 356.07999, 356.07999, 356.07999, 356.64999, 356.64999, 356.64999, 357.22, 357.22, 357.22, 357.78, 357.78, 357.78, 358.35001, 358.35001, 358.35001, 358.91, 358.91, 358.91, 359.47, 359.47, 359.47, 360.03, 360.03, 360.03, 360.59, 360.59, 360.59, 361.14999, 361.14999, 361.14999, 361.70001, 361.70001, 361.70001, 362.26001, 362.26001, 362.26001, 362.81, 362.81, 362.81, 363.35999, 363.35999, 363.35999, 363.91, 363.91, 363.91, 364.45999, 364.45999, 364.45999, 365.01001, 365.01001, 365.01001, 365.56, 365.56, 365.56, 366.10001, 366.10001, 366.10001, 366.64999, 366.64999, 366.64999, 367.19, 367.19, 367.19, 367.73001, 367.73001, 367.73001, 368.26999, 368.26999, 368.26999, 368.81, 368.81, 368.81, 369.35001, 369.35001, 369.35001, 369.89001, 369.89001, 369.89001, 370.42001, 370.42001, 370.42001, 370.95999, 370.95999, 370.95999, 371.48999, 371.48999, 371.48999, 372.03, 372.03, 372.03, 372.56, 372.56, 372.56, 373.09, 373.09, 373.09, 373.62, 373.62, 373.62, 374.14999, 374.14999, 374.14999, 374.67999, 374.67999, 374.67999, 375.20999, 375.20999, 375.20999, 375.73001, 375.73001, 375.73001, 376.26001, 376.26001, 376.26001, 376.78, 376.78, 376.78, 377.31, 377.31, 377.31, 377.82999, 377.82999, 377.82999, 378.35001, 378.35001, 378.35001, 378.87, 378.87, 378.87, 379.39001, 379.39001, 379.39001, 379.91, 379.91, 379.91, 380.42999, 380.42999, 380.42999, 380.95001, 380.95001, 380.95001, 381.47, 381.47, 381.47, 381.98001, 381.98001, 381.98001, 382.5, 382.5, 382.5, 383.01001, 383.01001, 383.01001, 383.53, 383.53, 383.53, 384.04001, 384.04001, 384.04001, 384.54999, 384.54999, 384.54999, 385.07001, 385.07001, 385.07001, 385.57999, 385.57999, 385.57999, 386.09, 386.09, 386.09, 386.60001, 386.60001, 386.60001, 387.10999, 387.10999, 387.10999, 387.62, 387.62, 387.62, 388.13, 388.13, 388.13, 388.63, 388.63, 388.63, 389.14001, 389.14001, 389.14001, 389.64999, 389.64999, 389.64999, 390.14999, 390.14999, 390.14999, 388.63, 388.63, 388.63, 389.14001, 389.14001, 389.14001, 389.64999, 389.64999, 389.64999, 390.14999, 390.14999, 390.14999, 390.66, 390.66, 390.66, 391.16, 391.16, 391.16, 391.67001, 391.67001, 391.67001, 392.17001, 392.17001, 392.17001, 392.67999, 392.67999, 392.67999, 393.17999, 393.17999, 393.17999, 393.67999, 393.67999, 393.67999, 394.17999, 394.17999, 394.17999, 394.67999, 394.67999, 394.67999, 395.19, 395.19, 395.19, 395.69, 395.69, 395.69, 396.19, 396.19, 396.19, 396.69, 396.69, 396.69, 397.19, 397.19, 397.19, 397.69, 397.69, 397.69, 398.19, 398.19, 398.19, 398.69, 398.69, 398.69, 399.19, 399.19, 399.19, 399.67999, 399.67999, 399.67999, 400.17999, 400.17999, 400.17999, 400.67999, 400.67999, 400.67999, 401.17999, 401.17999, 401.17999, 401.67999, 401.67999, 401.67999, 402.17001, 402.17001, 402.17001, 402.67001, 402.67001, 402.67001, 403.17001, 403.17001, 403.17001, 403.66, 403.66, 403.66, 404.16, 404.16, 404.16, 404.66, 404.66, 404.66, 405.14999, 405.14999, 405.14999, 405.64999, 405.64999, 405.64999, 406.14999, 406.14999, 406.14999, 406.64001, 406.64001, 406.64001, 407.14001, 407.14001, 407.14001, 407.64001, 407.64001, 407.64001, 408.13, 408.13, 408.13, 408.63, 408.63, 408.63, 409.13, 409.13, 409.13, 409.62, 409.62, 409.62, 410.12, 410.12, 410.12, 410.62, 410.62, 410.62, 411.10999, 411.10999, 411.10999, 411.60999, 411.60999, 411.60999, 412.10001, 412.10001, 412.10001, 412.60001, 412.60001, 412.60001, 413.10001, 413.10001, 413.10001, 413.60001, 413.60001, 413.60001, 414.09, 414.09, 414.09, 414.59, 414.59, 414.59, 415.09, 415.09, 415.09, 415.59, 415.59, 415.59, 416.07999, 416.07999, 416.07999, 416.57999, 416.57999, 416.57999, 417.07999, 417.07999, 417.07999, 417.57999, 417.57999, 417.57999, 418.07999, 418.07999, 418.07999, 418.57999, 418.57999, 418.57999], [nan, 1.6563722836524246, 1.6403722836524246, nan, 1.6616363395359364, 1.6476363395359366, nan, 1.6542989076538939, 1.640298907653894, nan, 1.6603287796168582, 1.6463287796168584, nan, 1.6573909602141936, 1.6453909602141936, nan, 1.6501728100483295, 1.6381728100483295, nan, 1.6535630092327471, 1.6435630092327473, nan, 1.6515913680498475, 1.6415913680498477, nan, 1.649326968253007, 1.6393269682530072, nan, 1.6508723273169004, 1.6408723273169006, nan, 1.6473749873362236, 1.6373749873362238, nan, 1.6485071871004755, 1.6385071871004757, nan, 1.6462154858600102, 1.6362154858600104, nan, 1.6436834087598822, 1.6356834087598822, nan, 1.6431132715105765, 1.6351132715105765, nan, 1.6422846511661762, 1.6342846511661762, nan, 1.6398307684719318, 1.6318307684719318, nan, 1.6394408519662669, 1.6314408519662669, nan, 1.6374428509272396, 1.6294428509272396, nan, 1.6368074965992703, 1.6288074965992703, nan, 1.634211530333035, 1.626211530333035, nan, 1.633597879928187, 1.625597879928187, nan, 1.6316773015694914, 1.6236773015694914, nan, 1.6288549924331006, 1.6208549924331006, nan, 1.6261911228582016, 1.6181911228582015, nan, 1.623860370624227, 1.615860370624227, nan, 1.6226660879658288, 1.6146660879658288, nan, 1.6217483954461045, 1.6137483954461045, nan, 1.622059125989092, 1.614059125989092, nan, 1.620294733806861, 1.612294733806861, nan, 1.6204932554209357, 1.6124932554209357, nan, 1.6203255198620012, 1.6123255198620012, nan, 1.619138021497404, 1.611138021497404, nan, 1.6204105257665495, 1.6124105257665495, nan, 1.621235077199874, 1.613235077199874, nan, 1.6187912416880703, 1.6107912416880703, nan, 1.6204196882297972, 1.6124196882297972, nan, 1.6190368907017385, 1.6110368907017385, nan, 1.6184850551191468, 1.6104850551191467, nan, 1.6173228562399729, 1.6093228562399728, nan, 1.6168153905854543, 1.6088153905854543, nan, 1.6179403869979996, 1.6099403869979996, nan, 1.6171967111234533, 1.6091967111234533, nan, 1.6183159173824806, 1.6103159173824806, nan, 1.6161220874076225, 1.6081220874076225, nan, 1.6154366661699004, 1.6074366661699004, nan, 1.6134507790415067, 1.6054507790415067, nan, 1.6148839833096118, 1.6068839833096118, nan, 1.6172492163476981, 1.6072492163476984, nan, 1.617232299729947, 1.6072322997299473, nan, 1.6127321043459215, 1.6027321043459217, nan, 1.6188723793940134, 1.6088723793940136, nan, 1.6168005408009027, 1.606800540800903, nan, 1.6207486465235683, 1.6107486465235685, nan, 1.619707789685342, 1.6097077896853422, nan, 1.6192964675684907, 1.6092964675684909, nan, 1.619804272990439, 1.6098042729904392, nan, 1.6167647309822475, 1.6067647309822477, nan, 1.621132812484864, 1.6111328124848643, nan, 1.6161356911507883, 1.6041356911507882, nan, 1.618094662439775, 1.606094662439775, nan, 1.6178531546799915, 1.6058531546799915, nan, 1.620236269971587, 1.608236269971587, nan, 1.6122328837497617, 1.6002328837497617, nan, 1.6175586500151538, 1.603558650015154, nan, 1.6168228692284308, 1.6048228692284308, nan, 1.624878202410646, 1.6108782024106463, nan, 1.61579879626911, 1.6017987962691103, nan, 1.614458708765915, 1.6004587087659152, nan, 1.6347364188290658, 1.6027364188290658, nan, 1.6349092605148896, 1.6069092605148896, nan, 1.6281493452793494, 1.6021493452793496, nan, 1.6302798966697, 1.6062798966697, nan, 1.6219338276299236, 1.5999338276299238, nan, 1.6185077651242317, 1.5985077651242316, nan, 1.622655399235577, 1.6046553992355772, nan, 1.6215119347895088, 1.603511934789509, nan, 1.6168510466335868, 1.598851046633587, nan, 1.6137532268507935, 1.5977532268507935, nan, 1.6104870719133475, 1.5944870719133475, nan, 1.6108884748636345, 1.5968884748636347, nan, 1.613523559015856, 1.597523559015856, nan, 1.6030101592112505, 1.5890101592112507, nan, 1.6067312604952777, 1.592731260495278, nan, 1.605377877440321, 1.591377877440321, nan, 1.6043921540929178, 1.590392154092918, nan, 1.606589807386528, 1.594589807386528, nan, 1.6055684913350448, 1.5935684913350447, nan, 1.604943400832842, 1.5909434008328422, nan, 1.6031998900762003, 1.5891998900762005, nan, 1.6030150338732805, 1.5910150338732805, nan, 1.598930738034209, 1.5889307380342093, nan, 1.602156816544494, 1.590156816544494, nan, 1.6022182334684933, 1.5902182334684933, nan, 1.603512896681686, 1.591512896681686, nan, 1.601101996088882, 1.589101996088882, nan, 1.5993960300930927, 1.5873960300930927, nan, 1.598688229676817, 1.586688229676817, nan, 1.5963322143224217, 1.5863322143224219, nan, 1.5967530088094213, 1.5867530088094215, nan, 1.5966145385024288, 1.586614538502429, nan, 1.5964637114820217, 1.586463711482022, nan, 1.5928221602705457, 1.582822160270546, nan, 1.5978834293750266, 1.5878834293750268, nan, 1.5965729711917385, 1.5865729711917387, nan, 1.592309104722474, 1.5823091047224742, nan, 1.596811203896316, 1.5868112038963162, nan, 1.5931066262119133, 1.5831066262119136, nan, 1.590965267353939, 1.578965267353939, nan, 1.5964289179893894, 1.5864289179893896, nan, 1.5919117373724219, 1.581911737372422, nan, 1.5867310651422228, 1.576731065142223, nan, 1.5946590769172397, 1.5826590769172397, nan, 1.5899680475176061, 1.5799680475176063, nan, 1.592099454232746, 1.580099454232746, nan, 1.587195601241917, 1.575195601241917, nan, 1.5914707251659344, 1.5794707251659343, nan, 1.5925012245981702, 1.5805012245981702, nan, 1.5898978086861526, 1.5778978086861526, nan, 1.591800751487047, 1.5778007514870471, nan, 1.5918505559733815, 1.5778505559733818, nan, 1.5927486239152706, 1.5787486239152708, nan, 1.5925918165373358, 1.578591816537336, nan, 1.5880404634087084, 1.5740404634087086, nan, 1.5931743649291072, 1.5771743649291072, nan, 1.5939104770394237, 1.5779104770394237, nan, 1.5903664432736304, 1.5743664432736304, nan, 1.5882071958230994, 1.5702071958230996, nan, 1.5995304673682158, 1.581530467368216, nan, 1.5970072549949592, 1.5770072549949592]}, {[353.79999, 354.37, 354.94, 355.51001, 356.07999, 356.64999, 357.22, 357.78, 358.35001, 358.91, 359.47, 360.03, 360.59, 361.14999, 361.70001, 362.26001, 362.81, 363.35999, 363.91, 364.45999, 365.01001, 365.56, 366.10001, 366.64999, 367.19, 376.78, 378.87, 379.39001, 379.91, 380.42999, 380.95001, 381.47, 381.98001, 382.5, 383.01001, 383.53, 384.04001, 384.54999, 385.07001, 385.57999, 386.09, 386.60001, 387.10999, 387.62, 388.13, 388.63, 389.14001, 389.64999, 390.14999, 388.63, 389.14001, 389.64999, 390.14999, 390.66, 391.16, 391.67001, 392.17001, 392.67999, 393.17999, 393.67999, 394.17999, 394.67999, 395.19, 395.69, 396.19, 396.69, 397.19, 397.69, 398.19, 398.69, 399.19, 399.67999, 400.17999, 400.67999, 401.17999, 401.67999, 402.17001, 402.67001, 403.17001, 403.66, 404.16, 404.66, 405.14999, 405.64999, 406.14999, 406.64001, 407.14001, 407.64001, 408.13, 408.63, 409.13, 409.62, 410.12, 410.62, 411.10999, 411.60999, 412.10001, 412.60001, 413.10001, 413.60001, 414.09, 414.59, 415.09, 415.59, 416.07999, 416.57999, 417.07999, 417.57999, 418.07999, 418.57999], [1.6483722836524246, 1.6546363395359365, 1.647298907653894, 1.6533287796168583, 1.6513909602141936, 1.6441728100483295, 1.6485630092327472, 1.6465913680498476, 1.644326968253007, 1.6458723273169005, 1.6423749873362237, 1.6435071871004756, 1.6412154858600103, 1.6396834087598822, 1.6391132715105765, 1.6382846511661762, 1.6358307684719318, 1.6354408519662669, 1.6334428509272396, 1.6328074965992703, 1.630211530333035, 1.629597879928187, 1.6276773015694914, 1.6248549924331006, 1.6221911228582016, 1.6131967111234533, 1.6094507790415067, 1.6108839833096118, 1.6122492163476982, 1.6122322997299472, 1.6077321043459216, 1.6138723793940135, 1.6118005408009028, 1.6157486465235684, 1.6147077896853421, 1.6142964675684908, 1.614804272990439, 1.6117647309822476, 1.6161328124848642, 1.6101356911507883, 1.612094662439775, 1.6118531546799915, 1.614236269971587, 1.6062328837497617, 1.6105586500151539, 1.6108228692284308, 1.6178782024106462, 1.6087987962691102, 1.6074587087659151, 1.6187364188290658, 1.6209092605148896, 1.6151493452793495, 1.6182798966697, 1.6109338276299237, 1.6085077651242317, 1.613655399235577, 1.612511934789509, 1.607851046633587, 1.6057532268507935, 1.6024870719133475, 1.6038884748636346, 1.605523559015856, 1.5960101592112506, 1.5997312604952778, 1.598377877440321, 1.597392154092918, 1.600589807386528, 1.5995684913350448, 1.5979434008328421, 1.5961998900762004, 1.5970150338732805, 1.5939307380342091, 1.596156816544494, 1.5962182334684933, 1.597512896681686, 1.595101996088882, 1.5933960300930927, 1.592688229676817, 1.5913322143224218, 1.5917530088094214, 1.591614538502429, 1.5914637114820218, 1.5878221602705458, 1.5928834293750267, 1.5915729711917386, 1.587309104722474, 1.5918112038963161, 1.5881066262119135, 1.584965267353939, 1.5914289179893895, 1.586911737372422, 1.581731065142223, 1.5886590769172397, 1.5849680475176062, 1.586099454232746, 1.581195601241917, 1.5854707251659343, 1.5865012245981702, 1.5838978086861526, 1.584800751487047, 1.5848505559733816, 1.5857486239152707, 1.585591816537336, 1.5810404634087085, 1.5851743649291072, 1.5859104770394237, 1.5823664432736304, 1.5792071958230995, 1.590530467368216, 1.5870072549949592]}] ("Real Part vs wavelength")
  n1 = call <vilib>:"Add State(s) to Queue__jki_lib_state_machine.vi"("State(s) in (\"\")"="Macro: Initialize") -> ("States Out"=w2:string)  [unwired: 14 in]
  n2 = while "JKI - String-Based Queued State Machine (Basic) v1.0" {
    shift-right: [w6] -> _
    shift-left: _ -> [w5]
    shift-right: [w9] -> _
    shift-left: _ -> [w3]
    shift-right: [w8] -> _
    shift-left: w2 -> [w10]
    stop <- w7 stop-if-true
    w4 = -1  # Timeout
    # "Template Copyright © 2008 JKI - http://jkisoft.com/state-machine"
    n3 = call <vilib>:"Parse State Queue__jki_lib_state_machine.vi"("State Queue"=w10, "Error In (no error)"=w3) -> ("Remaining States"=w12:string, "Current State"=w13:string, "Arguments"=w11:string)  [unwired: 11 in]
    n4 = case shown="\"Retrieve RI\"" w13 {
      selector: w13 -> [_ _ w171 _ _ _ _ _ _ _ _ _ _ _ _ _ _ _ _ _ _ _ _ _ _ _ _ _ _ _ _]
      tunnel: w12 -> [w20 w170 w175 w193 w199 w204 w208 w222 w228 w232 w237 w243 w254 w280 w285 w295 w299 w326 w362 w399 w413 w420 w473 w520 w646 w714 w793 w863 w965 w1117 w1195]
      tunnel: w11 -> [_ _ _ _ _ _ _ _ _ _ _ w238 w248 _ _ _ _ w309 _ _ _ w414 _ _ _ _ _ _ _ _ _]
      tunnel: w5 -> [w18 w167 w173 w184 w196 w202 w205 _ w223 w229 w235 w241 w250 w277 w282 w292 w296 w312 w359 w396 w410 w417 w470 w517 w644 w712 w791 w835 w940 w1114 w1153]
      tunnel: [w17 w168 w177 w190 errorcluster {"status"=FALSE, "code"=0, "source"=""} ("error out") w201 w206 w219 w224 w230 w234 w239 w251 w278 w283 w293 w297 w324 w360 w397 w411 w418 w471 w518 w643 w711 w790 w861 w963 w1115 w1193] -> w9
      tunnel: w3 -> [w16 w168 w176 w190 w195 w201 w206 w219 w225 w230 w234 w240 w252 w278 w283 w293 w297 w324 w360 w397 w411 w418 w471 w518 w643 w711 w790 w861 w963 w1115 w1193]
      tunnel: [w19 w169 w174 w192 w198 w203 w207 w221 w227 w231 w236 w242 w253 w279 w284 w294 w298 w325 w361 w398 w412 w419 w472 w519 w645 w713 w792 w862 w964 w1116 w1194] -> w8
      tunnel: [_ _ _ _ _ TRUE _ _ _ _ _ _ _ _ _ _ _ _ _ _ _ _ _ _ _ _ _ _ _ _ _] -> w7
      tunnel: [w15 w167 w173 w191 w196 w202 w205 w220 w223 w229 w235 w241 w250 w277 w282 w292 w296 w323 w358 w396 w409 w416 w469 w516 w644 w712 w791 w834 w939 w1114 w1152] -> w6
      tunnel: w4 -> [w14 _ _ _ _ _ _ _ _ _ _ _ _ _ _ _ _ _ _ _ _ _ _ _ _ _ _ _ _ _ _]
      frame "", "Idle" {
        # "executes when the state queue is empty"
        n5 = event shown="[7] \"Retrieve RI\": Value Change" {
          selector: _ -> [_ _ _ _ _ _ _ _ _ _ _ _ _ _ _ _ _ _ _ _ _ _]
          dyn-events: _ -> [_ _ _ _ _ _ _ _ _ _ _ _ _ _ _ _ _ _ _ _ _ _]
          timeout: w14 -> [_ _ _ _ _ _ _ _ _ _ _ _ _ _ _ _ _ _ _ _ _ _]
          tunnel: w20 -> [w24 w33 w53 w59 w65 w71 w76 w84 w90 w95 w100 w105 w110 w115 w120 w125 w132 w139 w147 w152 w160 w166]
          tunnel: [w23 w32 w52 w58 w64 w70 w75 w83 w89 w94 w99 w104 w109 w114 w119 w124 w131 w138 w146 w151 w159 w165] -> w19
          tunnel: w18 -> [w21 w30 w50 w56 w62 w68 w73 w81 w87 w92 w97 w102 w107 w112 w117 w122 w127 w134 w144 w149 w157 w163]
          tunnel: [w22 w31 w51 w57 w63 w69 w74 w82 w88 w93 w98 w103 w108 w113 w118 w123 w130 w137 w145 w150 w158 w164] -> w17
          tunnel: w16 -> [w22 w31 w51 w57 w63 w69 w74 w82 w88 w93 w98 w103 w108 w113 w118 w123 w130 w137 w145 w150 w158 w164]
          tunnel: [w21 w30 w50 w56 w62 w68 w73 w81 w87 w92 w97 w102 w107 w112 w117 w122 w126 w133 w144 w149 w157 w163] -> w15
          event Timeout {
            # "Timeout Frame\n(this will only execute if the Event Structure timeout is >= 0)"
            n6 = event-data() -> ()  [unwired: 1 in, 1 out]
            n7 = call <vilib>:"Add State(s) to Queue__jki_lib_state_machine.vi"("State(s) in (\"\")"=w24) -> ("States Out"=w23:string)  [unwired: 14 in]
          }
          event "Diameters to fit": Mouse Down {
            # "Timeout Frame\n(this will only execute if the Event Structure timeout is >= 0)"
            n8 = event-data() -> ("Coords"=w29:T13)  [unwired: 1 in, 7 out]
            n9 = case shown="True" "Quick Fit" {
              tunnel: ["" w36] -> w25
              frame False {
              }
              frame True {
                n10 = local read "Use Factors"() -> (w35:bool)
                n11 = Select(t="Load Files >> Dont Initialize Sizes\nRetrieve RI >> UseFactors", s=w35, f="Load Files >> Dont Initialize Sizes\nRetrieve RI >> DontUseFactors") -> (s? t:f=w36:string)
                n12 = case shown="True" w35 {
                  frame False {
                  }
                  frame True {
                    n13 = One Button Dialog(message="You are using Extinction factor and Diameter factors/offset in this calculation !!") -> ()  [unwired: 1 in, 1 out]
                  }
                }
              }
            }
            n14 = invoke on="Diameters to fit" class="LstBox (strict)" method="Point To Row"("Point"=w29) -> ("Row"=w28:i32, "InGlyph"=w27:bool)  [unwired: 6 in, 5 out]
            n15 = case shown="True" w27 {
              tunnel: w28 -> [_ w47]
              frame False {
              }
              frame True {
                w43 = 37 ("Item Symbols")
                n16 = property on="Diameters to fit" class="LstBox (strict)"() -> ("Item Symbols"=w40:i32[])  [unwired: 2 in, 2 out]
                n17 = Index Array(array=w40, index=w47) -> (element=w46:i32)
                n18 = Equal?(x=w46, y=w43) -> (x = y?=w45:bool)
                n19 = Select(t=38 ("Item Symbols"), s=w45, f=w43) -> (s? t:f=w44:i32)
                n20 = Replace Array Subset(array=w40, new element=w44, index=w47) -> (w41:i32[])
                n21 = property on="Diameters to fit" class="LstBox (strict)"("Item Symbols"=w41) -> ()  [unwired: 2 in, 2 out]
              }
            }
            n22 = call <vilib>:"Add State(s) to Queue__jki_lib_state_machine.vi"("State(s) in Front (\"\")"=w25, "State(s) in (\"\")"=w33) -> ("States Out"=w32:string)  [unwired: 13 in]
          }
          event "Diamter Offset Radio Button": Mouse Up {
            w48 = TRUE ("Diamter Offset Radio Button")
            # "Timeout Frame\n(this will only execute if the Event Structure timeout is >= 0)"
            n23 = event-data() -> ()  [unwired: 1 in, 8 out]
            n24 = local write "Diamter Offset Radio Button"(w48) -> ()
            n25 = local write "Diameter Factor Radio Button"(FALSE ("Diameter Factor Radio Button")) -> ()
            n26 = local write "Diameter Factor or Offset"(w48) -> ()
            n27 = call <vilib>:"Add State(s) to Queue__jki_lib_state_machine.vi"("State(s) in (\"\")"=w53) -> ("States Out"=w52:string)  [unwired: 14 in]
          }
          event "Diameter Factor Radio Button": Mouse Up {
            w54 = FALSE ("Diamter Offset Radio Button")
            # "Timeout Frame\n(this will only execute if the Event Structure timeout is >= 0)"
            n28 = event-data() -> ()  [unwired: 1 in, 8 out]
            n29 = local write "Diamter Offset Radio Button"(w54) -> ()
            n30 = local write "Diameter Factor Radio Button"(TRUE ("Diameter Factor Radio Button")) -> ()
            n31 = local write "Diameter Factor or Offset"(w54) -> ()
            n32 = call <vilib>:"Add State(s) to Queue__jki_lib_state_machine.vi"("State(s) in (\"\")"=w59) -> ("States Out"=w58:string)  [unwired: 14 in]
          }
          event "Imaginary Part vs wavelength": Cursor Move {
            # "Timeout Frame\n(this will only execute if the Event Structure timeout is >= 0)"
            n33 = event-data() -> ()  [unwired: 1 in, 9 out]
            n34 = property on="Imaginary Part vs wavelength" class="XYGraph (strict)"() -> ("Cursor.Cursor X"=w61:dbl)  [unwired: 2 in, 2 out]
            n35 = property on="Real Part vs wavelength" class="XYGraph (strict)"("Cursor.Cursor X"=w61) -> ()  [unwired: 2 in, 2 out]
            n36 = call <vilib>:"Add State(s) to Queue__jki_lib_state_machine.vi"("State(s) in Front (\"\")"="Update Corrected multiple charge extinction graph" ("State(s) in Front (\"\")"), "State(s) in (\"\")"=w65) -> ("States Out"=w64:string)  [unwired: 13 in]
          }
          event "Real Part vs wavelength": Cursor Move {
            n37 = event-data() -> ()  [unwired: 1 in, 9 out]
            n38 = property on="Real Part vs wavelength" class="XYGraph (strict)"() -> ("Cursor.Cursor X"=w67:dbl)  [unwired: 2 in, 2 out]
            n39 = property on="Imaginary Part vs wavelength" class="XYGraph (strict)"("Cursor.Cursor X"=w67) -> ()  [unwired: 2 in, 2 out]
            n40 = call <vilib>:"Add State(s) to Queue__jki_lib_state_machine.vi"("State(s) in Front (\"\")"="Update Corrected multiple charge extinction graph" ("State(s) in Front (\"\")"), "State(s) in (\"\")"=w71) -> ("States Out"=w70:string)  [unwired: 13 in]
          }
          event "OK": Value Change {
            # "Exit Button Value Change (pressed) Event\n(this executes Macro: Exit to terminate the VI)"
            n41 = event-data() -> ()  [unwired: 1 in, 1 out]
            n42 = call <vilib>:"Add State(s) to Queue__jki_lib_state_machine.vi"("State(s) in Front (\"\")"="Macro: Exit", "State(s) in (\"\")"=w76) -> ("States Out"=w75:string)  [unwired: 13 in]
          }
          event "Retrieve RI": Value Change {
            # "Exit Button Value Change (pressed) Event\n(this executes Macro: Exit to terminate the VI)"
            n43 = event-data() -> ()  [unwired: 1 in, 6 out]
            n44 = Select(t="Load Files >> Dont Initialize Sizes\nRetrieve RI >> UseFactors", s="Use Factors", f="Load Files >> Dont Initialize Sizes\nRetrieve RI >> DontUseFactors") -> (s? t:f=w80:string)
            n45 = case shown="False" "Use Factors" {
              frame False {
              }
              frame True {
                n46 = One Button Dialog(message="You are using Extinction factor and Diameter factors/offset in this calculation !!") -> ()  [unwired: 1 in, 1 out]
              }
            }
            n47 = call <vilib>:"Add State(s) to Queue__jki_lib_state_machine.vi"("State(s) in Front (\"\")"=w80, "State(s) in (\"\")"=w84) -> ("States Out"=w83:string)  [unwired: 13 in]
          }
          event "Retrieve RI Calculate lines seperately": Value Change {
            # "Exit Button Value Change (pressed) Event\n(this executes Macro: Exit to terminate the VI)"
            n48 = event-data() -> ()  [unwired: 1 in, 6 out]
            n49 = call <vilib>:"Add State(s) to Queue__jki_lib_state_machine.vi"("State(s) in Front (\"\")"="Load Files MC\nRetrieve RI", "State(s) in (\"\")"=w90) -> ("States Out"=w89:string)  [unwired: 13 in]
          }
          event "Retrieve RI without taking the mean (MC)": Value Change {
            # "Exit Button Value Change (pressed) Event\n(this executes Macro: Exit to terminate the VI)"
            n50 = event-data() -> ()  [unwired: 1 in, 6 out]
            n51 = call <vilib>:"Add State(s) to Queue__jki_lib_state_machine.vi"("State(s) in Front (\"\")"="Load Files MC\nRetreive RI from Single Measurements(MC)", "State(s) in (\"\")"=w95) -> ("States Out"=w94:string)  [unwired: 13 in]
          }
          event "Save RI": Value Change {
            # "Exit Button Value Change (pressed) Event\n(this executes Macro: Exit to terminate the VI)"
            n52 = event-data() -> ()  [unwired: 1 in, 6 out]
            n53 = call <vilib>:"Add State(s) to Queue__jki_lib_state_machine.vi"("State(s) in Front (\"\")"="Save RI to file", "State(s) in (\"\")"=w100) -> ("States Out"=w99:string)  [unwired: 13 in]
          }
          event "Save RI expanded Edition": Value Change {
            # "Exit Button Value Change (pressed) Event\n(this executes Macro: Exit to terminate the VI)"
            n54 = event-data() -> ()  [unwired: 1 in, 6 out]
            n55 = call <vilib>:"Add State(s) to Queue__jki_lib_state_machine.vi"("State(s) in Front (\"\")"="Save RI to File Expanded Edition", "State(s) in (\"\")"=w105) -> ("States Out"=w104:string)  [unwired: 13 in]
          }
          event "Find Extinction Factor Graph": Value Change {
            # "Exit Button Value Change (pressed) Event\n(this executes Macro: Exit to terminate the VI)"
            n56 = event-data() -> ()  [unwired: 1 in, 6 out]
            n57 = call <vilib>:"Add State(s) to Queue__jki_lib_state_machine.vi"("State(s) in Front (\"\")"="Load Files >> Dont Initialize Sizes\nFind Extinction Factor", "State(s) in (\"\")"=w110) -> ("States Out"=w109:string)  [unwired: 13 in]
          }
          event "Plot RI": Value Change {
            # "Exit Button Value Change (pressed) Event\n(this executes Macro: Exit to terminate the VI)"
            n58 = event-data() -> ()  [unwired: 1 in, 6 out]
            n59 = call <vilib>:"Add State(s) to Queue__jki_lib_state_machine.vi"("State(s) in Front (\"\")"="Append Mie Curve", "State(s) in (\"\")"=w115) -> ("States Out"=w114:string)  [unwired: 13 in]
          }
          event "Save RI MC": Value Change {
            # "Exit Button Value Change (pressed) Event\n(this executes Macro: Exit to terminate the VI)"
            n60 = event-data() -> ()  [unwired: 1 in, 6 out]
            n61 = call <vilib>:"Add State(s) to Queue__jki_lib_state_machine.vi"("State(s) in Front (\"\")"="Save RI -Monte Carlo to file", "State(s) in (\"\")"=w120) -> ("States Out"=w119:string)  [unwired: 13 in]
          }
          event "Retrieve RI (MC)": Value Change {
            # "Exit Button Value Change (pressed) Event\n(this executes Macro: Exit to terminate the VI)"
            n62 = event-data() -> ()  [unwired: 1 in, 6 out]
            n63 = call <vilib>:"Add State(s) to Queue__jki_lib_state_machine.vi"("State(s) in Front (\"\")"="Load Files\nRetrieve RI Monte Carlo", "State(s) in (\"\")"=w125) -> ("States Out"=w124:string)  [unwired: 13 in]
          }
          event "Extinction Cross Section File": Value Change {
            # "Exit Button Value Change (pressed) Event\n(this executes Macro: Exit to terminate the VI)"
            n64 = event-data() -> ()  [unwired: 1 in, 6 out]
            n65 = local read "Extinction Cross Section File"() -> (w128:path)
            n66 = Bundle By Name(cluster=w127, "Extinction Cross section Path"=w128) -> (w126:T15)
            n67 = call <vilib>:"Add State(s) to Queue__jki_lib_state_machine.vi"("State(s) in Front (\"\")"="Load Files >> Initialize Sizes\nUpdate Window after Load Files", "State(s) in (\"\")"=w132) -> ("States Out"=w131:string)  [unwired: 13 in]
          }
          event "Mutiple Charge Data File": Value Change {
            # "Exit Button Value Change (pressed) Event\n(this executes Macro: Exit to terminate the VI)"
            n68 = event-data() -> ()  [unwired: 1 in, 6 out]
            n69 = local read "Mutiple Charge Data File"() -> (w135:path)
            n70 = Bundle By Name(cluster=w134, "Multiple charge correction file Path"=w135) -> (w133:T15)
            n71 = call <vilib>:"Add State(s) to Queue__jki_lib_state_machine.vi"("State(s) in Front (\"\")"="Load Files\nUpdate Window after Load Files", "State(s) in (\"\")"=w139) -> ("States Out"=w138:string)  [unwired: 13 in]
          }
          event "Calculate Errors": Value Change {
            # "Exit Button Value Change (pressed) Event\n(this executes Macro: Exit to terminate the VI)"
            n72 = event-data() -> ("NewVal"=w143:bool)  [unwired: 1 in, 5 out]
            n73 = Select(t=FALSE, s=w143, f=FALSE) -> (s? t:f=w141:bool)
            n74 = property on="Approximate Errors" class="Bool (strict)"("Visible"=w143) -> ()  [unwired: 2 in, 2 out]
            n75 = property on="Approximate Errors" class="Bool (strict)"("Value"=w141) -> ()  [unwired: 2 in, 2 out]
            n76 = call <vilib>:"Add State(s) to Queue__jki_lib_state_machine.vi"("State(s) in (\"\")"=w147) -> ("States Out"=w146:string)  [unwired: 14 in]
          }
          event "ShiftSMPStoSizes": Value Change {
            # "Exit Button Value Change (pressed) Event\n(this executes Macro: Exit to terminate the VI)"
            n77 = event-data() -> ()  [unwired: 1 in, 6 out]
            n78 = call <vilib>:"Add State(s) to Queue__jki_lib_state_machine.vi"("State(s) in Front (\"\")"="ShiftSMPStoSizes" ("State(s) in Front (\"\")"), "State(s) in (\"\")"=w152) -> ("States Out"=w151:string)  [unwired: 13 in]
          }
          event "autoscale": Value Change {
            n79 = event-data() -> ()  [unwired: 1 in, 6 out]
            n80 = property on="Imaginary Part vs wavelength" class="XYGraph (strict)"("XScale.ScaleFit"=u8 1 ("X Scale.Scale Fit"), "YScale.ScaleFit"=u8 1 ("Y Scale.Scale Fit")) -> ()  [unwired: 2 in, 2 out]
            n81 = property on="Real Part vs wavelength" class="XYGraph (strict)"("XScale.ScaleFit"=u8 1 ("X Scale.Scale Fit"), "YScale.ScaleFit"=u8 1 ("Y Scale.Scale Fit")) -> ()  [unwired: 2 in, 2 out]
            n82 = call <vilib>:"Add State(s) to Queue__jki_lib_state_machine.vi"("State(s) in (\"\")"=w160) -> ("States Out"=w159:string)  [unwired: 14 in]
          }
          event Panel Close? {
            # "Discard the event because we'll close the front panel ourselves in Macro: Exit"
            # "Close Panel button (pressed) Event\n(this executes Macro: Exit to terminate the VI)"
            n83 = event-data() -> ()  [unwired: 1 in, 1 out]
            n84 = call <vilib>:"Add State(s) to Queue__jki_lib_state_machine.vi"("State(s) in Front (\"\")"="Macro: Exit", "State(s) in (\"\")"=w166) -> ("States Out"=w165:string)  [unwired: 13 in]
            n85 = event-data("Discard?"=TRUE) -> ()  [unwired: 1 in, 1 out]
          }
        }
      }
      frame "---------- Core ----------" {
        # "Do not put any code in this frame.\n(it is a separator no-op)"
        n86 = call <vilib>:"Add State(s) to Queue__jki_lib_state_machine.vi"("State(s) in (\"\")"=w170) -> ("States Out"=w169:string)  [unwired: 14 in]
      }
      frame Default {
        w180 = 42 items=["No error", "Argument error", "Memory is full", "Out of zone", "End of file", "File already open", "Generic file I/O error", "File not found", "File permission error", "Disk is full", "Duplicate path", "Too many files open", "System feature not enabled", "Resource file not found", "Cannot add resource", "Resource not found", "Image not found", "Image memory error", "Pen does not exist", "Config type invalid", "Config token not found", "Config parse error", "Config memory error", "Bad external code format", "Bad external code offset", "External code not present", "Null window", "Destroy window error", "Null menu", "Print aborted", "Bad print record", "Print driver error", "Windows error during printing", "Memory error during printing", "Print dialog error", "Generic print error", "Invalid device refnum", "Device not found", "Device parameter error", "Device unit error", "Cannot open device", "Device call aborted", "Generic error", "Cancelled by user", "Object ID too low", "Object ID too high", "Object not in heap", "Unknown heap", "Unknown object (invalid DefProc)", "Unknown object (DefProc not in table)", "Message out of range", "Invalid (null) method", "Unknown message", "Manager call not supported", "Bad address", "Network operation in progress", "Network operation timed out", "Connection is busy", "Network attribute not supported", "Network error", "Address in use", "System out of memory", "Connection aborted", "Connection refused", "Not connected", "Already connected", "Connection closed", "Initialization error (interapplication manager)", "Bad occurrence", "Wait on unbound occurrence handler", "Occurrence queue overflow", "Datalog type conflict", "Unused", "Unrecognized type (interapplication manager)", "Memory corrupt", "Failed to make temporary DLL", "Old CIN version", "Drag socket not found", "Failed to load drop-object", "Failed to register OLE object", "Failed to release OLE object", "Format specifier type mismatch", "Unknown format specifier", "Too few format specifiers", "Too many format specifiers", "Scan failed", "Newer CIN version", "Error converting to variant", "Runtime menu error", "Password tampered", "Variant attribute not found", "Incompatible variant data type", "Event data is not available", "Event Store is not present", "Occurrence is not found", "Event Queue is not created", "Event info is not available", "Refnum passed is NULL", "Error retrieving Class GUID", "Error retrieving CoClass GUID", "Error retrieving TypeLib GUID.", "Bad built application magic bytes.", "Specific driver is different from the specific driver associated with the Logical Name.", "There is no session opened to the class driver.", "Max Error", "MAX - Error with config objects", "MAX - Error loading configuration", "MAX - Group not supported"]
        # "Current State"
        # "Do not delete, rename, or modify this frame.\n(this is used to capture unhandled states and typos)"
        # "Handle mistyped state name (developer tool)"
        n87 = call <vilib>:"Add State(s) to Queue__jki_lib_state_machine.vi"("State(s) in (\"\")"=w175) -> ("States Out"=w174:string)  [unwired: 14 in]
        n88 = Format Into String(format string="Software Exception: Unhandled State \"%s\"." ("message"), error in=w176, w171) -> (resulting string=w179:string, error out=w178:errorcluster)  [unwired: 1 in]
        n89 = call <vilib>:"Error Cluster From Error Code.vi"("show call chain? (False)"=TRUE, "error in (no error)"=w178, "error message (\"\")"=w179, "error code (0)"=w180) -> ("error out"=w177:errorcluster)  [unwired: 5 in]
      }
      frame "Initialize Core Data" {
        # "Do not delete, rename, or modify this frame.\n(this is used to determine panel behavior on exit)"
        # "originally closed?"
        # "exe?"
        # "If panel starts closed or is an EXE, then close it when we exit"
        n90 = call <vilib>:"Add State(s) to Queue__jki_lib_state_machine.vi"("State(s) in (\"\")"=w193) -> ("States Out"=w192:string)  [unwired: 14 in]
        n91 = property class="App"() -> ("App.Kind"=w188:T9)  [unwired: 2 in, 2 out]
        n92 = property class="VI"() -> ("Front Panel.Open"=w189:bool)  [unwired: 2 in, 2 out]
        n93 = Equal?(x=w188, y=T9."Run Time System" ("Application:Kind")) -> (x = y?=w185:bool)
        n94 = Not(x=w189) -> (.not. x?=w186:bool)
        n95 = Or(x=w186, y=w185) -> (x .or. y?=w183:bool)
        n96 = control-ref of="Current VI Reference"() -> (w182:refnum<vi>)
        n97 = Bundle By Name(cluster=w184, "Core.Current VI Reference"=w182, "Core.Close Panel on Exit?"=w183) -> (w191:T15)
      }
      frame "Error Handler" {
        # "Unhandled Error -- Display it"
        # "Handle any errors here.\nYou can also output any states to clean-up after errors occur"
        # "Clear error"
        n98 = call <vilib>:"General Error Handler.vi"("error in (no error)"=w195) -> ()  [unwired: 10 in, 5 out]
        n99 = call <vilib>:"Add State(s) to Queue__jki_lib_state_machine.vi"("State(s) in Front (\"\")"="/* Post Error States", "State(s) in (\"\")"=w199) -> ("States Out"=w198:string)  [unwired: 13 in]
      }
      frame "Exit" {
        # "Do not put any code in this frame.\n(No errors that occur here will be handled.)"
        n100 = call <vilib>:"Add State(s) to Queue__jki_lib_state_machine.vi"("State(s) in (\"\")"=w204) -> ("States Out"=w203:string)  [unwired: 14 in]
      }
      frame "---------- Data ----------" {
        # "Do not put any code in this frame.\n(It is a separator no-op. You can make a copy of this frame to create a new Data frame)"
        n101 = call <vilib>:"Add State(s) to Queue__jki_lib_state_machine.vi"("State(s) in (\"\")"=w208) -> ("States Out"=w207:string)  [unwired: 14 in]
      }
      frame "Data: Initialize" {
        w210 = 0  # NumberOfMeasurementsperSize
        w211 = dbl[][] []  # FullExtinctionData
        w212 = path ""  # Multiple charge correction file Path
        w213 = path ""  # Extinction Cross section Path
        w214 = T14 {"Real RI"=[], "Imaginary RI"=[], "Std Imaginary RI"=[], "Std Real RI"=[], "Wavelength"=[], "Residue"=[], "Extinction Factor"=[], "Diameter Factor"=[], "Diameter Offset"=[], "Best fit result"=[], "Normalized Residuals"=[]}  # RI MC results
        w215 = T14 {"Real RI"=[], "Imaginary RI"=[], "Std Imaginary RI"=[], "Std Real RI"=[], "Wavelength"=[], "Residue"=[], "Extinction Factor"=[], "Diameter Factor"=[], "Diameter Offset"=[], "Best fit result"=[], "Normalized Residuals"=[]}  # RI results
        w216 = T6 {"SMPS Sizes"=[], "Concentration"=[], "Double Charge Correction Flag"=FALSE}  # Particle Distribution Data
        w217 = T5 {"Extinction"=[], "Extinction Uncertainty"=[], "Size parameters"=[], "Number ofSizes"=0.0, "GeometricCrossSection"=[], "WaveLength"=[], "Sizes"=[]}  # Extinction ExtinctionUncertainity Size parameter and Number ofS sizes
        w218 = T16 {"Current VI Reference"=refnum, "Close Panel on Exit?"=FALSE}  # Core
        # "do not delete - used by framework"
        # "Data names and types of shift register data are defined by this bundle."
        # "Initialize the shift-register data, here.\n(data names are defined by what you wire into the bundle function)"
        n102 = call <vilib>:"Add State(s) to Queue__jki_lib_state_machine.vi"("State(s) in (\"\")"=w222) -> ("States Out"=w221:string)  [unwired: 14 in]
        n103 = Bundle("Core"=w218, "Extinction ExtinctionUncertainity Size parameter and Number ofS sizes"=w217, "Particle Distribution Data"=w216, "RI results"=w215, "RI MC results"=w214, "Extinction Cross section Path"=w213, "Multiple charge correction file Path"=w212, "FullExtinctionData"=w211, "NumberOfMeasurementsperSize"=w210, "Baes data type definition"="Baes data type definition") -> (w220:T15)  [unwired: 1 in]
      }
      frame "Data: Cleanup" {
        # "Cleanup any data and references, here.\n(this is called automatically, by the Macro: Exit)"
        n104 = Unbundle By Name(w223) -> ("Core.Current VI Reference"=w226:refnum<vi>)
        n105 = call <vilib>:"Add State(s) to Queue__jki_lib_state_machine.vi"("State(s) in (\"\")"=w228) -> ("States Out"=w227:string)  [unwired: 14 in]
        n106 = Close Reference(reference=w226, error in (no error)=w225) -> (error out=w224:errorcluster)
      }
      frame "---------- UI ----------" {
        # "Do not put any code in this frame.\n(It is a separator no-op. You can make a copy of this frame to create a new UI frame)"
        n107 = call <vilib>:"Add State(s) to Queue__jki_lib_state_machine.vi"("State(s) in (\"\")"=w232) -> ("States Out"=w231:string)  [unwired: 14 in]
      }
      frame "UI: Initialize" {
        # "Initialize the User Interface, here.\n(this is called automatically, by the Macro: Init)"
        n108 = call <vilib>:"Add State(s) to Queue__jki_lib_state_machine.vi"("State(s) in (\"\")"=w237) -> ("States Out"=w236:string)  [unwired: 14 in]
        n109 = property on="Retrieve RI" class="Bool"("BoolText.Text"="Retrieve RI" ("Boolean Text.Text")) -> ()  [unwired: 2 in, 2 out]
      }
      frame "UI: Cursor Set" {
        # "Argument"
        # "Set and Unset Cursor Busy.\n(Usage: \"UI: Cursor Set >> Busy|Idle\")"
        n110 = call <vilib>:"Add State(s) to Queue__jki_lib_state_machine.vi"("State(s) in (\"\")"=w243) -> ("States Out"=w242:string)  [unwired: 14 in]
        n111 = case shown="\"Idle\", Default" w238 {
          tunnel: w240 -> [w245 w247]
          tunnel: [w244 w246] -> w239
          frame "Idle", Default {
            n112 = call <vilib>:"Unset Busy.vi"("error in (no error)"=w245) -> ("error out"=w244:errorcluster)  [unwired: 10 in]
          }
          frame "Busy" {
            n113 = call <vilib>:"Set Busy.vi"("error in (no error)"=w247) -> ("error out"=w246:errorcluster)  [unwired: 9 in, 1 out]
          }
        }
      }
      frame "UI: Front Panel State" {
        # "Argument"
        # "Set Front Panel Open or Closed\n(Usage: \"UI: Front Panel State >> Open|Close\")"
        n114 = Unbundle By Name(w250) -> ("Core.Current VI Reference"=w249:refnum<vi>)
        n115 = call <vilib>:"Add State(s) to Queue__jki_lib_state_machine.vi"("State(s) in (\"\")"=w254) -> ("States Out"=w253:string)  [unwired: 14 in]
        n116 = case shown="\"Open\", Default" w248 {
          tunnel: w252 -> [w258 w271]
          tunnel: [w260 w272] -> w251
          tunnel: w249 -> [w259 w269]
          frame "Open", Default {
            n117 = property class="VI"(reference=w259, error in=w258) -> (reference out=w256:refnum<vi>, error out=w257:errorcluster, "Front Panel.Open"=w255:bool)
            n118 = case shown="False" w255 {
              tunnel: [w263 w266] -> w260
              tunnel: w257 -> [w262 w266]
              tunnel: w256 -> [w261 _]
              frame False {
                n119 = invoke class="VI" method="FP.Open"(reference=w261, error in=w262, "Activate"=TRUE, "State"=T10."Standard") -> (error out=w263:errorcluster)  [unwired: 1 in, 4 out]
              }
              frame True {
              }
            }
          }
          frame "Close" {
            n120 = property class="VI"(reference=w269, error in=w271) -> (reference out=w268:refnum<vi>, error out=w270:errorcluster, "Front Panel.Open"=w267:bool)
            n121 = case shown="True" w267 {
              tunnel: [w273 w276] -> w272
              tunnel: w270 -> [w273 w275]
              tunnel: w268 -> [_ w274]
              frame False {
              }
              frame True {
                n122 = invoke class="VI" method="FP.Close"(reference=w274, error in=w275) -> (error out=w276:errorcluster)  [unwired: 1 in, 2 out]
              }
            }
          }
        }
      }
      frame "---------- Macro ----------" {
        # "Do not put any code in this frame.\n(It is a separator no-op. You can make a copy of this frame to create a new Macro frame)"
        n123 = call <vilib>:"Add State(s) to Queue__jki_lib_state_machine.vi"("State(s) in (\"\")"=w280) -> ("States Out"=w279:string)  [unwired: 14 in]
      }
      frame "Macro: Initialize" {
        w281 = "Data: Initialize\nInitialize Core Data\nUI: Initialize\nUI: Front Panel State >> Open"  # Data: Initialize Initialize Core Data UI: Initialize UI: Front Panel State >> Open
        # "Initialization Macro\n(This is called once, when the VI starts)"
        n124 = call <vilib>:"Add State(s) to Queue__jki_lib_state_machine.vi"("State(s) in Front (\"\")"=w281, "State(s) in (\"\")"=w285) -> ("States Out"=w284:string)  [unwired: 13 in]
      }
      frame "Macro: Exit" {
        # "Exit Macro\n(This is called once, when the VI exits)"
        n125 = Unbundle By Name(w292) -> ("Core.Close Panel on Exit?"=w291:bool)
        n126 = Select(t="UI: Front Panel State >> Close", s=w291, f="") -> (s? t:f=w288:string)
        n127 = call <vilib>:"Add State(s) to Queue__jki_lib_state_machine.vi"("State(s) in (\"\")"=w288, "State(s) at Back (\"\")"="Data: Cleanup\nExit") -> ("States Out"=w286:string)  [unwired: 13 in]
        n128 = call <vilib>:"Add State(s) to Queue__jki_lib_state_machine.vi"("State(s) in Front (\"\")"=w286, "State(s) in (\"\")"=w295) -> ("States Out"=w294:string)  [unwired: 13 in]
      }
      frame "---------- New Category ----------" {
        # "Template Separator\n(You can make a copy of, or modify, this frame)"
        n129 = call <vilib>:"Add State(s) to Queue__jki_lib_state_machine.vi"("State(s) in (\"\")"=w299) -> ("States Out"=w298:string)  [unwired: 14 in]
      }
      frame "Load Files" {
        n130 = call <vilib>:"Add State(s) to Queue__jki_lib_state_machine.vi"("State(s) in (\"\")"=w326) -> ("States Out"=w325:string)  [unwired: 14 in]
        n131 = Unbundle By Name(w312) -> ("Extinction Cross section Path"=w311:path, "Multiple charge correction file Path"=w310:path)
        n132 = call "ReadBAESdataFromFileVer3.vi"("Factor Size Parameter"=1.0, "Factor Extinction"="Extinction Factor in Data", "Factor Ext Uncertainty"="Factor Ext Uncertainty in Data", "file path"=w311) -> ("Extinction data in graph format"=→"Extinction Data per size":T17, "Extinction ExtinctionUncertainity Size parameter and Number ofS sizes"=w305:T5)
        n133 = call "ReadParticleSizeSpectrum.vi"("file path"=w310, "Factor Size paramter"=1.0) -> ("Particle Distribution Data"=w306:T6)  [unwired: 1 out]
        n134 = Strip Path(path=w311) -> (stripped path=w314:path, name=w318:string)
        n135 = Strip Path(path=w310) -> (stripped path=w313:path, name=w316:string)
        n136 = case shown="\"Initialize Sizes\"" w309 {
          tunnel: w305 -> [_ w344 _]
          frame "False", Default {
          }
          frame "Initialize Sizes" {
            n137 = Unbundle By Name(w344) -> ("Number ofSizes"=w343:dbl, "Sizes"=w342:dbl[])
            n138 = for {
              N: w343 -> [_]
              tunnel: [w349] -> w345 mode=indexing
              tunnel: w342 -> [w348] mode=indexing
              n139 = Number To Decimal String(number=w348) -> (decimal integer string=w349:string)  [unwired: 1 in]
            }
            n140 = Initialize Array(38 ("Item Symbols"), w343) -> (w346:i32[])
            n141 = property on="Diameters to fit" class="LstBox (strict)"("Item Symbols"=w346, "Item Names"=w345) -> ()  [unwired: 2 in, 2 out]
          }
          frame "Dont Initialize Sizes" {
          }
        }
        n142 = property on="Extinction Cross Section File" class="Path"("StartPath"=w314) -> ()  [unwired: 2 in, 2 out]
        n143 = property on="Mutiple Charge Data File" class="Path"("StartPath"=w313) -> ()  [unwired: 2 in, 2 out]
        n144 = case shown="True" "Correct SMPS sizes to selected Sizes" {
          tunnel: [w332 w334] -> w304
          tunnel: w306 -> [w332 w337]
          tunnel: w305 -> [_ w339]
          frame False {
          }
          frame True {
            n145 = Unbundle By Name(w337) -> ("Concentration"=w341:dbl[][], "SMPS Sizes"=w340:dbl[])
            n146 = Unbundle By Name(w339) -> ("Sizes"=w338:dbl[])
            n147 = call "Find and Shift SMPS sizes according to selected Peak Position.vi"("Sizes"=w338, "SMPS Sizes"=w340, "Concentration"=w341, "method"=3) -> ("SMPS sizes"=w335:dbl[], "Shifted Concentration"=w336:dbl[][])  [unwired: 5 in, 1 out]
            n148 = Bundle By Name(cluster=w337, "Concentration"=w336, "SMPS Sizes"=w335) -> (w334:T6)
          }
        }
        n149 = Unbundle By Name(w304) -> ("SMPS Sizes"=w303:dbl[], "Concentration"=w302:dbl[][])
        n150 = Bundle By Name(cluster=w312, "Extinction ExtinctionUncertainity Size parameter and Number ofS sizes"=w305, "Particle Distribution Data"=w304) -> (w323:T15)
        n151 = for {
          tunnel: w303 -> [w329]
          tunnel: w302 -> [w328] mode=indexing
          shift-right: [w331] -> w300
          shift-left: T11 [] -> [w330]
          n152 = Bundle("SMPS Sizes"=w329, "Concentration"=w328) -> (w327:T18)  [unwired: 1 in]
          n153 = Build Array (concatenate)(w330, w327) -> (w331:T11)
        }
        "Size Distribution" <- w300
        n154 = String To Path(string=w318) -> (path=w317:path)
        n155 = String To Path(string=w316) -> (path=w315:path)
        n156 = local write "Extinction Cross Section File"(w317) -> ()
        n157 = local write "Mutiple Charge Data File"(w315) -> ()
      }
      frame "ShiftSMPStoSizes" {
        n158 = call <vilib>:"Add State(s) to Queue__jki_lib_state_machine.vi"("State(s) in (\"\")"=w362) -> ("States Out"=w361:string)  [unwired: 14 in]
        n159 = Unbundle By Name(w359) -> ("Particle Distribution Data.Concentration"=w355:dbl[][], "Particle Distribution Data.SMPS Sizes"=w354:dbl[], "Extinction ExtinctionUncertainity Size parameter and Number ofS sizes.Sizes"=w356:dbl[])
        n160 = call "Find and Shift SMPS sizes according to selected Peak Position.vi"("Sizes"=w356, "SMPS Sizes"=w354, "Concentration"=w355, "method"="method") -> ("Peak Position in the old data"=→"Peak Center":dbl[], "SMPS sizes"=w357:dbl[], "Shifted Concentration"=w351:dbl[][])  [unwired: 5 in]
        n161 = Transpose Matrix(1:w351) -> (0:→"yi out":dbl[][])
        n162 = for {
          tunnel: w351 -> [w369] mode=indexing
          tunnel: w357 -> [w368]
          tunnel: w355 -> [w367] mode=indexing
          tunnel: w354 -> [w366]
          n163 = Bundle("SMPS sizes"=w368, "Shifted Concentration"=w369) -> (w365:T19)  [unwired: 1 in]
          n164 = Bundle("SMPS Sizes"=w366, "Concentration"=w367) -> (w364:T18)  [unwired: 1 in]
          n165 = Build Array(w365, w364) -> (→"SMPS":T11)
        }
        n166 = Bundle By Name(cluster=w359, "Particle Distribution Data.Concentration"=w351, "Particle Distribution Data.SMPS Sizes"=w357) -> (w358:T15)
      }
      frame "Append Mie Curve" {
        # "Calculate\nThe correction\nfor tested n and k"
        n167 = call <vilib>:"Add State(s) to Queue__jki_lib_state_machine.vi"("State(s) in (\"\")"=w399) -> ("States Out"=w398:string)  [unwired: 14 in]
        n168 = disable-structure shown="Disabled" {
          frame Disabled {
            n169 = control-ref of="Real Part vs wavelength"() -> (w401:refnum<vi>)
            n170 = control-ref of="Imaginary Part vs wavelength"() -> (w400:refnum<vi>)
            n171 = property on="Property Node" class="XYGraph (strict)" props=["Cursor", "Cursor Y"](reference=w401) -> ()  [unwired: 1 in, 3 out]
            n172 = property on="Property Node" class="XYGraph (strict)" props=["Cursor", "Cursor Y"](reference=w400) -> ()  [unwired: 1 in, 3 out]
          }
          frame Enabled {
          }
        }
        n173 = Unbundle By Name(w396) -> ("Baes data type definition"=w378:T8, "Baes data type definition.Extinction"=w379:dbl[], "Baes data type definition.Extinction Uncertainty"=w382:dbl[], "Baes data type definition.Number ofSizes"=w381:dbl)
        n174 = property on="Corrected for multiple charge particles" class="XYGraph (strict)"() -> ("Value"=w393:cluster{"Size parameters":dbl[], dbl[]}[])  [unwired: 2 in, 2 out]
        n175 = call "CalculateExtinctionCorrectionsToDoublyChargeParticleContribution.vi"("refractive index, imaginary"="k", "refractive index, real"="n", "Extinction ExtinctionUncertainity Size parameter and Number ofS sizes"=w378) -> ("Expected Extinction Cross Section"=w380:sgl[])  [unwired: 1 out]
        n176 = call "CalculateAreaOfFirstPeakofSizeDistribution.vi"("Extinction ExtinctionUncertainity Size parameter and Number ofS sizes"=w378) -> ("Area of First peak"=w376:dbl[])
        n177 = Subtract(x=w379, y=w380) -> (x-y=w377:dbl[])
        n178 = call "PlotMieCurve.vi"("refractive index, imaginary"="k", "refractive index, real"="n", "Use Extinction Factor"=FALSE, "Extinction ExtinctionUncertainity Size parameter and Number ofS sizes"=w378) -> ("Mie Results In Size Parameters"=w383:sgl[], "Size parameters"=w395:dbl[], "Extinction Crosssections"=w394:dbl[])
        n179 = Divide(x=w377, y=w376) -> (x/y=w375:dbl[])
        n180 = Subtract(x=w375, y=w383) -> (x-y=w385:dbl[])
        n181 = Bundle("Size parameters"=w395, "Extinction Crosssections"=w394) -> (w392:T20)  [unwired: 1 in]
        n182 = Divide(x=w385, y=w382) -> (x/y=w384:dbl[])
        n183 = Build Array (concatenate)(w393, w392) -> (w390:T21)
        n184 = Square(x=w384) -> (x^2=w374:dbl[])
        n185 = Array Size(array=w390) -> (size(s)=w389:i32)
        n186 = Add Array Elements(numeric array=w374) -> (sum=w373:dbl)
        n187 = Subtract(x=w389, y=1) -> (x-y=w387:i32)
        n188 = Divide(x=w373, y=w381) -> (x/y=→"Residue":dbl)
        n189 = property on="Corrected for multiple charge particles" class="XYGraph (strict)"("Value"=w390, "Active Plot"=w387, "Plot.Plot Color"=u32 0) -> ()  [unwired: 2 in, 2 out]
      }
      frame "Load Files MC" {
        # "Loading files for Monte Carlo simulation for the purpoese of error analysis"
        n190 = call <vilib>:"Add State(s) to Queue__jki_lib_state_machine.vi"("State(s) in (\"\")"=w413) -> ("States Out"=w412:string)  [unwired: 14 in]
        n191 = local read "Extinction Cross Section File"() -> (w406:path)
        n192 = local read "Mutiple Charge Data File"() -> (w405:path)
        n193 = local read "Diameter Factor"() -> (w402:dbl)
        n194 = call "ReadParticleSizeSpectrum.vi"("file path"=w405, "Factor Size paramter"=w402) -> ("Particle Distribution Data"=w407:T6)  [unwired: 1 out]
        n195 = call "ReadBAESdataFromFileMCVersion.vi"("file path"=w406) -> ("Extinction ExtinctionUncertainity Size parameter and Number ofS sizes"=w408:T5, "FullExtinctionData"=w404:dbl[][], "NumberOfMeasurementsperSize"=w403:i32)
        n196 = Bundle By Name(cluster=w410, "Extinction ExtinctionUncertainity Size parameter and Number ofS sizes"=w408, "Particle Distribution Data"=w407, "Extinction Cross section Path"=w406, "Multiple charge correction file Path"=w405, "FullExtinctionData"=w404, "NumberOfMeasurementsperSize"=w403) -> (w409:T15)
      }
      frame "Retrieve RI" {
        n197 = stacked-sequence {
          tunnel: w417 -> [w448 _]
          tunnel: [w450 _] -> w416
          tunnel: w414 -> [w430 _]
          frame #0 {
            n198 = case shown="\"UseFactors\"" w430 {
              tunnel: [1.0 ("Extinction Factor") "Extinction Factor"] -> w433
              tunnel: [1.0 ("Diameter Factor") "Diameter Factor"] -> w432
              tunnel: [0.0 ("Diameter Offset") "Diameter Offset"] -> w431
              frame "DontUseFactors", Default {
              }
              frame "UseFactors" {
              }
            }
            n199 = property on="Diameters to fit" class="LstBox (strict)"() -> ("Item Symbols"=w429:i32[])  [unwired: 2 in, 2 out]
            n200 = for {
              tunnel: w429 -> [w459] mode=indexing
              tunnel: 38 ("Item Symbols") -> [w458]
              tunnel: [w457] -> w427 mode=indexing
              n201 = Equal?(x=w459, y=w458) -> (x = y?=w457:bool)
            }
            n202 = property on="Max Wavelength" class="CmbBox"() -> ("Value"=w441:string)  [unwired: 2 in, 2 out]
            n203 = property on="Min Wavelength" class="CmbBox"() -> ("Value"=w442:string)  [unwired: 2 in, 2 out]
            n204 = property on="Retrieve RI" class="Bool"("BoolText.Text"="Running...." ("Boolean Text.Text")) -> ()  [unwired: 2 in, 2 out]
            n205 = Unbundle By Name(w448) -> ("Extinction ExtinctionUncertainity Size parameter and Number ofS sizes"=w425:T5, "Particle Distribution Data"=w426:T6)
            n206 = Decimal String To Number(string=w442) -> (number=w440:i32)  [unwired: 2 in, 1 out]
            n207 = Decimal String To Number(string=w441) -> (number=w439:i32)  [unwired: 2 in, 1 out]
            n208 = local read "General Data for RI Retrieval VI"() -> (w435:T3)
            n209 = local read "ExtinctionOrAbsorptionOrScattering"() -> (w422:i8)
            n210 = control-ref of="Real Part vs wavelength"() -> (w456:refnum<vi>)
            n211 = control-ref of="Not Corrected for Multiple charge Best fit result"() -> (w454:refnum<vi>)
            n212 = control-ref of="Imaginary Part vs wavelength"() -> (w455:refnum<vi>)
            n213 = control-ref of="Normalized Residuals vs Size parameter"() -> (w453:refnum<vi>)
            n214 = control-ref of="Simplex"() -> (w434:refnum<vi>)
            n215 = local read "Approximate Errors"() -> (w446:bool)
            n216 = Bundle("Real Part vs wavelength"=w456, "Imaginary Part vs wavelength"=w455, "Normalized Residuals vs Size parameter"=w453, "Not Corrected for Multiple charge Best fit result"=w454, "Simplex"=w434) -> (w452:T22)  [unwired: 1 in]
            n217 = Bundle By Name(cluster=w435, "Min WaveLength Index"=w440, "Max WaveLength Index"=w439, "Extinction Factor"="Extinction Factor", "Size Parameter Factor"="Size Parameter Factor", "Size Paramter Offset"="Size Parameter Offset", "Extinction Factor"=w433, "Diameter Factor"=w432, "Diameter Offset"=w431, "ExtinctionOrAbsorptionOrScattering"=w422) -> (w451:T3)
            n218 = call "RestructureDataAccordingToSelectedSizes.vi"("Extinction Data input"=w425, "Particle Distribution input"=w426, "Sizes to Fit"=w427) -> ("Extinciton Data ouput"=w424:T5, "Particle Distribution output"=w423:T6)
            n219 = call "RIRetrieval.vi"("General Data for RI Retrieval VI"=w451, "Approximate Errors"=w446, "Restrict to Positive Imaginary Part"="Restrict to Positive Imaginary Part", "Extinction Measured Data"=w424, "Calculate Errors"="Calculate Errors", "Particle Distribution Data"=w423, "Graph Refs"=w452, "Minimization method"="Minimization method") -> ("All Input data in one Cluster"=w443:T8, "RI results"=w449:T14)  [unwired: 2 out]
            n220 = Bundle By Name(cluster=w448, "RI results"=w449, "Baes data type definition"=w443, "Extinction ExtinctionUncertainity Size parameter and Number ofS sizes"=w424, "Particle Distribution Data"=w423) -> (w450:T15)
          }
          frame #1 {
            n221 = disable-structure shown="Disabled" {
              frame Disabled {
                n222 = One Button Dialog(message="RI retrieval finished successfully") -> ()  [unwired: 1 in, 1 out]
              }
              frame Enabled {
              }
            }
            n223 = property on="Retrieve RI" class="Bool"("BoolText.Text"="Retrieve RI" ("Boolean Text.Text")) -> ()  [unwired: 2 in, 2 out]
          }
        }
        n224 = call <vilib>:"Add State(s) to Queue__jki_lib_state_machine.vi"("State(s) in Front (\"\")"="Update Corrected multiple charge extinction graph" ("State(s) in Front (\"\")"), "State(s) in (\"\")"=w420) -> ("States Out"=w419:string)  [unwired: 13 in]
      }
      frame "Find Extinction and Size Parameter Factor" {
        n225 = stacked-sequence {
          tunnel: w470 -> [w507 _]
          tunnel: [w509 _] -> w469
          frame #0 {
            # "Real"
            n226 = property on="Max Wavelength" class="CmbBox"() -> ("Value"=w504:string)  [unwired: 2 in, 2 out]
            n227 = property on="Min Wavelength" class="CmbBox"() -> ("Value"=w505:string)  [unwired: 2 in, 2 out]
            n228 = local read "General Data for RI Retrieval VI"() -> (w476:T3)
            n229 = local read "Size Parameter Factor"() -> (w479:bool)
            n230 = local read "Size Parameter Offset"() -> (w478:bool)
            n231 = Decimal String To Number(string=w505) -> (number=w503:i32)  [unwired: 2 in, 1 out]
            n232 = Decimal String To Number(string=w504) -> (number=w502:i32)  [unwired: 2 in, 1 out]
            n233 = control-ref of="Simplex"() -> (w475:refnum<vi>)
            n234 = local read "Extinction Factor"() -> (w480:bool)
            n235 = control-ref of="Real Part vs wavelength"() -> (w513:refnum<vi>)
            n236 = control-ref of="Not Corrected for Multiple charge Best fit result"() -> (w511:refnum<vi>)
            n237 = control-ref of="Imaginary Part vs wavelength"() -> (w512:refnum<vi>)
            n238 = control-ref of="Normalized Residuals vs Size parameter"() -> (w510:refnum<vi>)
            n239 = Unbundle By Name(w507) -> ("Extinction ExtinctionUncertainity Size parameter and Number ofS sizes"=w500:T5, "Particle Distribution Data"=w498:T6)
            n240 = Bundle By Name(cluster=w476, "Min WaveLength Index"=w503, "Max WaveLength Index"=w502, "Extinction Factor"=w480, "Size Parameter Factor"=w479, "Size Paramter Offset"=w478, "ExtinctionOrAbsorptionOrScattering"="ExtinctionOrAbsorptionOrScattering") -> (w477:T3)
            n241 = Bundle(cluster="Graph Refs", "Real Part vs wavelength"=w513, "Imaginary Part vs wavelength"=w512, "Normalized Residuals vs Size parameter"=w510, "Not Corrected for Multiple charge particles"=w511, "Simplex 2"=w475) -> (w493:T4)
            n242 = local read "Restrict to Positive Imaginary Part"() -> (w496:bool)
            n243 = local read "Minimization method"() -> (w499:u16)
            n244 = local read "Approximate Errors"() -> (w501:bool)
            n245 = local read "Calculate Errors"() -> (w497:bool)
            n246 = Bundle(cluster="Data for RIRetrieval VI", "Approximate Errors"=w501, "Extinction ExtinctionUncertainity Size parameter and Number ofS sizes"=w500, "Minimization method"=w499, "Graph Ref"=w493, "Particle Distribution Data"=w498, "Calculate Errors"=w497, "Restrict to Positive Imaginary Part"=w496, "MinMaxWavelength"=w477) -> (w486:T7)
            n247 = call "RIRetrieval.vi"("General Data for RI Retrieval VI"=w477, "Approximate Errors"=w501, "Restrict to Positive Imaginary Part"=w496, "Extinction Measured Data"=w500, "Calculate Errors"=w497, "Particle Distribution Data"=w498, "Graph Refs"=w493, "Minimization method"=w499) -> ("All Input data in one Cluster"=w506:T8, "RI results"=w508:T14)  [unwired: 2 out]
            n248 = Bundle By Name(cluster=w507, "RI results"=w508, "Baes data type definition"=w506) -> (w509:T15)
            n249 = To Variant(anything=w486) -> (Variant=w490:variant)
            n250 = vi-ref "FindExtinctionAndSizeParameterFactors.vi"() -> (w489:refnum<vi>)
            n251 = Build Array(5.0 ("element"), 5.0 ("element")) -> (w492:dbl[])
            n252 = call-poly <vilib>:"Unconstrained Optimization.vi"("function data"=w490, "objective function"=w489, "stopping criteria"=T12 {"function tolerance"=0.01, "parameter tolerance"=0.05, "max iterations"=10, "max function calls"=1000, "gradient tolerance"=1000000.0, "max time (sec)"=-1.0}, "start"=w492) -> ("minimum"=w482:dbl[])  [unwired: 4 in, 3 out]
            n253 = Index Array(array=w482, index=0) -> (element=→"Minimized Extinction Factor":dbl)
            n254 = Index Array(array=w482, index=0) -> (element=→"Minimized Size Parameter Factor":dbl)
          }
          frame #1 {
            n255 = One Button Dialog(message="RI retrieval finished successfully") -> ()  [unwired: 1 in, 1 out]
          }
        }
        n256 = call <vilib>:"Add State(s) to Queue__jki_lib_state_machine.vi"("State(s) in Front (\"\")"="Update Corrected multiple charge extinction graph" ("State(s) in Front (\"\")"), "State(s) in (\"\")"=w473) -> ("States Out"=w472:string)  [unwired: 13 in]
      }
      frame "Find Extinction Factor" {
        n257 = stacked-sequence {
          tunnel: w517 -> [w526 _]
          tunnel: [w555 _] -> w516
          frame #0 {
            n258 = Subtract(x="Diameter FO Finish", y="Diameter FO start") -> (x-y=w550:dbl)
            n259 = Divide(x=w550, y="Diameter FO Interval") -> (x/y=w548:dbl)
            n260 = Round To Nearest(number=w548) -> (nearest integer value=w547:dbl)
            n261 = Increment(x=w547) -> (x+1=w546:dbl)
            n262 = call-poly <vilib>:"Ramp Pattern.vi"("start"="Diameter FO start", "end"="Diameter FO Finish", "samples"=w546) -> ("Ramp Pattern"=w530:dbl[])  [unwired: 7 in, 1 out]
            n263 = Tick Count (ms)() -> (millisecond timer value=w529:u32)
            n264 = property on="Diameters to fit" class="LstBox (strict)"() -> ("Item Symbols"=w528:i32[])  [unwired: 2 in, 2 out]
            n265 = for {
              tunnel: w528 -> [w558] mode=indexing
              tunnel: 38 ("Item Symbols") -> [w557]
              tunnel: [w556] -> w523 mode=indexing
              n266 = Equal?(x=w558, y=w557) -> (x = y?=w556:bool)
            }
            n267 = Unbundle By Name(w526) -> ("Particle Distribution Data"=w525:T6, "Extinction ExtinctionUncertainity Size parameter and Number ofS sizes"=w524:T5)
            n268 = call "RestructureDataAccordingToSelectedSizes.vi"("Extinction Data input"=w524, "Particle Distribution input"=w525, "Sizes to Fit"=w523) -> ("Extinciton Data ouput"=w521:T5, "Particle Distribution output"=w522:T6)
            n269 = for {
              tunnel: [w588] -> w554
              tunnel: w526 -> [w587]
              tunnel: [w586] -> w553
              tunnel: w530 -> [w579] mode=indexing
              tunnel: [w578] -> w533 mode=indexing
              tunnel: [w576] -> _
              tunnel: ["Extinction Factor Start"] -> _
              tunnel: [w567] -> w531
              tunnel: w530 -> [w568]
              tunnel: w529 -> [w566]
              tunnel: w522 -> [w560]
              tunnel: w521 -> [w559]
              i -> [w564]
              n270 = Subtract(x="Extinction Factor Finish", y="Extinction Factor Start") -> (x-y=w573:dbl)
              n271 = Divide(x=w573, y="Extinction Factor Interval") -> (x/y=w571:dbl)
              n272 = Array Size(array=w568) -> (size(s)=w563:i32)
              n273 = Round To Nearest(number=w571) -> (nearest integer value=w570:dbl)
              n274 = Subtract(x="Extinction Factor Finish", y="Extinction Factor Start") -> (x-y=w577:dbl)
              n275 = Increment(x=w570) -> (x+1=w569:dbl)
              n276 = Divide(x=w577, y=w569) -> (x/y=w576:dbl)
              n277 = call-poly <vilib>:"Ramp Pattern.vi"("start"="Extinction Factor Start", "end"="Extinction Factor Finish", "samples"=w569) -> ("Ramp Pattern"=w567:dbl[])  [unwired: 7 in, 1 out]
              n278 = Array Size(array=w567) -> (size(s)=w561:i32)
              n279 = control-ref of="Progress bar for Extinction search"() -> (w565:refnum<vi>)
              n280 = Multiply(x=w563, y=w561) -> (x*y=w562:i32)
              n281 = for {
                tunnel: [w623] -> w588
                tunnel: w587 -> [_]
                tunnel: [w638] -> w586
                tunnel: w567 -> [w624] mode=indexing
                tunnel: [w619] -> w585 mode=indexing
                tunnel: [w618] -> w584 mode=indexing
                tunnel: [w617] -> w578 mode=indexing
                tunnel: w579 -> [w611]
                shift-right: [w595] -> _
                shift-left: w566 -> [w603]
                tunnel: w564 -> [_]
                tunnel: w565 -> [w601]
                tunnel: w564 -> [w598]
                tunnel: w562 -> [w594]
                tunnel: w561 -> [w591]
                tunnel: w560 -> [w590]
                tunnel: w559 -> [w589]
                i -> [w602]
                n282 = local read "Size Parameter Factor"() -> (w628:bool)
                n283 = local read "Size Parameter Offset"() -> (w627:bool)
                n284 = local read "Extinction Factor"() -> (w629:bool)
                n285 = property on="Max Wavelength" class="CmbBox"() -> ("Value"=w636:string)  [unwired: 2 in, 2 out]
                n286 = property on="Min Wavelength" class="CmbBox"() -> ("Value"=w637:string)  [unwired: 2 in, 2 out]
                n287 = Decimal String To Number(string=w637) -> (number=w635:i32)  [unwired: 2 in, 1 out]
                n288 = Decimal String To Number(string=w636) -> (number=w634:i32)  [unwired: 2 in, 1 out]
                n289 = Select(t=w611, s="Diameter Factor or Offset", f=0.0) -> (s? t:f=w613:dbl)
                n290 = Select(t=1.0 ("Diameter Factor"), s="Diameter Factor or Offset", f=w611) -> (s? t:f=w609:dbl)
                n291 = Tick Count (ms)() -> (millisecond timer value=w595:u32)
                n292 = Bundle By Name(cluster="General Data for RI Retrieval VI", "Min WaveLength Index"=w635, "Max WaveLength Index"=w634, "Extinction Factor"=w629, "Size Parameter Factor"=w628, "Size Paramter Offset"=w627, "Extinction Factor"=w624, "Diameter Offset"=w613, "Diameter Factor"=w609) -> (w626:T3)
                n293 = Subtract(x=w595, y=w603) -> (x-y=w604:u32)
                n294 = Multiply(x=w591, y=w598) -> (x*y=w597:i32)
                n295 = control-ref of="Real Part vs wavelength"() -> (w642:refnum<vi>)
                n296 = control-ref of="Not Corrected for Multiple charge Best fit result"() -> (w640:refnum<vi>)
                n297 = control-ref of="Imaginary Part vs wavelength"() -> (w641:refnum<vi>)
                n298 = control-ref of="Normalized Residuals vs Size parameter"() -> (w639:refnum<vi>)
                n299 = control-ref of="Simplex"() -> (w608:refnum<vi>)
                n300 = Increment(x=w602) -> (x+1=w596:i32)
                n301 = Add(x=w597, y=w596) -> (x+y=w593:i32)
                n302 = Subtract(x=w594, y=w593) -> (x-y=w592:i32)
                n303 = property class="Slide (strict)"(reference=w601, "Value"=w593) -> ()  [unwired: 1 in, 2 out]
                n304 = Bundle(cluster="Graph Refs 2", "Real Part vs wavelength"=w642, "Imaginary Part vs wavelength"=w641, "Normalized Residuals vs Size parameter"=w639, "Not Corrected for Multiple charge particles"=w640, "Simplex 2"=w608) -> (w630:T4)
                n305 = local read "Restrict to Positive Imaginary Part"() -> (w632:bool)
                n306 = Divide(x=w604, y=u32 60000) -> (x/y=w600:dbl)
                n307 = Multiply(x=w600, y=w592) -> (x*y=→"Time Left (min)":dbl)
                n308 = local read "Minimization method"() -> (w633:u16)
                n309 = local read "Max Wavelength"() -> (w616:string)
                n310 = call "RIRetrieval.vi"("General Data for RI Retrieval VI"=w626, "Approximate Errors"=FALSE, "Restrict to Positive Imaginary Part"=w632, "Extinction Measured Data"=w589, "Calculate Errors"=FALSE, "Particle Distribution Data"=w590, "Graph Refs"=w630, "Minimization method"=w633) -> ("All Input data in one Cluster"=w638:T8, "RI results"=w623:T14)  [unwired: 2 out]
                n311 = Unbundle By Name(w623) -> ("Real RI"=w622:dbl[], "Imaginary RI"=w621:dbl[], "Residue"=w620:dbl[])
                n312 = Decimal String To Number(string=w616) -> (number=w615:i32)  [unwired: 2 in, 1 out]
                n313 = Index Array(array=w622, index=w615) -> (element=w619:dbl)
                n314 = Index Array(array=w621, index=w615) -> (element=w618:dbl)
                n315 = Index Array(array=w620, index=w615) -> (element=w617:dbl)
              }
              n316 = property class="Slide (strict)"(reference=w565, "Scale.Maximum"=w562) -> ()  [unwired: 1 in, 2 out]
              n317 = Bundle("Ramp Pattern"=w567, w585) -> (w583:cluster{"Ramp Pattern":dbl[], dbl[]})  [unwired: 1 in]
              n318 = Bundle("Ramp Pattern"=w567, w584) -> (w582:cluster{"Ramp Pattern":dbl[], dbl[]})  [unwired: 1 in]
              n319 = Bundle("Ramp Pattern"=w567, w578) -> (w581:cluster{"Ramp Pattern":dbl[], dbl[]})  [unwired: 1 in]
              n320 = Build Array(w583, w582, w581) -> (→"Extinction Factor Results":cluster{"Ramp Pattern":dbl[], dbl[]}[])
            }
            "Residue Graph Matrix" <- w533
            n321 = Bundle By Name(cluster=w526, "RI results"=w554, "Baes data type definition"=w553) -> (w555:T15)
            n322 = Array Max & Min(array=w533) -> (min index (indices)=w545:i32[])  [unwired: 3 out]
            n323 = call <vilib>:"create_plot_surface.vi"("z matrix"=w533, "y vector"=w531, "x vector"=w530) -> ("plots out"=→"3D Graph":refnum<class "Base Datatype.lvclass">[])  [unwired: 2 in, 6 out]
            n324 = local read "Diameter Factor or Offset"() -> (w537:bool)
            n325 = Index Array(array=w545, index #1=0 ("index"), index #2=1 ("index")) -> (element #1=w541:i32, element #2=w542:i32)
            n326 = Index Array(array=w531, index=w542) -> (element=w540:dbl)
            n327 = Index Array(array=w530, index=w541) -> (element=w536:dbl)
            n328 = local write "Extinction Factor"(w540) -> ()
            n329 = Select(t=1.0 ("Diameter Factor"), s=w537, f=w536) -> (s? t:f=w534:dbl)
            n330 = Select(t=w536, s=w537, f=0.0) -> (s? t:f=w535:dbl)
            n331 = local write "Diameter Factor"(w534) -> ()
            n332 = local write "Diameter Offset"(w535) -> ()
          }
          frame #1 {
          }
        }
        n333 = call <vilib>:"Add State(s) to Queue__jki_lib_state_machine.vi"("State(s) in Front (\"\")"="Load Files >> Dont Initialize Sizes\nRetrieve RI >> UseFactors\nUpdate Corrected multiple charge extinction graph" ("State(s) in Front (\"\")"), "State(s) in (\"\")"=w520) -> ("States Out"=w519:string)  [unwired: 13 in]
      }
      frame "Save RI to file" {
        n334 = stacked-sequence {
          tunnel: w644 -> [w697 _]
          frame #0 {
            n335 = local read "Approximate Errors"() -> (w662:bool)
            n336 = property on="Max Wavelength" class="CmbBox"() -> ("Value"=w673:string)  [unwired: 2 in, 2 out]
            n337 = property on="Min Wavelength" class="CmbBox"() -> ("Value"=w674:string)  [unwired: 2 in, 2 out]
            n338 = Unbundle By Name(w697) -> ("Extinction Cross section Path"=w705:path, "RI results.Wavelength"=w706:dbl[], "RI results.Real RI"=w707:dbl[], "RI results.Std Real RI"=w676:dbl[], "RI results.Imaginary RI"=w677:dbl[], "RI results.Std Imaginary RI"=w675:dbl[], "RI results.Residue"=w650:dbl[], "RI results.Extinction Factor"=w649:dbl[], "RI results.Diameter Factor"=w648:dbl[], "RI results.Diameter Offset"=w647:dbl[])
            n339 = local read "Calculate Errors"() -> (w663:bool)
            n340 = Decimal String To Number(string=w673) -> (number=w672:i32)  [unwired: 2 in, 1 out]
            n341 = Decimal String To Number(string=w674) -> (number=w652:i32)  [unwired: 2 in, 1 out]
            n342 = Unbundle By Name(w697) -> ("Extinction ExtinctionUncertainity Size parameter and Number ofS sizes"=w696:T5, "Particle Distribution Data"=w695:T6, "RI results"=w694:T14)
            n343 = Build Array(w706, w707, w677, w676, w675, w650, w649, w648, w647) -> (w704:dbl[][])
            n344 = Select(t="+ApproxError" ("name or relative path"), s=w662, f="-ApproxError" ("name or relative path")) -> (s? t:f=w661:string)
            n345 = Subtract(x=w672, y=w652) -> (x-y=w702:i32)
            n346 = call <vilib>:"Get File Extension.vi"("file"=w705) -> ("filename without extension"=w655:string)  [unwired: 7 in, 3 out]
            n347 = local read "Restrict to Positive Imaginary Part"() -> (w668:bool)
            n348 = Concatenate Strings(w655, w661) -> (w660:string)
            n349 = call "PrepareExtinctionCrossSectionToFile.vi"("Extinction ExtinctionUncertainity Size parameter and Number ofS sizes"=w696, "RI results"=w694, "Particle Distribution Data"=w695, "Min Wavelength index"=w652, "Max Wavelength index"=w672) -> ("Extinction"=w692:dbl[][], "CorrectedExtinction"=w693:dbl[][], "Sigma_diameter_string"=w682:string[])
            n350 = Transpose 2D Array(2D array=w704) -> (transposed array=w703:dbl[][])
            n351 = Increment(x=w702) -> (x+1=w651:i32)
            n352 = Select(t="+Error" ("name or relative path"), s=w663, f="-Error" ("name or relative path")) -> (s? t:f=w659:string)
            n353 = Concatenate Strings(w660, w659) -> (w658:string)
            n354 = Select(t="+Restricted" ("name or relative path"), s=w668, f="-Restricted" ("name or relative path")) -> (s? t:f=w657:string)
            n355 = Array Subset(array=w703, index (row)=w652, length (row)=w651) -> (w701:dbl[][])  [unwired: 2 in]
            n356 = Array Subset(array=w692, index (row)=w652, length (row)=w651) -> (w691:dbl[][])  [unwired: 2 in]
            n357 = Array Subset(array=w693, index (row)=w652, length (row)=w651) -> (w690:dbl[][])  [unwired: 2 in]
            n358 = Concatenate Strings(w658, w657) -> (w656:string)
            n359 = Transpose 2D Array(2D array=w691) -> (transposed array=w689:dbl[][])
            n360 = Transpose 2D Array(2D array=w690) -> (transposed array=w688:dbl[][])
            n361 = Number To Fractional String(number=w701, precision (6)=i16 3) -> (F-format string=w686:string[][])  [unwired: 2 in]
            n362 = Build Array (concatenate)(w689, w688) -> (w687:dbl[][])
            n363 = Concatenate Strings(w656, "_RIresult.txt" ("name or relative path")) -> (w708:string)
            n364 = Strip Path(path=w705) -> (stripped path=w709:path)  [unwired: 1 out]
            n365 = Number To Engineering String(4:w687) -> (0:w679:string[][])  [unwired: 3 in]
            n366 = Build Path(base path=w709, name or relative path=w708) -> (appended path=w698:path)
            "Saved RI to this filename and path" <- w698
            n367 = Transpose 2D Array(2D array=w679) -> (transposed array=w678:string[][])
            n368 = Build Array (concatenate)(string[] ["Wavelength (nm)", "Real Part", "Imaginary Part", "Conf Real Part", "Conf Imaginary part", "Residue (MDBF)", "Extinction Factor", "Diameter Factor", "Diameter Offset (nm)"] ("column headers"), w686) -> (w683:string[][])
            n369 = Build Array (concatenate)(w682, w678) -> (w681:string[][])
            n370 = Transpose 2D Array(2D array=w683) -> (transposed array=w685:string[][])
            n371 = Transpose 2D Array(2D array=w681) -> (transposed array=w680:string[][])
            n372 = Build Array (concatenate)(w685, w680) -> (w654:string[][])
            n373 = Transpose 2D Array(2D array=w654) -> (transposed array=w653:string[][])
            n374 = call-poly <vilib>:"Write To Spreadsheet File.vi"("transpose? (no:F)"=FALSE, "2D data"=w653, "file path (dialog if empty)"=w698) -> ()  [unwired: 5 in, 1 out]
          }
          frame #1 {
            n375 = One Button Dialog(message="File save was completed successfully") -> ()  [unwired: 1 in, 1 out]
          }
        }
        n376 = call <vilib>:"Add State(s) to Queue__jki_lib_state_machine.vi"("State(s) in (\"\")"=w646) -> ("States Out"=w645:string)  [unwired: 14 in]
      }
      frame "Save RI to File Expanded Edition" {
        n377 = stacked-sequence {
          tunnel: w712 -> [w771 _]
          frame #0 {
            # "This inlcudes the number of sizes and the reduced chi^2 measurement for each wavelength"
            n378 = Unbundle By Name(w771) -> ("Extinction Cross section Path"=w779:path, "RI results.Wavelength"=w780:dbl[], "RI results.Real RI"=w781:dbl[], "RI results.Std Real RI"=w749:dbl[], "RI results.Imaginary RI"=w750:dbl[], "RI results.Std Imaginary RI"=w748:dbl[], "RI results.Residue"=w720:dbl[], "Extinction ExtinctionUncertainity Size parameter and Number ofS sizes.Number ofSizes"=w719:dbl)
            n379 = Build Array(w780, w781, w750, w749, w748, w720) -> (w778:dbl[][])
            n380 = Transpose 2D Array(2D array=w778) -> (transposed array=w777:dbl[][])
            n381 = property on="Min Wavelength" class="CmbBox"() -> ("Value"=w747:string)  [unwired: 2 in, 2 out]
            n382 = property on="Max Wavelength" class="CmbBox"() -> ("Value"=w746:string)  [unwired: 2 in, 2 out]
            n383 = Decimal String To Number(string=w746) -> (number=w744:i32)  [unwired: 2 in, 1 out]
            n384 = Decimal String To Number(string=w747) -> (number=w745:i32)  [unwired: 2 in, 1 out]
            n385 = Unbundle By Name(w771) -> ("Extinction ExtinctionUncertainity Size parameter and Number ofS sizes"=w770:T5, "Particle Distribution Data"=w769:T6, "RI results"=w768:T14)
            n386 = Subtract(x=w744, y=w745) -> (x-y=w776:i32)
            n387 = call "PrepareExtinctionCrossSectionToFile.vi"("Extinction ExtinctionUncertainity Size parameter and Number ofS sizes"=w770, "RI results"=w768, "Particle Distribution Data"=w769, "Min Wavelength index"=w745, "Max Wavelength index"=w744) -> ("Extinction"=w765:dbl[][], "CorrectedExtinction"=w767:dbl[][], "Sigma_diameter_string"=w755:string[])
            n388 = Increment(x=w776) -> (x+1=w766:i32)
            n389 = Array Subset(array=w777, index (row)=w745, length (row)=w766) -> (w775:dbl[][])  [unwired: 2 in]
            n390 = Array Subset(array=w765, index (row)=w745, length (row)=w766) -> (w764:dbl[][])  [unwired: 2 in]
            n391 = Array Subset(array=w767, index (row)=w745, length (row)=w766) -> (w763:dbl[][])  [unwired: 2 in]
            n392 = Transpose 2D Array(2D array=w764) -> (transposed array=w762:dbl[][])
            n393 = Transpose 2D Array(2D array=w763) -> (transposed array=w761:dbl[][])
            n394 = Number To Fractional String(number=w775, precision (6)=i16 3) -> (F-format string=w759:string[][])  [unwired: 2 in]
            n395 = Build Array (concatenate)(w762, w761) -> (w760:dbl[][])
            n396 = Number To Engineering String(4:w760) -> (0:w752:string[][])  [unwired: 3 in]
            n397 = Transpose 2D Array(2D array=w752) -> (transposed array=w751:string[][])
            n398 = local read "Calculate Errors"() -> (w735:bool)
            n399 = Build Array (concatenate)(string[] ["Wavelength (nm)", "Real Part", "Imaginary Part", "Conf Real Part", "Conf Imaginary part", "Eta (reduced Chi^2)"] ("column headers"), w759) -> (w756:string[][])
            n400 = Build Array (concatenate)(w755, w751) -> (w754:string[][])
            n401 = local read "Approximate Errors"() -> (w734:bool)
            n402 = Transpose 2D Array(2D array=w756) -> (transposed array=w758:string[][])
            n403 = Transpose 2D Array(2D array=w754) -> (transposed array=w753:string[][])
            n404 = local read "Restrict to Positive Imaginary Part"() -> (w740:bool)
            n405 = Select(t="+ApproxError" ("name or relative path"), s=w734, f="-ApproxError" ("name or relative path")) -> (s? t:f=w733:string)
            n406 = Build Array (concatenate)(w758, w753) -> (w722:string[][])
            n407 = Select(t="+Error" ("name or relative path"), s=w735, f="-Error" ("name or relative path")) -> (s? t:f=w731:string)
            n408 = call <vilib>:"Get File Extension.vi"("file"=w779) -> ("filename without extension"=w718:string)  [unwired: 7 in, 3 out]
            n409 = Number To Decimal String(number=w719) -> (decimal integer string=w717:string)  [unwired: 1 in]
            n410 = Concatenate Strings(w718, w733) -> (w732:string)
            n411 = Array Size(array=w722) -> (size(s)=w727:i32[])
            n412 = Concatenate Strings(w718, "_" ("element"), w717) -> (w715:string)
            n413 = Select(t="+Restricted" ("name or relative path"), s=w740, f="-Restricted" ("name or relative path")) -> (s? t:f=w729:string)
            n414 = Concatenate Strings(w732, w731) -> (w730:string)
            n415 = Index Array(array=w727, index=0) -> (element=w725:i32)
            n416 = for {
              N: w725 -> [_]
              tunnel: [w785] -> w724 mode=indexing
              tunnel: w715 -> [w786]
              i -> [w788]
              n417 = Equal To 0?(x=w788) -> (x = 0?=w787:bool)
              n418 = Select(t=w786, s=w787, f="") -> (s? t:f=w785:string)
            }
            n419 = Concatenate Strings(w730, w729) -> (w728:string)
            n420 = Concatenate Strings(w728, "-RIresult.txt" ("name or relative path")) -> (w782:string)
            n421 = Strip Path(path=w779) -> (stripped path=w783:path)  [unwired: 1 out]
            n422 = Build Path(base path=w783, name or relative path=w782) -> (appended path=w772:path)
            "Saved RI to this filename and path 2" <- w772
            n423 = Transpose 2D Array(2D array=w722) -> (transposed array=w721:string[][])
            n424 = Build Array (concatenate)(w724, w721) -> (w723:string[][])
            n425 = call-poly <vilib>:"Write To Spreadsheet File.vi"("transpose? (no:F)"=FALSE, "2D data"=w723, "file path (dialog if empty)"=w772) -> ()  [unwired: 5 in, 1 out]
          }
          frame #1 {
            n426 = One Button Dialog(message="File save was completed successfully") -> ()  [unwired: 1 in, 1 out]
          }
        }
        n427 = call <vilib>:"Add State(s) to Queue__jki_lib_state_machine.vi"("State(s) in (\"\")"=w714) -> ("States Out"=w713:string)  [unwired: 14 in]
      }
      frame "Save RI -Monte Carlo to file" {
        n428 = stacked-sequence {
          tunnel: w791 -> [w811 _]
          frame #0 {
            n429 = Unbundle By Name(w811) -> ("Extinction Cross section Path"=w801:path, "RI MC results.Wavelength"=w802:dbl[], "RI MC results.Real RI"=w806:dbl[], "RI MC results.Std Real RI"=w805:dbl[], "RI MC results.Imaginary RI"=w804:dbl[], "RI MC results.Std Imaginary RI"=w803:dbl[])
            n430 = Build Array(w802, w806, w805, w804, w803) -> (w800:dbl[][])
            n431 = call <vilib>:"Get File Extension.vi"("file"=w801) -> ("filename without extension"=w809:string)  [unwired: 7 in, 3 out]
            n432 = Transpose 2D Array(2D array=w800) -> (transposed array=w795:dbl[][])
            n433 = Concatenate Strings(w809, "-RI-MC-result.xls" ("name or relative path")) -> (w807:string)
            n434 = Strip Path(path=w801) -> (stripped path=w810:path)  [unwired: 1 out]
            n435 = Number To Fractional String(number=w795, precision (6)=i16 3) -> (F-format string=w796:string[][])  [unwired: 2 in]
            n436 = Build Array (concatenate)(string[] ["Wavelength (nm)", "Real Part (MC)", "Std Real Part (MC)", "Imaginary Part  (MC)", "Std Imaginary part (MC)"] ("column headers"), w796) -> (w798:string[][])
            n437 = Build Path(base path=w810, name or relative path=w807) -> (appended path=w797:path)
            "Saved RI (MC) to this filename and path" <- w797
            n438 = call-poly <vilib>:"Write To Spreadsheet File.vi"("2D data"=w798, "file path (dialog if empty)"=w797) -> ()  [unwired: 6 in, 1 out]
          }
          frame #1 {
            n439 = One Button Dialog(message="File save was completed successfully") -> ()  [unwired: 1 in, 1 out]
          }
        }
        n440 = call <vilib>:"Add State(s) to Queue__jki_lib_state_machine.vi"("State(s) in (\"\")"=w793) -> ("States Out"=w792:string)  [unwired: 14 in]
      }
      frame "Retrieve RI Monte Carlo" {
        w836 = T14 {"Real RI"=[], "Imaginary RI"=[], "Std Imaginary RI"=[], "Std Real RI"=[], "Wavelength"=[], "Residue"=[], "Extinction Factor"=[], "Diameter Factor"=[], "Diameter Offset"=[], "Best fit result"=[], "Normalized Residuals"=[]}  # RI MC results
        n441 = call <vilib>:"Add State(s) to Queue__jki_lib_state_machine.vi"("State(s) in (\"\")"=w863) -> ("States Out"=w862:string)  [unwired: 14 in]
        n442 = property on="Min Wavelength" class="CmbBox"() -> ("Value"=w820:string)  [unwired: 2 in, 2 out]
        n443 = property on="Max Wavelength" class="CmbBox"() -> ("Value"=w818:string)  [unwired: 2 in, 2 out]
        n444 = Decimal String To Number(string=w820) -> (number=w819:i32)  [unwired: 2 in, 1 out]
        n445 = Decimal String To Number(string=w818) -> (number=w817:i32)  [unwired: 2 in, 1 out]
        n446 = Unbundle By Name(w835) -> ("Extinction ExtinctionUncertainity Size parameter and Number ofS sizes"=w857:T5, "Particle Distribution Data"=w860:T6)
        n447 = local read "General Data for RI Retrieval VI"() -> (w813:T3)
        n448 = local read "Size Parameter Factor"() -> (w815:bool)
        n449 = local read "Size Parameter Offset"() -> (w814:bool)
        n450 = local read "Extinction Factor"() -> (w816:bool)
        n451 = Bundle(cluster=w813, "Min WaveLength Index"=w819, "Max WaveLength Index"=w817, "Extinction Factor"=w816, "Size Parameter Factor"=w815, "Size Paramter Offset"=w814) -> (w827:T3)  [unwired: 4 in]
        n452 = Unbundle By Name(w857) -> ("Extinction"=w859:dbl[][], "Extinction Uncertainty"=w858:dbl[][])
        n453 = local read "Restrict to Positive Imaginary Part"() -> (w821:bool)
        n454 = local read "Size of statistics"() -> (w837:i32)
        n455 = local read "Size of statistics"() -> (w825:i32)
        n456 = control-ref of="MC progress"() -> (w826:refnum<vi>)
        n457 = Tick Count (ms)() -> (millisecond timer value=w838:u32)
        n458 = property class="Slide (strict)"(reference=w826, "Scale.Maximum"=w825) -> ()  [unwired: 1 in, 2 out]
        n459 = for {
          N: w837 -> [_]
          tunnel: w860 -> [w898]
          tunnel: w859 -> [w895]
          tunnel: w858 -> [w894]
          tunnel: w857 -> [w892]
          tunnel: [w887] -> w856 mode=indexing
          tunnel: [w883] -> w845 mode=indexing
          tunnel: [w882] -> w829
          tunnel: w837 -> [w877]
          shift-right: [w874] -> _
          shift-left: w838 -> [w881]
          tunnel: w827 -> [w873]
          tunnel: w826 -> [w872]
          tunnel: [w870] -> w824
          tunnel: w821 -> [w866]
          i -> [w871]
          n460 = for {
            tunnel: w895 -> [w904] mode=indexing
            tunnel: w894 -> [w903] mode=indexing
            tunnel: [w902] -> w893 mode=indexing
            n461 = for {
              tunnel: w904 -> [w912] mode=indexing
              tunnel: w903 -> [w910] mode=indexing
              tunnel: [w905] -> w902 mode=indexing
              w909 = 1000000000.0 ("y")
              n462 = Multiply(x=w912, y=w909) -> (x*y=w911:dbl)
              n463 = Multiply(x=w910, y=w909) -> (x*y=w908:dbl)
              n464 = Random Number (0-1)() -> (number: 0 to 1=w913:dbl)
              n465 = call-poly <vilib>:"Continuous Inverse CDF.vi"("std"=w908, "mean"=w911, "cdf(x)"=w913) -> ("x"=w907:dbl)  [unwired: 7 in, 1 out]
              n466 = Multiply(x=w907, y=1e-09) -> (x*y=w905:dbl)
            }
          }
          n467 = Tick Count (ms)() -> (millisecond timer value=w874:u32)
          n468 = Subtract(x=w874, y=w881) -> (x-y=w880:u32)
          n469 = Increment(x=w871) -> (x+1=w870:i32)
          n470 = property class="Slide (strict)"(reference=w872, "Value"=w870) -> ()  [unwired: 1 in, 2 out]
          n471 = Divide(x=w880, y=u32 60000) -> (x/y=w878:dbl)
          n472 = Subtract(x=w877, y=w871) -> (x-y=w876:i32)
          n473 = Multiply(x=w878, y=w876) -> (x*y=→"Time Left (min) (MC)":dbl)
          n474 = control-ref of="Simplex"() -> (w865:refnum<vi>)
          n475 = control-ref of="Real Part vs wavelength"() -> (w901:refnum<vi>)
          n476 = control-ref of="Not Corrected for Multiple charge Best fit result"() -> (w899:refnum<vi>)
          n477 = control-ref of="Imaginary Part vs wavelength"() -> (w900:refnum<vi>)
          n478 = control-ref of="Normalized Residuals vs Size parameter"() -> (w897:refnum<vi>)
          n479 = local read "Minimization method"() -> (w869:u16)
          n480 = local read "Calculate Errors"() -> (w867:bool)
          n481 = Bundle By Name(cluster=w892, "Extinction"=w893) -> (w891:T5)
          n482 = Bundle("Real Part vs wavelength"=w901, "Imaginary Part vs wavelength"=w900, "Normalized Residuals vs Size parameter"=w897, "Not Corrected for Multiple charge Best fit result"=w899, "Simplex"=w865) -> (w896:T22)  [unwired: 1 in]
          n483 = call "RIRetrieval.vi"("General Data for RI Retrieval VI"=w873, "Approximate Errors"="Approximate Errors", "Restrict to Positive Imaginary Part"=w866, "Extinction Measured Data"=w891, "Calculate Errors"=w867, "Particle Distribution Data"=w898, "Graph Refs"=w896, "Minimization method"=w869) -> ("Imaginary Part vs wavelength"=w884:cluster{dbl[], dbl[]}[], "Real Part vs wavelength"=w890:cluster{dbl[], dbl[]}[])  [unwired: 2 out]
          n484 = Index Array(array=w890, index=0) -> (element=w888:cluster{dbl[], dbl[]})
          n485 = Index Array(array=w884, index=0) -> (element=w885:cluster{dbl[], dbl[]})
          n486 = Unbundle(w885) -> (w883:dbl[])  [unwired: 1 out]
          n487 = Unbundle(w888) -> (w882:dbl[], w887:dbl[])
          "Loop index (MC)" <- w871
        }
        n488 = call <vilib>:"Covariance Matrix.vi"("X"=w856) -> ("mean vector"=w828:dbl[], "covariance matrix V"=w855:T23)  [unwired: 9 in]
        n489 = call <vilib>:"Covariance Matrix.vi"("X"=w845) -> ("mean vector"=w832:dbl[], "covariance matrix V"=w850:T23)  [unwired: 9 in]
        n490 = Greater?(x=w824, y=0) -> (0:w822:bool)
        n491 = case shown="True" w822 {
          frame False {
          }
          frame True {
            n492 = One Button Dialog(message="MC run finished successfully") -> ()  [unwired: 1 in, 1 out]
          }
        }
        n493 = Index Array(array=w855) -> (element=w854:T23)  [unwired: 2 in]
        n494 = Index Array(array=w850) -> (element=w849:T23)  [unwired: 2 in]
        n495 = call-poly <vilib>:"Matrix To Array.vi"("Real Matrix"=w854) -> ("Real 2D Array"=w853:dbl[][])
        n496 = call-poly <vilib>:"Matrix To Array.vi"("Real Matrix"=w849) -> ("Real 2D Array"=w848:dbl[][])
        n497 = Index Array(array=w853, index (col)=0 ("disabled index (col)")) -> (element=w851:dbl[])  [unwired: 1 in]
        n498 = Index Array(array=w848, index (col)=0 ("disabled index (col)")) -> (element=w846:dbl[])  [unwired: 1 in]
        n499 = Bundle(w829, "mean vector"=w828) -> (w844:cluster{dbl[], "mean vector":dbl[]})  [unwired: 1 in]
        n500 = Square Root(x=w851) -> (sqrt(x)=w830:dbl[])
        n501 = Bundle(w829, "mean vector"=w832) -> (w841:cluster{dbl[], "mean vector":dbl[]})  [unwired: 1 in]
        n502 = Square Root(x=w846) -> (sqrt(x)=w831:dbl[])
        n503 = call "XY error bars.vi"("XY plot"=w844, "Yerror"=w830) -> ("Y error bars"=w843:cluster{dbl[], dbl[]})  [unwired: 6 in, 2 out]
        n504 = call "XY error bars.vi"("XY plot"=w841, "Yerror"=w831) -> ("Y error bars"=w840:cluster{dbl[], dbl[]})  [unwired: 6 in, 2 out]
        n505 = Bundle By Name(cluster=w836, "Real RI"=w828, "Imaginary RI"=w832, "Std Imaginary RI"=w831, "Std Real RI"=w830, "Wavelength"=w829) -> (w833:T14)
        n506 = Build Array(w844, w843) -> (→"Real Part MC":cluster{dbl[], "mean vector":dbl[]}[])
        n507 = Build Array(w841, w840) -> (→"Imaginary Part MC":cluster{dbl[], "mean vector":dbl[]}[])
        n508 = Bundle By Name(cluster=w835, "RI MC results"=w833) -> (w834:T15)
      }
      frame "Retreive RI from Single Measurements(MC)" {
        w941 = T14 {"Real RI"=[], "Imaginary RI"=[], "Std Imaginary RI"=[], "Std Real RI"=[], "Wavelength"=[], "Residue"=[], "Extinction Factor"=[], "Diameter Factor"=[], "Diameter Offset"=[], "Best fit result"=[], "Normalized Residuals"=[]}  # RI MC results
        n509 = call <vilib>:"Add State(s) to Queue__jki_lib_state_machine.vi"("State(s) in (\"\")"=w965) -> ("States Out"=w964:string)  [unwired: 14 in]
        n510 = property on="Min Wavelength" class="CmbBox"() -> ("Value"=w921:string)  [unwired: 2 in, 2 out]
        n511 = property on="Max Wavelength" class="CmbBox"() -> ("Value"=w920:string)  [unwired: 2 in, 2 out]
        n512 = Unbundle By Name(w940) -> ("Extinction ExtinctionUncertainity Size parameter and Number ofS sizes"=w959:T5, "Particle Distribution Data"=w962:T6, "FullExtinctionData"=w926:dbl[][], "NumberOfMeasurementsperSize"=w923:i32)
        n513 = Decimal String To Number(string=w921) -> (number=w918:i32)  [unwired: 2 in, 1 out]
        n514 = Decimal String To Number(string=w920) -> (number=w919:i32)  [unwired: 2 in, 1 out]
        n515 = local write "Size of statistics"(w923) -> ()
        n516 = local read "General Data for RI Retrieval VI"() -> (w914:T3)
        n517 = local read "Size Parameter Factor"() -> (w916:bool)
        n518 = local read "Size Parameter Offset"() -> (w915:bool)
        n519 = local read "Extinction Factor"() -> (w917:bool)
        n520 = Unbundle By Name(w959) -> ("Number ofSizes"=w961:dbl, "Extinction Uncertainty"=w960:dbl[][])
        n521 = Bundle(cluster=w914, "Min WaveLength Index"=w918, "Max WaveLength Index"=w919, "Extinction Factor"=w917, "Size Parameter Factor"=w916, "Size Paramter Offset"=w915) -> (w932:T3)  [unwired: 4 in]
        n522 = local read "Restrict to Positive Imaginary Part"() -> (w922:bool)
        n523 = local read "Size of statistics"() -> (w930:i32)
        n524 = control-ref of="MC progress"() -> (w931:refnum<vi>)
        n525 = Tick Count (ms)() -> (millisecond timer value=w942:u32)
        n526 = property class="Slide (strict)"(reference=w931, "Scale.Maximum"=w930) -> ()  [unwired: 1 in, 2 out]
        n527 = for {
          N: w923 -> [_]
          tunnel: w962 -> [w1002]
          tunnel: w961 -> [w974]
          tunnel: w960 -> [_]
          tunnel: w959 -> [w999]
          tunnel: [w994] -> w958 mode=indexing
          tunnel: [w990] -> w947 mode=indexing
          tunnel: [w989] -> w934
          tunnel: w923 -> [w984]
          shift-right: [w982] -> _
          shift-left: w942 -> [w988]
          tunnel: w932 -> [w968]
          tunnel: w931 -> [w981]
          tunnel: [w980] -> w929
          tunnel: w926 -> [w975]
          tunnel: w923 -> [w970]
          tunnel: w922 -> [w969]
          i -> [w973]
          n528 = Tick Count (ms)() -> (millisecond timer value=w982:u32)
          n529 = Subtract(x=w982, y=w988) -> (x-y=w987:u32)
          n530 = Increment(x=w973) -> (x+1=w972:i32)
          n531 = Increment(x=w973) -> (x+1=w980:i32)
          n532 = mathscript code="Extinction=[];\nfor j=0:(NumOfSizes-1)\nExtinction=[Extinction FullExt(:,j*NumOfMeas+i)];\ntemp=j*NumOfMeas+i;\nend\n%Extinction=Extinction';"("FullExt"=w975, "i"=w972, "NumOfSizes"=w974, "NumOfMeas"=w970) -> ("Extinction"=w971:dbl[][])  [unwired: 1 in, 1 out]
          n533 = property class="Slide (strict)"(reference=w981, "Value"=w980) -> ()  [unwired: 1 in, 2 out]
          n534 = Divide(x=w987, y=u32 60000) -> (x/y=w985:dbl)
          n535 = Bundle By Name(cluster=w999, "Extinction"=w971) -> (w998:T5)
          n536 = Subtract(x=w984, y=w973) -> (x-y=w983:i32)
          n537 = control-ref of="Simplex"() -> (w967:refnum<vi>)
          n538 = Multiply(x=w985, y=w983) -> (x*y=w977:dbl)
          n539 = control-ref of="Real Part vs wavelength"() -> (w1005:refnum<vi>)
          n540 = control-ref of="Not Corrected for Multiple charge Best fit result"() -> (w1003:refnum<vi>)
          n541 = control-ref of="Imaginary Part vs wavelength"() -> (w1004:refnum<vi>)
          n542 = control-ref of="Normalized Residuals vs Size parameter"() -> (w1001:refnum<vi>)
          n543 = local write "Time Left (min) (MC)"(w977) -> ()
          n544 = local read "Minimization method"() -> (w979:u16)
          n545 = local read "Approximate Errors"() -> (w976:bool)
          n546 = local read "Calculate Errors"() -> (w978:bool)
          n547 = Bundle("Real Part vs wavelength"=w1005, "Imaginary Part vs wavelength"=w1004, "Normalized Residuals vs Size parameter"=w1001, "Not Corrected for Multiple charge Best fit result"=w1003, "Simplex"=w967) -> (w1000:T22)  [unwired: 1 in]
          n548 = call "RIRetrieval.vi"("General Data for RI Retrieval VI"=w968, "Approximate Errors"=w976, "Restrict to Positive Imaginary Part"=w969, "Extinction Measured Data"=w998, "Calculate Errors"=w978, "Particle Distribution Data"=w1002, "Graph Refs"=w1000, "Minimization method"=w979) -> ("Imaginary Part vs wavelength"=w991:cluster{dbl[], dbl[]}[], "Real Part vs wavelength"=w997:cluster{dbl[], dbl[]}[])  [unwired: 2 out]
          n549 = Index Array(array=w997, index=0) -> (element=w995:cluster{dbl[], dbl[]})
          n550 = Index Array(array=w991, index=0) -> (element=w992:cluster{dbl[], dbl[]})
          n551 = Unbundle(w995) -> (w989:dbl[], w994:dbl[])
          n552 = Unbundle(w992) -> (w990:dbl[])  [unwired: 1 out]
          "Loop index (MC) 2" <- w973
        }
        n553 = call <vilib>:"Covariance Matrix.vi"("X"=w958) -> ("mean vector"=w933:dbl[], "covariance matrix V"=w957:T23)  [unwired: 9 in]
        n554 = call <vilib>:"Covariance Matrix.vi"("X"=w947) -> ("mean vector"=w937:dbl[], "covariance matrix V"=w952:T23)  [unwired: 9 in]
        n555 = Greater?(x=w929, y=0) -> (0:w927:bool)
        n556 = case shown="True" w927 {
          frame False {
          }
          frame True {
            n557 = One Button Dialog(message="MC run finished successfully") -> ()  [unwired: 1 in, 1 out]
          }
        }
        n558 = Index Array(array=w957) -> (element=w956:T23)  [unwired: 2 in]
        n559 = Index Array(array=w952) -> (element=w951:T23)  [unwired: 2 in]
        n560 = call-poly <vilib>:"Matrix To Array.vi"("Real Matrix"=w956) -> ("Real 2D Array"=w955:dbl[][])
        n561 = call-poly <vilib>:"Matrix To Array.vi"("Real Matrix"=w951) -> ("Real 2D Array"=w950:dbl[][])
        n562 = Index Array(array=w955, index (col)=0 ("disabled index (col)")) -> (element=w953:dbl[])  [unwired: 1 in]
        n563 = Index Array(array=w950, index (col)=0 ("disabled index (col)")) -> (element=w948:dbl[])  [unwired: 1 in]
        n564 = Bundle(w934, "mean vector"=w933) -> (w946:cluster{dbl[], "mean vector":dbl[]})  [unwired: 1 in]
        n565 = Square Root(x=w953) -> (sqrt(x)=w935:dbl[])
        n566 = Bundle(w934, "mean vector"=w937) -> (w944:cluster{dbl[], "mean vector":dbl[]})  [unwired: 1 in]
        n567 = Square Root(x=w948) -> (sqrt(x)=w936:dbl[])
        n568 = call "XY error bars.vi"("XY plot"=w946, "Yerror"=w935) -> ("Y error bars"=w945:cluster{dbl[], dbl[]})  [unwired: 6 in, 2 out]
        n569 = call "XY error bars.vi"("XY plot"=w944, "Yerror"=w936) -> ("Y error bars"=w943:cluster{dbl[], dbl[]})  [unwired: 6 in, 2 out]
        n570 = Bundle By Name(cluster=w941, "Real RI"=w933, "Imaginary RI"=w937, "Std Imaginary RI"=w936, "Std Real RI"=w935, "Wavelength"=w934) -> (w938:T14)
        n571 = Build Array(w946, w945) -> (w925:cluster{dbl[], "mean vector":dbl[]}[])
        n572 = Build Array(w944, w943) -> (w924:cluster{dbl[], "mean vector":dbl[]}[])
        n573 = local write "Real Part MC"(w925) -> ()
        n574 = local write "Imaginary Part MC"(w924) -> ()
        n575 = Bundle By Name(cluster=w940, "RI MC results"=w938) -> (w939:T15)
      }
      frame "Update Window after Load Files" {
        n576 = Unbundle By Name(w1114) -> ("Extinction ExtinctionUncertainity Size parameter and Number ofS sizes.WaveLength"=w1113:dbl[])
        n577 = call <vilib>:"Add State(s) to Queue__jki_lib_state_machine.vi"("State(s) in (\"\")"=w1117) -> ("States Out"=w1116:string)  [unwired: 14 in]
        n578 = for {
          tunnel: w1113 -> [w1129] mode=indexing
          tunnel: [w1130] -> w1112 mode=indexing
          tunnel: [w1128] -> w1111 mode=indexing
          i -> [w1128]
          n579 = Number To Decimal String(number=w1128) -> (decimal integer string=w1127:string)  [unwired: 1 in]
          n580 = Number To Fractional String(number=w1129, precision (6)=i16 3) -> (F-format string=w1126:string)  [unwired: 2 in]
          n581 = Bundle(w1126, w1127) -> (w1130:cluster{string, string})  [unwired: 1 in]
        }
        n582 = flat-sequence {
          tunnel: w1112 -> [w1119]
          tunnel: w1112 -> [w1118]
          tunnel: w1111 -> [w1124]
          frame #0 {
            n583 = property on="Max Wavelength" class="CmbBox"("Strings And Values[]"=w1119) -> ()  [unwired: 2 in, 2 out]
            n584 = property on="Min Wavelength" class="CmbBox"("Strings And Values[]"=w1118) -> ()  [unwired: 2 in, 2 out]
          }
          frame #1 {
            n585 = Array Max & Min(array=w1124) -> (max value=w1120:i32, min value=w1123:i32)  [unwired: 2 out]
            n586 = Number To Decimal String(number=w1120) -> (decimal integer string=w1122:string)  [unwired: 1 in]
            n587 = Number To Decimal String(number=w1123) -> (decimal integer string=w1121:string)  [unwired: 1 in]
            n588 = property on="Max Wavelength" class="CmbBox"("Value"=w1122) -> ()  [unwired: 2 in, 2 out]
            n589 = property on="Min Wavelength" class="CmbBox"("Value"=w1121) -> ()  [unwired: 2 in, 2 out]
          }
        }
      }
      frame "Update Corrected multiple charge extinction graph" {
        w1134 = i16 3 ("precision (6)")
        n590 = call <vilib>:"Add State(s) to Queue__jki_lib_state_machine.vi"("State(s) in (\"\")"=w1195) -> ("States Out"=w1194:string)  [unwired: 14 in]
        n591 = control-ref of="Imaginary Part vs wavelength"() -> (w1190:refnum<vi>)
        n592 = Unbundle By Name(w1153) -> ("Baes data type definition"=w1175:T8, "Extinction ExtinctionUncertainity Size parameter and Number ofS sizes.WaveLength"=w1189:dbl[], "Extinction ExtinctionUncertainity Size parameter and Number ofS sizes.Extinction"=w1178:dbl[][], "Extinction ExtinctionUncertainity Size parameter and Number ofS sizes.Extinction Uncertainty"=w1179:dbl[][], "Extinction ExtinctionUncertainity Size parameter and Number ofS sizes.Size parameters"=w1181:dbl[][], "Extinction ExtinctionUncertainity Size parameter and Number ofS sizes.Number ofSizes"=w1182:dbl, "Extinction ExtinctionUncertainity Size parameter and Number ofS sizes.GeometricCrossSection"=w1183:dbl[], "Extinction ExtinctionUncertainity Size parameter and Number ofS sizes.WaveLength"=w1185:dbl[], "Particle Distribution Data.SMPS Sizes"=w1186:dbl[], "Particle Distribution Data.Concentration"=w1187:dbl[][], "Particle Distribution Data.Double Charge Correction Flag"=w1188:bool, "RI results.Extinction Factor"=w1171:dbl[], "RI results.Diameter Factor"=w1167:dbl[], "RI results.Diameter Offset"=w1166:dbl[], "RI results.Residue"=w1169:dbl[], "RI results.Real RI"=w1162:dbl[], "RI results.Std Real RI"=w1161:dbl[], "RI results.Imaginary RI"=w1160:dbl[], "RI results.Std Imaginary RI"=w1159:dbl[], "RI results.Best fit result"=w1158:dbl[][], "RI results.Normalized Residuals"=w1157:dbl[][])  [unwired: 1 out]
        n593 = property on="Property Node" class="XYGraph (strict)"(reference=w1190) -> ("Cursor.Cursor X"=w1133:dbl)  [unwired: 1 in, 2 out]
        "Wavelength" <- w1133
        n594 = Search 1D Array(1D array=w1189, element=w1133) -> (index of element=w1156:i32)  [unwired: 1 in]
        "index of element" <- w1156
        n595 = Index Array(array=w1185, index=w1156) -> (element=w1184:dbl)
        n596 = Index Array(array=w1169, index=w1156) -> (element=→"Residue (MDBF)":dbl)
        n597 = Index Array(array=w1178, index (row)=w1156) -> (element=w1177:dbl[])  [unwired: 1 in]
        n598 = Index Array(array=w1179, index (row)=w1156) -> (element=w1176:dbl[])  [unwired: 1 in]
        n599 = Index Array(array=w1181, index (row)=w1156) -> (element=w1180:dbl[])  [unwired: 1 in]
        n600 = Index Array(array=w1171, index=w1156) -> (element=w1168:dbl)
        "Extinction Factor" <- w1168
        n601 = Index Array(array=w1167, index=w1156) -> (element=w1164:dbl)
        "Diameter Factor" <- w1164
        n602 = Index Array(array=w1166, index=w1156) -> (element=w1163:dbl)
        "Diameter Offset" <- w1163
        n603 = Index Array(array=w1162, index=w1156) -> (element=w1150:dbl)
        "Real part" <- w1150
        n604 = Index Array(array=w1161, index=w1156) -> (element=w1149:dbl)
        "Real Uncertainty" <- w1149
        n605 = Index Array(array=w1159, index=w1156) -> (element=w1137:dbl)
        "Imaginary Uncertainty" <- w1137
        n606 = Index Array(array=w1160, index=w1156) -> (element=w1138:dbl)
        "Imaginary Part" <- w1138
        n607 = Index Array(array=w1158, index (row)=w1156) -> (element=w1155:dbl[])  [unwired: 1 in]
        n608 = Index Array(array=w1157, index (row)=w1156) -> (element=w1154:dbl[])  [unwired: 1 in]
        n609 = Less Than 0?(x=w1156) -> (x < 0?=w1172:bool)
        n610 = Number To Fractional String(number=w1150, precision (6)=w1134) -> (F-format string=w1148:string)  [unwired: 2 in]
        n611 = Number To Fractional String(number=w1133, precision (6)=w1134) -> (F-format string=w1132:string)  [unwired: 2 in]
        n612 = Number To Fractional String(number=w1149, precision (6)=w1134) -> (F-format string=w1146:string)  [unwired: 2 in]
        n613 = Number To Fractional String(number=w1138, precision (6)=w1134) -> (F-format string=w1143:string)  [unwired: 2 in]
        n614 = Number To Fractional String(number=w1137, precision (6)=w1134) -> (F-format string=w1141:string)  [unwired: 2 in]
        n615 = Concatenate Strings("WL=" ("string"), w1132, "nm" ("string")) -> (→"Wavelength":string)
        n616 = Concatenate Strings("n=" ("string"), w1148, "±" ("element"), w1146) -> (→"Real Part":string)
        n617 = Concatenate Strings("k=" ("string"), w1143, "±" ("element"), w1141) -> (→"Imaginary Part":string)
        n618 = Bundle By Name(cluster=w1175, "Extinction"=w1177, "Extinction Uncertainty"=w1176, "Size parameters"=w1180, "Number ofSizes"=w1182, "GeometricCrossSection"=w1183, "Wave Length"=w1184, "SMPS Sizes"=w1186, "Concentration"=w1187, "Double Charge Correction"=w1188, "Extincation Factor"=w1168) -> (w1151:T8)
        n619 = in-place {
          in-place-border: w1164 -> [w1203]
          in-place-border: w1163 -> [w1201]
          n620 = in-place-cluster #1(w1151) -> ("Size parameters"=w1207:dbl[], "Wave Length"=w1197:dbl)
          n621 = Multiply(x=w1207, y=w1197) -> (x*y=w1206:dbl[])
          n622 = Divide(x=w1206, y=3.141592653589793) -> (x/y=w1204:dbl[])
          n623 = Multiply(x=w1204, y=w1203) -> (x*y=w1202:dbl[])
          n624 = Add(x=w1202, y=w1201) -> (x+y=w1200:dbl[])
          n625 = Multiply(x=w1200, y=3.141592653589793) -> (x*y=w1198:dbl[])
          n626 = Divide(x=w1198, y=w1197) -> (x/y=w1196:dbl[])
          n627 = in-place-cluster #1("Size parameters"=w1196, "Wave Length"=w1197) -> (w1165:T8)
        }
        n628 = Bundle By Name(cluster=w1153, "Baes data type definition"=w1151) -> (w1152:T15)
        n629 = control-ref of="Real Part vs wavelength"() -> (w1192:refnum<vi>)
        n630 = control-ref of="Imaginary Part vs wavelength"() -> (w1191:refnum<vi>)
        n631 = property on="Property Node" class="XYGraph (strict)"(reference=w1192) -> ("Cursor.Cursor Y"=w1174:dbl)  [unwired: 1 in, 2 out]
        n632 = property on="Property Node" class="XYGraph (strict)"(reference=w1191) -> ("Cursor.Cursor Y"=w1173:dbl)  [unwired: 1 in, 2 out]
        n633 = case shown="False" w1172 {
          tunnel: w1165 -> [w1225 _]
          tunnel: w1174 -> [w1221 _]
          tunnel: w1173 -> [w1220 _]
          tunnel: w1151 -> [w1222 _]
          tunnel: w1155 -> [w1235 _]
          tunnel: w1154 -> [w1231 _]
          frame False {
            # "Calculate Residue (CDMRI)"
            # "Update Measured graph as well"
            n634 = call "CalculateExpectedExtinctionIncludingDoublyChargeParticleCorrection.vi"("refractive index, imaginary"=w1220, "refractive index, real"=w1221, "Extinction ExtinctionUncertainity Size parameter and Number ofS sizes"=w1222) -> ("Expected Extinction Cross Section"=w1219:sgl[])  [unwired: 1 out]
            n635 = call "CalculateExtinctionCorrectionsToDoublyChargeParticleContribution.vi"("refractive index, imaginary"=w1220, "refractive index, real"=w1221, "Extinction ExtinctionUncertainity Size parameter and Number ofS sizes"=w1222) -> ("Expected Extinction graph"=→"Multiple charge correction term":cluster{"Size parameters":dbl[], dbl[]}, "Expected Extinction Cross Section"=w1218:sgl[])
            n636 = Subtract(x=w1219, y=w1218) -> (x-y=w1215:sgl[])
            n637 = Unbundle By Name(w1225) -> ("Extinction"=w1229:dbl[], "Size parameters"=w1217:dbl[], "Extinction Uncertainty"=w1212:dbl[], "Number ofSizes"=w1209:dbl)
            n638 = Subtract(x=w1229, y=w1218) -> (x-y=w1224:dbl[])
            n639 = call "CalculateAreaOfFirstPeakofSizeDistribution.vi"("Extinction ExtinctionUncertainity Size parameter and Number ofS sizes"=w1225) -> ("Area of First peak"=w1214:dbl[])
            n640 = Bundle("Size parameters"=w1217, "Extinction"=w1229) -> (w1245:T24)  [unwired: 1 in]
            n641 = Bundle("Size parameters"=w1217, "Extinction"=w1229) -> (w1237:T24)  [unwired: 1 in]
            n642 = Bundle("Size parameters"=w1217, "Normalized Residuals"=w1231) -> (w1233:T25)  [unwired: 1 in]
            n643 = Divide(x=w1215, y=w1214) -> (x/y=w1213:dbl[])
            n644 = Divide(x=w1224, y=w1214) -> (x/y=w1223:dbl[])
            n645 = call "PlotMieCurve.vi"("refractive index, imaginary"=w1220, "refractive index, real"=w1221, "Use Extinction Factor"=TRUE, "Extinction ExtinctionUncertainity Size parameter and Number ofS sizes"=w1225) -> ("Mie Results In Size Parameters"=w1230:sgl[], "Size parameters"=w1242:dbl[], "Extinction Crosssections"=w1243:dbl[])
            n646 = Bundle("Size parameters"=w1217, "Best fit result"=w1235) -> (w1234:T26)  [unwired: 1 in]
            n647 = Build Array(w1233) -> (w1232:T2)
            n648 = call "XY error bars.vi"("XY plot"=w1237, "Yerror"=w1212) -> ("Y error bars"=w1236:cluster{dbl[], dbl[]})  [unwired: 6 in, 2 out]
            n649 = Subtract(x=w1230, y=w1223) -> (x-y=w1228:dbl[])
            n650 = Bundle("Size parameters"=w1217, w1223) -> (w1240:cluster{"Size parameters":dbl[], dbl[]})  [unwired: 1 in]
            n651 = Build Array(w1237, w1236, w1234) -> (w1238:T27)
            n652 = property on="Normalized Residuals vs Size parameter" class="XYGraph (strict)"("Value"=w1232) -> ()  [unwired: 2 in, 2 out]
            n653 = Bundle("Size parameters"=w1217, w1213) -> (w1216:cluster{"Size parameters":dbl[], dbl[]})  [unwired: 1 in]
            n654 = Bundle("Size parameters"=w1242, "Extinction Crosssections"=w1243) -> (w1241:T20)  [unwired: 1 in]
            n655 = property on="Not Corrected for Multiple charge Best fit result" class="XYGraph (strict)"("Value"=w1238) -> ()  [unwired: 2 in, 2 out]
            n656 = call "XY error bars.vi"("XY plot"=w1240, "Yerror"=w1212) -> ("Y error bars"=w1239:cluster{dbl[], dbl[]})  [unwired: 6 in, 2 out]
            n657 = Build Array(w1240, w1245, w1241, w1239, w1216) -> (→"Corrected for multiple charge particles":T21)
            n658 = Divide(x=w1228, y=w1212) -> (x/y=w1227:dbl[])
            n659 = Square(x=w1227) -> (x^2=w1211:dbl[])
            n660 = Add Array Elements(numeric array=w1211) -> (sum=w1210:dbl)
            n661 = Divide(x=w1210, y=w1209) -> (x/y=→"Residue (CDMRI)":dbl)
          }
          frame True {
          }
        }
      }
    }
  }
